vi "MC_7_25_12a_JW.vi"() -> ()   [LabVIEW 2011]
uses:
  <vilib>/Utility/file.llb/Read From Spreadsheet File (string).vi
  <vilib>/Utility/inputDevices.llb/keyboardAcquire.vi
  <vilib>/Utility/file.llb/Write To Spreadsheet File (DBL).vi
  <vilib>/Utility/file.llb/Write To Spreadsheet File (string).vi
  <vilib>/regexp/Match Regular Expression.xnode
panel:
  in  "Room Temp":dbl=294.0
  out "No Image 2":path=path "\\\\acad1\\physics/Jurchescu-group/JW-PD/Image Not Found.png"
  out "Save1 Array":string[][](array[string])
  out "XY Graph-Lin":cluster{dbl[], dbl[]}[](graph)
  out "Lin Vd":dbl
  out "Lin-Vg Array-Used":dbl[](array[numeric])
  out "Lin Id-Used":dbl[](array[numeric])
  out "Comments":string
  out "Folder Index":dbl caption="Length"
  out "Current \nRecord":string[](array[string])
  out "Transformer \nHeaders":string[](array[string])
  out "Current Device ID":string
  out "Column":string
  out "Row":string
  out "Rec: Concentration":dbl
  out "Rec: Solvent":string
  out "Rec: Method":string
  in  "?":T1(tab)
  out "Rec: Material":string
  in  "Treatment Concentration (mM):":dbl=30.0
  in  "Surface Treatment:":string
  in  "# Drops*:":dbl=inf
  in  "Solution Temp (C):":dbl=55.0
  in  "Relative Humidity (%):":dbl=nan
  in  "Room Temp (F):":dbl=nan
  in  "Time (s):":dbl=80.0
  out "Accel (RPM/s):":dbl
  in  "RPM:":dbl=1000.0
  in  "Wait Time (s):":dbl=10.0
  in  "Sample #:":dbl=1.0
  in  "Fabricator:":string="Jeremy"
  in  "Data File":path
  out "Data Folder":path
  in  "Image Folder":path
  out "Image File":path=path "D:/UserData/Desktop/Jeremy/WFU/Research/Programs/VI mods/Image Not Found.png"
  in  "Ramp (s):":dbl=3.0
  out "Calc: Off I-Sat":dbl caption="Off I-Sat" format="%#_4e"
  in  "Manuel-Dielectric":bool
  in  "Manuel-Length":bool
  out "Calc: VT-Lin":dbl
  out "New: VT-Lin":dbl
  out "Rec: VT-Lin":dbl caption="VT-Lin" format="%#_3g"
  out "Calc: Trap Density-STS":dbl format="%#_3e"
  out "New: Trap Density-STS":dbl format="%#_3e"
  out "Rec: Trap Density-STS":dbl caption="N-Sat (STS)" format="%#_3e"
  out "Calc: Trap Density-VT":dbl format="%#_3e"
  out "New: Trap Density-VT":dbl format="%#_3e"
  out "Rec: Trap Density-VT":dbl caption="N-Sat (VT)" format="%#_3e"
  out "Calc: Mobility-Lin":dbl format="%#_4e"
  out "New: Mobility-Lin":dbl format="%#_4e"
  out "Rec: Mobility-Lin":dbl caption="Mobility-Lin" format="%#_4e"
  out "Calc: Mobility-Sat":dbl format="%#_4e"
  out "Rec: Length":dbl caption="Length" format="%#_3g"
  out "Rec: Width":dbl caption="Width" format="%#_4g"
  out "Rec: Dielectric (d)":dbl caption="Dielectric (d)" format="%#_3g"
  out "XY Graph":cluster{dbl[], dbl[]}[](graph)
  in  "NumPts":dbl=5.0
  in  "Cancel Button":bool
  in  "Next Button":bool
  in  "Previous Button":bool
  in  "Up Button":bool
  in  "Down Button":bool
  out "Data Name:":string
  in  "Save Changes?":bool
  in  "New: Dielectric":dbl
  in  "New: Length":dbl
  in  "New: Width":dbl
  out "New: Mobility-Sat":dbl format="%#_4e"
  in  "Slide":dbl(slide) step=1.0 scale=-14.3..89.0 scale format="%#_1p"
  in  "Blank Button":bool
  in  "Zoom":i16(slide)=-3 scale=-5.0..5.0
  out "Image Out 2":T2(plugin-control)
  out "Image Out":T2(plugin-control)
  in  "Magnification":u16(ring) items=["5x", "10x", "20x", "50x", "80x"]
  out "Total Width":dbl
  out "Distances":dbl[](array[numeric])
  in  "Undo Button":bool
  in  "Remove Button":bool
  out "Rec: Mobility-Sat":dbl caption="Mobility-Sat" format="%#_4e"
  out "Index":string
  out "Image Name":string
  in  "Export":bool
  out "Calc: VT-Sat":dbl format="%#_3g"
  out "New: VT-Sat":dbl format="%#_3g"
  in  "Manual-Width":bool caption="Manual"
  out "XY Graph 2":cluster{dbl[], dbl[]}[](graph)
  in  "Next Button 2":bool
  in  "Previous Button 2":bool
  in  "Slide 2":dbl(slide) step=1.0 scale=-1.0..82.0 scale format="%#_1p"
  out "Calc: STS":dbl format="%#_3g"
  out "New: STS":dbl format="%#_3g"
  in  "NumPts 2":dbl=5.0 caption="NumPts"
  out "Rec: VT-Sat":dbl caption="VT-Sat" format="%#_3g"
  out "Rec: STS":dbl caption="STS-Sat" format="%#_3g"
  out "Rec: On/Off":dbl caption="On/Off-Sat" format="%#_4e"
  in  "Save Changes? 2":bool
  in  "Save Changes? 3":bool
  out "Date Recorded":string="Date Recorded" caption="Measured"
  out "Date Created":string caption="Fabricated"
  out "Rec: Temp":dbl caption="Sample Temp"
  out "New: Temp":dbl
  out "Rec: Off I-Sat":dbl caption="Off I-Sat" format="%#_4e"
  out "String":string
  in  "No Image":path=path "\\\\acad1\\physics/Jurchescu-group/JW-PD/Image Not Found.png"
  in  "Project":path=path "\\\\acad1\\physics/Jurchescu-group/JW-PD/Group Library/Origin Project Files/DeviceData_7_25a_JWW.opj"
  out "Index 2":dbl
  out "Sat Id-Log-Used":dbl[](array[numeric])
  out "Vg Array-Log-Used":dbl[](array[numeric])
  out "ROI Descriptor out":T3 {"Contours"."Type" items=["No Selection", "Point", "Line", "Rectangle", "Oval", "Polygon", "Freehand Region", "Annulus", "Unused2", "Unused3", "Broken Line", "Freehand Line", "Rotated Rectangle"]}
  out "ROI Descriptor":T3 {"Contours"."Type" items=["No Selection", "Point", "Line", "Rectangle", "Oval", "Polygon", "Freehand Region", "Annulus", "Unused2", "Unused3", "Broken Line", "Freehand Line", "Rotated Rectangle"]}
  out "Numeric 3":dbl
  out "Array 6":dbl[][](array[numeric])
  out "Cluster":T4
  out "Array 5":dbl[](array[numeric])
  out "Array 4":dbl[](array[numeric])
  out "Array 3":dbl[](array[numeric])
  out "Numeric 2":dbl
  out "Numeric":dbl
  out "Sat Id-Used":dbl[](array[numeric])
  out "Sat Vg Array-Used":dbl[](array[numeric])
  out "MobVi Index":dbl
  in  "Row Start":dbl=20.0
  # "Data Locations"
  # "Data Location"
  # "Image Location"
  # "Sample Properties"
  # "*     Inf = Full coverage\n   NaN = Unknown or Not Applicable"
  # "Recorded"
  # "Calculated"
  # "Re-Calculated"
  # "Manual"
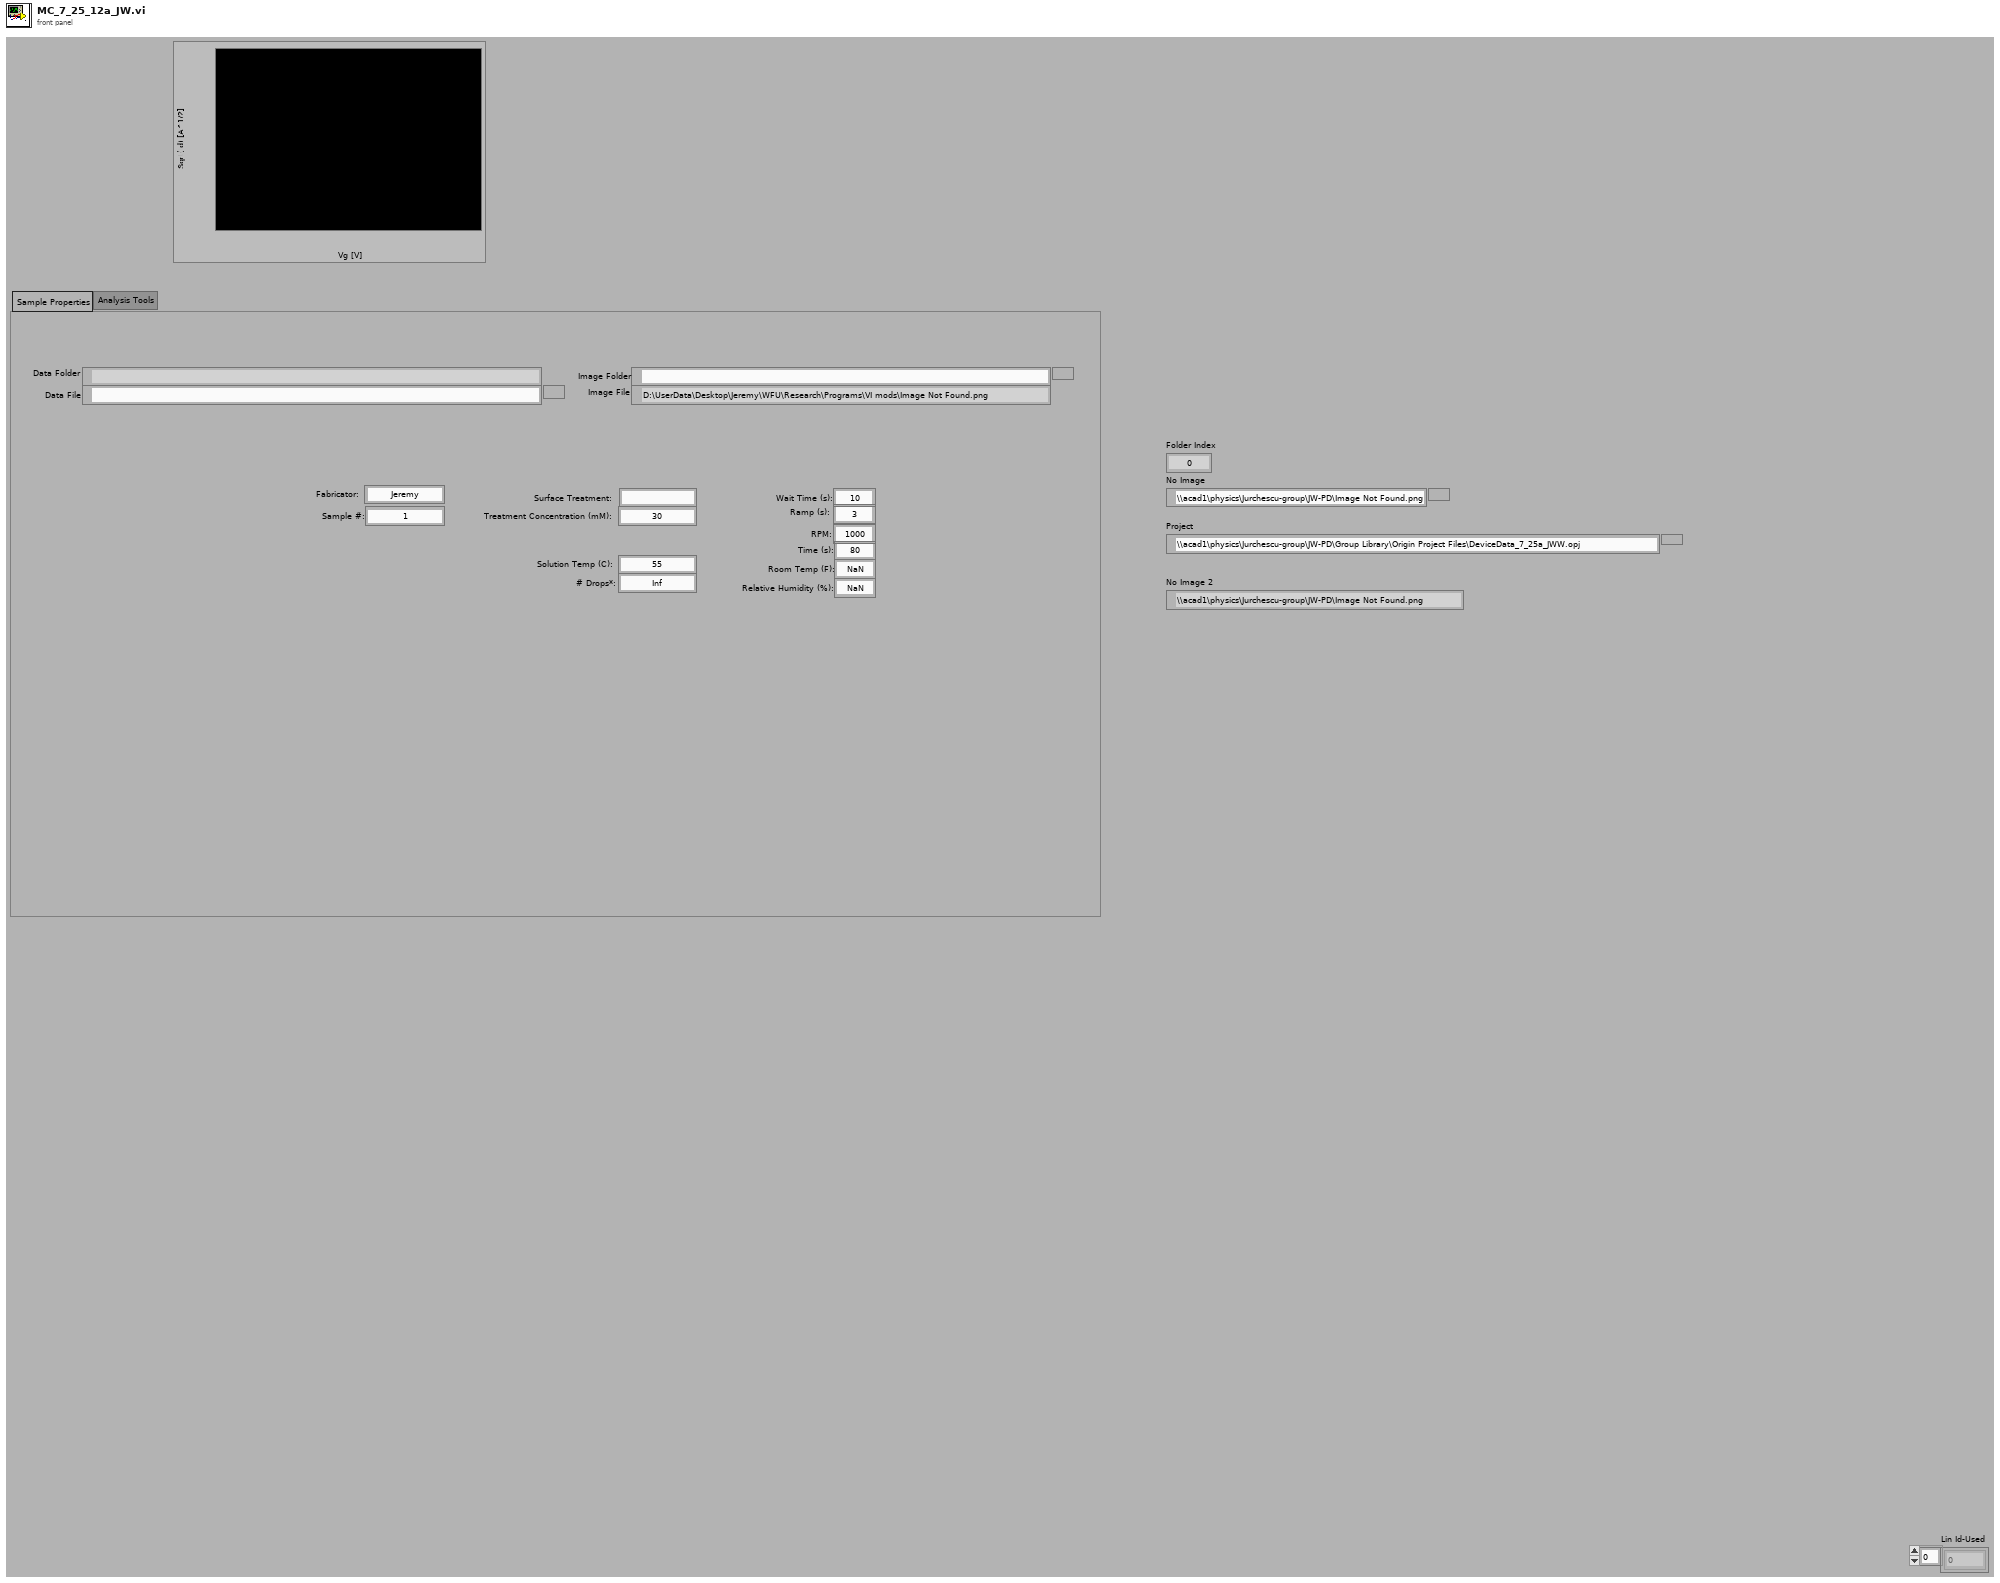
[diagram p1: front panel]
types:
  T1 = enum32{"Sample Properties", "Analysis Tools", "Current Database"}
  T2 = typedef "IMAQ Image.ctl" = refnum<image>
  T3 = typedef "ROI Descriptor" = cluster{"Global Rectangle":i32[], "Contours":cluster{"ID":enum32{"External", "Internal"}, "Type":u32, "Coordinates":i32[]}[]}
  T4 = cluster{"Numeric":dbl, "Numeric 2":dbl, "Numeric 3":dbl, "Numeric 4":dbl}
  T5 = cluster{"Mobility-Sat":dbl, "Moblitity-Lin":dbl, "On/Off":dbl, "Off Current":dbl, "Vt-Sat":dbl, "STS":dbl, "Trap Density-VT":dbl, "Trap Density-STS":dbl}
  T6 = cluster{"Date Recorded":string, "Index":string, "Length":dbl, "Width":dbl, "Sample Temp":dbl}
  T7 = cluster{"Date Created":string, "Material":string, "Solvent":string, "Concentration":dbl, "Method":string, "Dielectric (nm)":dbl, "Treatment":string, "Comments":string}
  T8 = cluster{"Mobility-Sat":dbl, "Vt-Sat":dbl, "Mobility-Lin":dbl, "Vt-Lin":dbl, "Off I-Sat":dbl, "On/Off I-Sat":dbl}
  T9 = cluster{"[0]":cluster{dbl[], dbl[]}, "[1]":cluster{dbl[], dbl[]}, "[2]":cluster{dbl[], dbl[]}, "[3]":cluster{dbl[], dbl[]}, "[4]":cluster{dbl[], dbl[]}, "[5]":cluster{dbl[], dbl[]}, "[6]":cluster{dbl[], dbl[]}, "[7]":cluster{dbl[], dbl[]}, "[8]":cluster{dbl[], dbl[]}}
  T10 = cluster{"Global Rectangle":i32[], "Contours":cluster{"Contour Type":u32, "ROI Type":u32, "Points":i32[]}[]}
  T11 = typedef "LVBoundsTypeDef.ctl" = cluster{"Width":u32, "Height":u32}
  T12 = enum16{"0", "1", "2", "3", "4", "5", "6", "7", "8", "9", "A", "B", "C", "D", "E", "F", "G", "H", "I", "J", "K", "L", "M", "N", "O", "P", "Q", "R", "S", "T", "U", "V", "W", "X", "Y", "Z", "F1", "F2", "F3", "F4", "F5", "F6", "F7", "F8", "F9", "F10", "F11", "F12", "F13", "F14", "F15", "ADD", "BACK", "BACKSLASH", "CAPITAL", "COMMA", "DECIMAL", "DELETE", "DIVIDE", "DOWN", "END", "EQUALS", "ESCAPE", "GRAVE (`)", "HOME", "INSERT", "LBRACKET", "LCONTROL", "LEFT", "L ALT", "LSHIFT", "LWIN", "MINUS", "MULTIPLY", "NEXT", "NUMLOCK", "NUMPAD_0", "NUMPAD_1", "NUMPAD_2", "NUMPAD_3", "NUMPAD_4", "NUMPAD_5", "NUMPAD_6", "NUMPAD_7", "NUMPAD_8", "NUMPAD_9", "PAUSE", "PERIOD", "PRIOR (PG UP)", "RBRACKET", "RCONTROL", "RETURN", "RIGHT", "R ALT", "RSHIFT", "RWIN", "SCROLL", "SEMICOLON", "SLASH", "SPACE", "SUBTRACT", "TAB", "UP", "ENTER (num pad)", "' (quote)"}[]
  T13 = enum16{"0", "1", "2", "3", "4", "5", "6", "7", "8", "9", "A", "B", "C", "D", "E", "F", "G", "H", "I", "J", "K", "L", "M", "N", "O", "P", "Q", "R", "S", "T", "U", "V", "W", "X", "Y", "Z", "F1", "F2", "F3", "F4", "F5", "F6", "F7", "F8", "F9", "F10", "F11", "F12", "F13", "F14", "F15", "ADD", "BACK", "BACKSLASH", "CAPITAL", "COMMA", "DECIMAL", "DELETE", "DIVIDE", "DOWN", "END", "EQUALS", "ESCAPE", "GRAVE (`)", "HOME", "INSERT", "LBRACKET", "LCONTROL", "LEFT", "L ALT", "LSHIFT", "LWIN", "MINUS", "MULTIPLY", "NEXT", "NUMLOCK", "NUMPAD_0", "NUMPAD_1", "NUMPAD_2", "NUMPAD_3", "NUMPAD_4", "NUMPAD_5", "NUMPAD_6", "NUMPAD_7", "NUMPAD_8", "NUMPAD_9", "PAUSE", "PERIOD", "PRIOR (PG UP)", "RBRACKET", "RCONTROL", "RETURN", "RIGHT", "R ALT", "RSHIFT", "RWIN", "SCROLL", "SEMICOLON", "SLASH", "SPACE", "SUBTRACT", "TAB", "UP", "ENTER (num pad)", "' (quote)"}
  T14 = cluster{"Contour Type":u32, "ROI Type":u32, "Points":i32[]}[]
  T15 = cluster{i32[], cluster{"Contour Type":u32, "ROI Type":u32, "Points":i32[]}[]}
  T16 = cluster{string, sgl, bool, bool, bool, bool, bool, bool, i32}
  T17 = cluster{i32, cluster{string, sgl, bool, bool, bool, bool, bool, bool, i32}, i32, i32}
  T18 = cluster{"Contour Type":u32, "ROI Type":u32, "Points":i32[]}
  T19 = cluster{"Points[0]":i32, "Points[1]":i32, "Points[2]":i32, "Points[3]":i32, "Points[4]":i32, "Points[5]":i32, "Points[6]":i32, "Points[7]":i32, "Points[8]":i32}
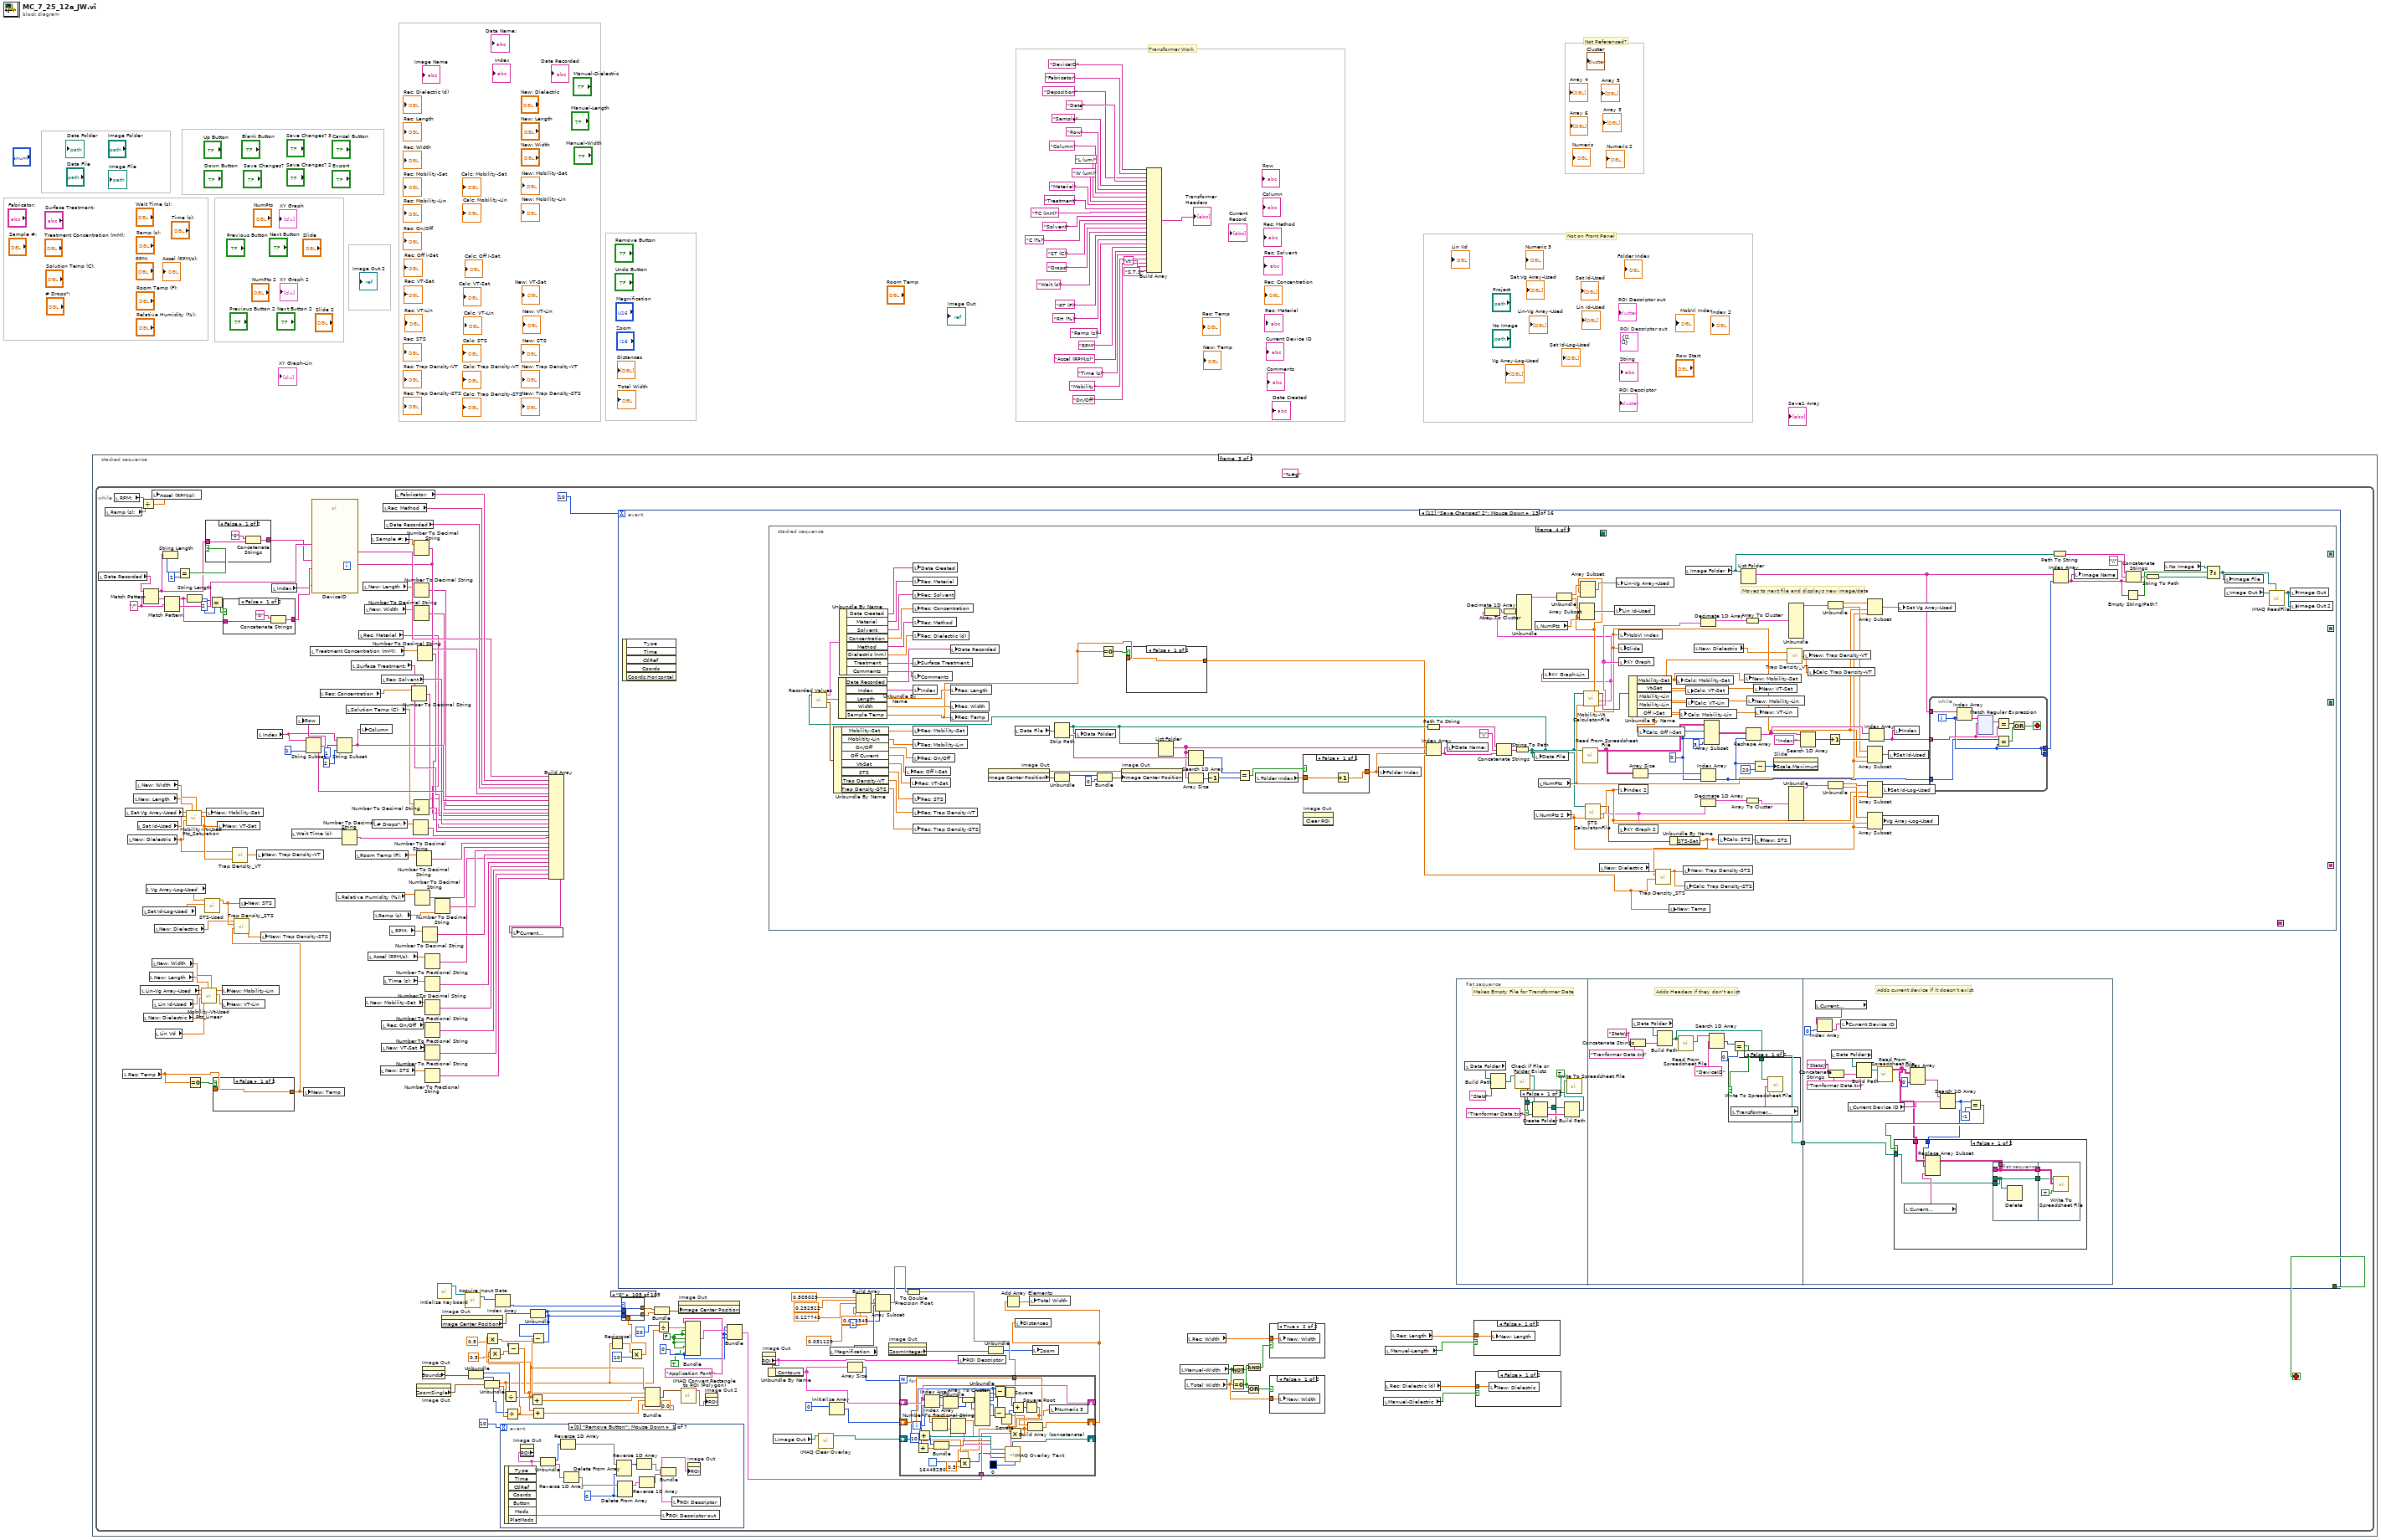
[diagram p0: block diagram]
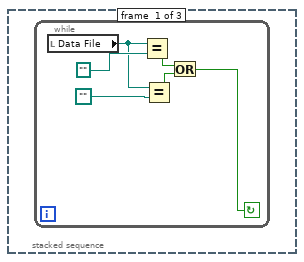
[diagram p2: hidden frame]
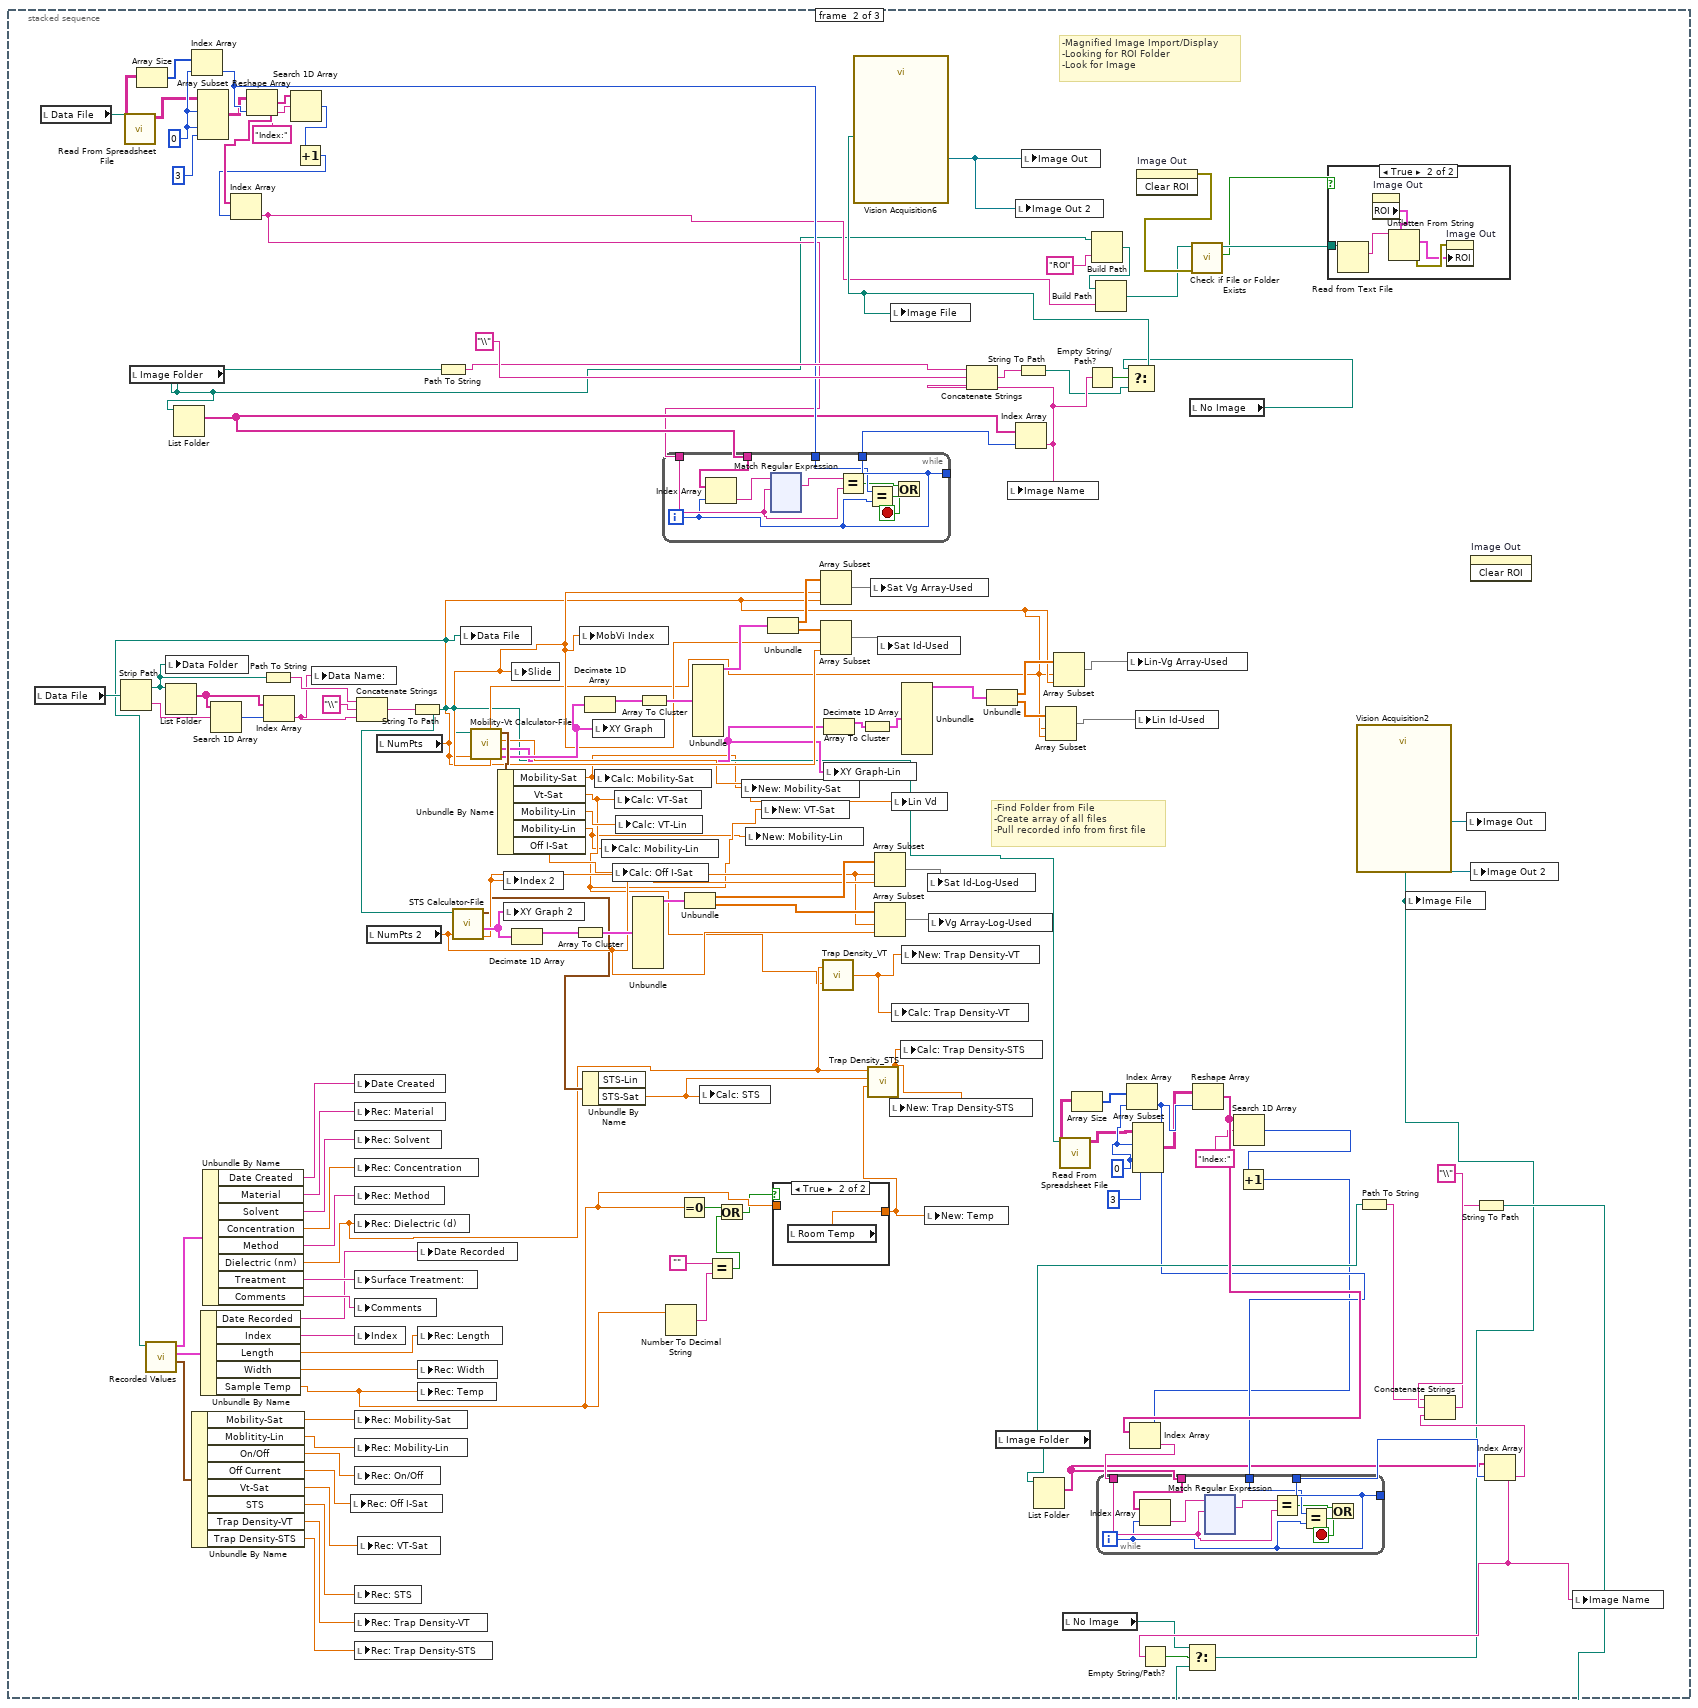
[diagram p3: hidden frame]
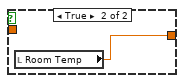
[diagram p6: hidden frame]
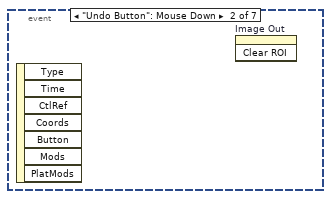
[diagram p13: hidden frame]
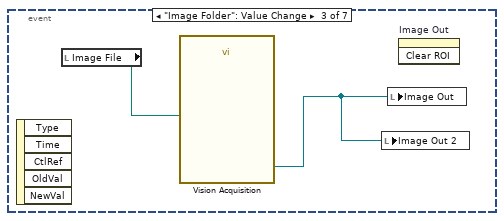
[diagram p14: hidden frame]
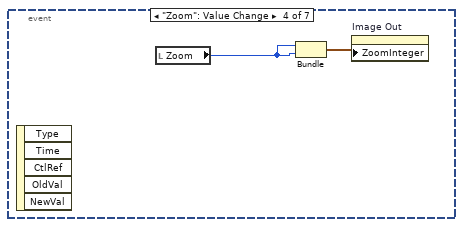
[diagram p15: hidden frame]
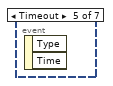
[diagram p16: hidden frame]
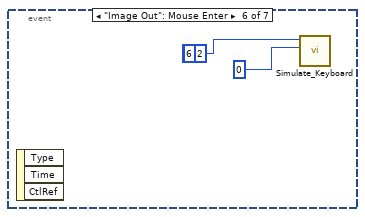
[diagram p17: hidden frame]
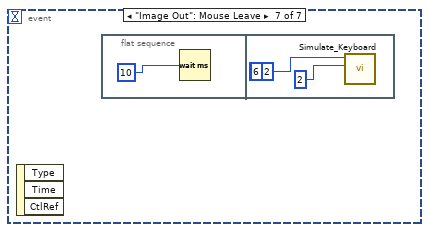
[diagram p18: hidden frame]
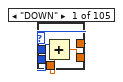
[diagram p19: hidden frame]
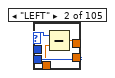
[diagram p20: hidden frame]
diagram:
  (unwired) T3 {"Global Rectangle"=[], "Contours"=[]}  # ROI Descriptor out
  # "Not Referenced?"
  # "Transformer Work"
  # "Not on Front Panel"
  n1 = stacked-sequence {
    frame #0 {
      n2 = while {
        stop <- w29 continue-if-true
        n3 = local read "Data File"() -> (w31:path)
        n4 = Equal?(x=w31, y=path "") -> (x = y?=w33:bool)
        n5 = Equal?(x=w31, y=path "") -> (x = y?=w32:bool)
        n6 = Or(x=w33, y=w32) -> (x .or. y?=w29:bool)
      }
    }
    frame #1 {
      w132 = 0
      w156 = 0
      # "-Find Folder from File\n-Create array of all files\n-Pull recorded info from first file"
      # "-Magnified Image Import/Display\n-Looking for ROI Folder\n-Look for Image"
      n7 = local read "Data File"() -> (w136:path)
      n8 = local read "Data File"() -> (w151:path)
      n9 = Strip Path(path=w136) -> (stripped path=w137:path, name=w123:string)
      n10 = call-poly <vilib>:"Read From Spreadsheet File.vi"("file path (dialog if empty)"=w151) -> ("all rows"=w154:string[][])  [unwired: 6 in, 4 out]
      n11 = local read "Image Folder"() -> (w93:path)
      n12 = Array Size(array=w154) -> (size(s)=w155:i32[])
      n13 = local write "Data Folder"(w137) -> ()
      n14 = List Folder(path=w137) -> (filenames=w127:string[])  [unwired: 3 in, 3 out]
      n15 = List Folder(path=w93) -> (filenames=w160:string[])  [unwired: 3 in, 3 out]
      n16 = Index Array(array=w155, index=w156) -> (element=w162:i32)
      n17 = Array Subset(array=w154, index (row)=w156, index (col)=w156, length (col)=3) -> (w153:string[][])  [unwired: 1 in]
      n18 = Search 1D Array(1D array=w127, element=w123) -> (index of element=w126:i32)  [unwired: 1 in]
      n19 = Reshape Array(w153, w162) -> (w167:string[])
      n20 = Path To String(path=w137) -> (string=w122:string)
      n21 = Index Array(array=w127, index=w126) -> (element=w92:string)
      n22 = Search 1D Array(1D array=w167, element="Index:") -> (index of element=w159:i32)  [unwired: 1 in]
      n23 = Increment(x=w159) -> (x+1=w158:i32)
      n24 = Index Array(array=w167, index=w158) -> (element=w94:string)
      n25 = local write "Data Name:"(w92) -> ()
      n26 = Concatenate Strings(w122, "\\", w92) -> (w124:string)
      n27 = local read "NumPts 2"() -> (w66:dbl)
      n28 = local read "NumPts"() -> (w57:dbl)
      n29 = String To Path(string=w124) -> (path=w50:path)
      n30 = call "Recorded Values.vi"("Path"=w50) -> ("Recorded Char"=w90:T5, "Recorded Prop"=w89:T6, "Fabrication Prop"=w91:T7)  [unwired: 8 in]
      n31 = Unbundle By Name(w90) -> ("Mobility-Sat"=w78:dbl, "Moblitity-Lin"=w77:dbl, "On/Off"=w76:dbl, "Off Current"=w75:dbl, "Vt-Sat"=w35:dbl, "STS"=w74:dbl, "Trap Density-VT"=w73:dbl, "Trap Density-STS"=w72:dbl)
      n32 = Unbundle By Name(w89) -> ("Date Recorded"=w82:string, "Index"=w81:string, "Length"=w80:dbl, "Width"=w79:dbl, "Sample Temp"=w41:dbl)
      n33 = Unbundle By Name(w91) -> ("Date Created"=w71:string, "Material"=w88:string, "Solvent"=w87:string, "Concentration"=w86:dbl, "Method"=w85:string, "Dielectric (nm)"=w46:dbl, "Treatment"=w84:string, "Comments"=w83:string)
      n34 = local write "Rec: Off I-Sat"(w75) -> ()
      n35 = local write "Date Created"(w71) -> ()
      n36 = local write "Rec: Material"(w88) -> ()
      n37 = local write "Rec: Solvent"(w87) -> ()
      n38 = local write "Rec: Concentration"(w86) -> ()
      n39 = local write "Rec: Method"(w85) -> ()
      n40 = local write "Rec: Dielectric (d)"(w46) -> ()
      n41 = local write "Surface Treatment:"(w84) -> ()
      n42 = local write "Comments"(w83) -> ()
      n43 = local write "Index"(w81) -> ()
      n44 = local write "Rec: Mobility-Sat"(w78) -> ()
      n45 = local write "Rec: Mobility-Lin"(w77) -> ()
      n46 = local write "Rec: On/Off"(w76) -> ()
      n47 = local write "Rec: STS"(w74) -> ()
      n48 = local write "Rec: Trap Density-VT"(w73) -> ()
      n49 = local write "Rec: Trap Density-STS"(w72) -> ()
      n50 = local write "Rec: VT-Sat"(w35) -> ()
      n51 = local write "Date Recorded"(w82) -> ()
      n52 = local write "Rec: Length"(w80) -> ()
      n53 = local write "Rec: Width"(w79) -> ()
      n54 = local write "Rec: Temp"(w41) -> ()
      n55 = Path To String(path=w93) -> (string=w164:string)
      n56 = call "STS Calculator-File.vi"("NumPts"=w66, "Path"=w50) -> ("STS Index-Sat"=w64:dbl, "XY Graph-Sat"=w65:cluster{dbl[], dbl[]}[], "Ouput"=w63:cluster{"STS-Sat":dbl, "STS-Lin":dbl})  [unwired: 5 in, 2 out]
      n57 = local write "Data File"(w50) -> ()
      n58 = call "Mobility-Vt Calculator-File.vi"("NumPts"=w57, "Path"=w50) -> ("XY Graph-Sat"=w68:cluster{dbl[], dbl[]}[], "XY Graph-Lin"=w52:cluster{dbl[], dbl[]}[], "Lin Vd"=w53:dbl, "Output"=w69:T8, "Index-Sat"=w67:dbl, "Index-Lin"=w56:dbl)  [unwired: 4 in]
      n59 = Unbundle By Name(w69) -> ("Mobility-Sat"=w45:dbl, "Vt-Sat"=w44:dbl, "Mobility-Lin"=w70:dbl, "Mobility-Lin"=w43:dbl, "Off I-Sat"=w51:dbl)
      n60 = local write "Index 2"(w64) -> ()
      n61 = local write "XY Graph 2"(w65) -> ()
      n62 = local write "Slide"(w67) -> ()
      n63 = Decimate 1D Array(w65) -> (w114:cluster{dbl[], dbl[]}[])  [unwired: 1 out]
      n64 = Array To Cluster(array=w114) -> (cluster=w116:T9)
      n65 = local write "MobVi Index"(w67) -> ()
      n66 = Unbundle By Name(w63) -> ("STS-Sat"=w49:dbl)  [unwired: 1 out]
      n67 = Decimate 1D Array(w68) -> (w150:cluster{dbl[], dbl[]}[])  [unwired: 1 out]
      n68 = local write "XY Graph"(w68) -> ()
      n69 = local write "Calc: Mobility-Sat"(w45) -> ()
      n70 = local write "Calc: Mobility-Lin"(w43) -> ()
      n71 = local write "Calc: Off I-Sat"(w51) -> ()
      n72 = local write "Calc: VT-Sat"(w44) -> ()
      n73 = local write "Calc: VT-Lin"(w70) -> ()
      n74 = Unbundle(w116) -> ("[0]"=w115:cluster{dbl[], dbl[]})  [unwired: 8 out]
      n75 = Array To Cluster(array=w150) -> (cluster=w148:T9)
      n76 = while {
        tunnel: w160 -> [w302]
        tunnel: w94 -> [w300]
        tunnel: [w299] -> _
        tunnel: [w299] -> w161
        tunnel: w162 -> [w298]
        i -> [w299]
        stop <- w295 stop-if-true
        n77 = Index Array(array=w302, index=w299) -> (element=w303:string)
        n78 = xnode "Match Regular Expression"("input string"=w303, "regular expression"=w300) -> ("whole match"=w301:string)  [unwired: 4 in, 4 out]
        n79 = Equal?(x=w301, y=w300) -> (x = y?=w297:bool)
        n80 = Equal?(x=w298, y=w299) -> (x = y?=w296:bool)
        n81 = Or(x=w297, y=w296) -> (x .or. y?=w295:bool)
      }
      n82 = Number To Decimal String(number=w41) -> (decimal integer string=w39:string)  [unwired: 1 in]
      n83 = Equal To 0?(x=w41) -> (x = 0?=w40:bool)
      n84 = Unbundle(w115) -> (w112:dbl[], w111:dbl[])
      n85 = Unbundle(w148) -> ("[0]"=w149:cluster{dbl[], dbl[]})  [unwired: 8 out]
      n86 = local write "Calc: STS"(w49) -> ()
      n87 = Equal?(x="", y=w39) -> (x = y?=w37:bool)
      n88 = Or(x=w40, y=w37) -> (x .or. y?=w36:bool)
      n89 = local write "New: Mobility-Sat"(w45) -> ()
      n90 = local write "New: Mobility-Lin"(w43) -> ()
      n91 = local write "New: VT-Sat"(w44) -> ()
      n92 = Unbundle(w149) -> (w113:dbl[], w117:dbl[])
      n93 = case shown="True" w36 {
        tunnel: [w168 w169] -> w48
        tunnel: w41 -> [w168 _]
        frame False {
        }
        frame True {
          n94 = local read "Room Temp"() -> (w169:dbl)
        }
      }
      n95 = Array Subset(array=w113, index=w67, length=w57) -> (w120:dbl[])
      n96 = Array Subset(array=w117, index=w67, length=w57) -> (w121:dbl[])
      n97 = call "Trap Density_VT.vi"("VT"=w44, "Dielectric"=w46) -> ("Trap Density-VT"=w42:dbl)
      n98 = Decimate 1D Array(w52) -> (w62:cluster{dbl[], dbl[]}[])  [unwired: 1 out]
      n99 = local write "XY Graph-Lin"(w52) -> ()
      n100 = Array To Cluster(array=w62) -> (cluster=w61:T9)
      n101 = call "Trap Density_STS.vi"("Temp (T) [K]"=w48, "S.T.S. (S)"=w49, "Dielectric"=w46) -> ("Trap Density (N)"=w47:dbl)  [unwired: 8 in]
      n102 = local write "Sat Vg Array-Used"(w120) -> ()
      n103 = Array Subset(array=w112, index=w64, length=w66) -> (w119:dbl[])
      n104 = Array Subset(array=w111, index=w64, length=w66) -> (w118:dbl[])
      n105 = local write "Sat Id-Used"(w121) -> ()
      n106 = local write "New: Trap Density-STS"(w47) -> ()
      n107 = local write "Lin Vd"(w53) -> ()
      n108 = local write "Calc: Trap Density-VT"(w42) -> ()
      n109 = local write "Calc: Trap Density-STS"(w47) -> ()
      n110 = Unbundle(w61) -> ("[0]"=w60:cluster{dbl[], dbl[]})  [unwired: 8 out]
      n111 = local write "New: Trap Density-VT"(w42) -> ()
      n112 = local write "New: Temp"(w48) -> ()
      n113 = local write "Sat Id-Log-Used"(w119) -> ()
      n114 = local write "Vg Array-Log-Used"(w118) -> ()
      n115 = Unbundle(w60) -> (w59:dbl[], w58:dbl[])
      n116 = local read "Image Folder"() -> (w143:path)
      n117 = Index Array(array=w160, index=w161) -> (element=w110:string)
      n118 = Concatenate Strings(w164, "\\", w110) -> (w165:string)
      n119 = local write "Image Name"(w110) -> ()
      n120 = String To Path(string=w165) -> (path=w108:path)
      n121 = List Folder(path=w143) -> (filenames=w139:string[])  [unwired: 3 in, 3 out]
      n122 = Array Subset(array=w58, index=w56, length=w57) -> (w54:dbl[])
      n123 = Array Subset(array=w59, index=w56, length=w57) -> (w55:dbl[])
      n124 = call-poly <vilib>:"Read From Spreadsheet File.vi"("file path (dialog if empty)"=w50) -> ("all rows"=w130:string[][])  [unwired: 6 in, 4 out]
      n125 = local read "No Image"() -> (w102:path)
      n126 = Array Size(array=w130) -> (size(s)=w131:i32[])
      n127 = Empty String/Path?(string/path=w110) -> (empty?=w109:bool)
      n128 = Build Path(base path=w93, name or relative path="ROI") -> (appended path=w96:path)
      n129 = Build Path(base path=w96, name or relative path=w94) -> (appended path=w95:path)
      n130 = Index Array(array=w131, index=w132) -> (element=w142:i32)
      n131 = local write "Lin-Vg Array-Used"(w55) -> ()
      n132 = Array Subset(array=w130, index (row)=w132, index (col)=w132, length (col)=3) -> (w129:string[][])  [unwired: 1 in]
      n133 = local write "Lin Id-Used"(w54) -> ()
      n134 = invoke on="Image Out" class="ImageControl" method="Clear ROI"() -> (error out=w100:errorcluster)  [unwired: 3 in, 2 out]
      n135 = local read "No Image"() -> (w101:path)
      n136 = Select(t=w101, s=w109, f=w108) -> (s? t:f=w107:path)
      n137 = call "Vision Acquisition6"("Image Path"=w107) -> ("Image Out"=w163:T2)  [unwired: 25 in, 1 out]
      n138 = local write "Image File"(w107) -> ()
      n139 = local write "Image Out 2"(w163) -> ()
      n140 = local write "Image Out"(w163) -> ()
      n141 = call <vilib>:"Check if File or Folder Exists.vi"("error in (no error)"=w100, "path"=w95) -> ("file or folder exists?"=w98:bool, "dup path"=w99:path)  [unwired: 7 in, 1 out]
      n142 = Reshape Array(w129, w142) -> (w147:string[])
      n143 = Search 1D Array(1D array=w147, element="Index:") -> (index of element=w135:i32)  [unwired: 1 in]
      n144 = Increment(x=w135) -> (x+1=w134:i32)
      n145 = Index Array(array=w147, index=w134) -> (element=w140:string)
      n146 = while {
        tunnel: w139 -> [w182]
        tunnel: w140 -> [w180]
        tunnel: [w179] -> _
        tunnel: [w179] -> w141
        tunnel: w142 -> [w178]
        i -> [w179]
        stop <- w175 stop-if-true
        n147 = Index Array(array=w182, index=w179) -> (element=w183:string)
        n148 = xnode "Match Regular Expression"("input string"=w183, "regular expression"=w180) -> ("whole match"=w181:string)  [unwired: 4 in, 4 out]
        n149 = Equal?(x=w181, y=w180) -> (x = y?=w177:bool)
        n150 = Equal?(x=w178, y=w179) -> (x = y?=w176:bool)
        n151 = Or(x=w177, y=w176) -> (x .or. y?=w175:bool)
      }
      n152 = case shown="True" w98 {
        tunnel: w99 -> [_ w170]
        frame False {
        }
        frame True {
          n153 = Read from Text File(file (use dialog)=w170) -> (text=w174:string)  [unwired: 3 in, 3 out]
          n154 = property on="Image Out" class="ImageControl"() -> ("ROI"=w171:T10)  [unwired: 2 in, 2 out]
          n155 = Unflatten From String(type=w171, binary string=w174) -> (value=w172:T10, error out=w173:errorcluster)  [unwired: 3 in, 1 out]
          n156 = property on="Image Out" class="ImageControl"(error in=w173, "ROI"=w172) -> ()  [unwired: 1 in, 2 out]
        }
      }
      n157 = Path To String(path=w143) -> (string=w144:string)
      n158 = invoke on="Image Out" class="ImageControl" method="Clear ROI"() -> ()  [unwired: 3 in, 3 out]
      n159 = Index Array(array=w139, index=w141) -> (element=w105:string)
      n160 = Empty String/Path?(string/path=w105) -> (empty?=w106:bool)
      n161 = Concatenate Strings(w144, "\\", w105) -> (w145:string)
      n162 = String To Path(string=w145) -> (path=w104:path)
      n163 = Select(t=w102, s=w106, f=w104) -> (s? t:f=w103:path)
      n164 = call "Vision Acquisition2"("Image Path"=w103) -> ("Image Out"=w138:T2)  [unwired: 25 in, 1 out]
      n165 = local write "Image File"(w103) -> ()
      n166 = local write "Image Out"(w138) -> ()
      n167 = local write "Image Out 2"(w138) -> ()
      n168 = local write "Image Name"(w105) -> ()
    }
    frame #2 {
      (unwired) "%#g"
      n169 = while {
        stop <- w580 stop-if-true
        w476 = "/"
        w530 = FALSE
        w528 = 0
        n170 = local read "Date Recorded"() -> (w479:string)
        n171 = local read "Ramp (s):"() -> (w446:dbl)
        n172 = local read "RPM:"() -> (w447:dbl)
        n173 = local read "Rec: Temp"() -> (w418:dbl)
        n174 = local read "Sat Vg Array-Used"() -> (w435:dbl[])
        n175 = local read "New: Dielectric"() -> (w420:dbl)
        n176 = local read "New: Length"() -> (w436:dbl)
        n177 = local read "New: Width"() -> (w438:dbl)
        n178 = local read "Sat Id-Used"() -> (w434:dbl[])
        n179 = local read "Lin-Vg Array-Used"() -> (w429:dbl[])
        n180 = Divide(x=w447, y=w446) -> (x/y=w445:dbl)
        n181 = local read "Sat Id-Log-Used"() -> (w433:dbl[])
        n182 = local read "New: Dielectric"() -> (w426:dbl)
        n183 = Match Pattern(string=w479, regular expression=w476) -> (before substring=w470:string, after substring=w477:string)  [unwired: 1 in, 2 out]
        n184 = local read "Vg Array-Log-Used"() -> (w432:dbl[])
        n185 = local read "New: Length"() -> (w428:dbl)
        n186 = local write "Accel (RPM/s):"(w445) -> ()
        n187 = local read "New: Width"() -> (w425:dbl)
        n188 = local read "Lin Id-Used"() -> (w430:dbl[])
        n189 = local read "New: Dielectric"() -> (w422:dbl)
        n190 = local read "Lin Vd"() -> (w424:dbl)
        n191 = String Length(string=w470) -> (length=w473:i32)
        n192 = Match Pattern(string=w477, regular expression=w476) -> (before substring=w464:string, after substring=w475:string)  [unwired: 1 in, 2 out]
        n193 = Equal?(x=w473, y=2) -> (x = y?=w471:bool)
        n194 = call "Mobility-Vt-Used Pts_Saturation.vi"("Width"=w438, "Length"=w436, "Dielectric (d)"=w420, "Sat Id Used"=w434, "Vg Used"=w435) -> ("Vt"=w421:dbl, "Mobility"=w437:dbl)  [unwired: 4 in, 1 out]
        n195 = String Length(string=w464) -> (length=w466:i32)
        n196 = Equal To 0?(x=w418) -> (x = 0?=w417:bool)
        n197 = call "Mobility-Vt-Used Pts_Linear.vi"("Width"=w425, "Length"=w428, "Vd"=w424, "Dielectric (d)"=w426, "Sat Id Used"=w430, "Vg Used"=w429) -> ("Vt"=w431:dbl, "Mobility"=w427:dbl)  [unwired: 3 in, 1 out]
        n198 = call "STS-Used.vi"("Id Used"=w433, "Vg-Used"=w432) -> ("STS"=w423:dbl)  [unwired: 9 in]
        n199 = case shown="False" w471 {
          tunnel: w470 -> [w590 w592]
          tunnel: [w589 w592] -> w469
          frame False {
            n200 = Concatenate Strings("0", w590) -> (w589:string)
          }
          frame True {
          }
        }
        n201 = local write "New: Mobility-Sat"(w437) -> ()
        n202 = Equal?(x=w466, y=2) -> (x = y?=w468:bool)
        n203 = case shown="False" w417 {
          tunnel: [w581 w582] -> w415
          tunnel: w418 -> [w581 _]
          frame False {
          }
          frame True {
            n204 = local read "Room Temp"() -> (w582:dbl)
          }
        }
        n205 = local write "New: VT-Sat"(w421) -> ()
        n206 = local write "New: Mobility-Lin"(w427) -> ()
        n207 = local write "New: VT-Lin"(w431) -> ()
        n208 = case shown="False" w468 {
          tunnel: w464 -> [w586 w588]
          tunnel: [w585 w588] -> w465
          frame False {
            n209 = Concatenate Strings("0", w586) -> (w585:string)
          }
          frame True {
          }
        }
        n210 = call "Trap Density_VT.vi"("VT"=w421, "Dielectric"=w420) -> ("Trap Density-VT"=w419:dbl)
        n211 = call "Trap Density_STS.vi"("Temp (T) [K]"=w415, "S.T.S. (S)"=w423, "Dielectric"=w422) -> ("Trap Density (N)"=w416:dbl)  [unwired: 8 in]
        n212 = local write "New: STS"(w423) -> ()
        n213 = local write "New: Trap Density-VT"(w419) -> ()
        n214 = local read "Index"() -> (w449:string)
        n215 = local write "New: Trap Density-STS"(w416) -> ()
        n216 = local read "Index"() -> (w463:string)
        n217 = local read "Wait Time (s):"() -> (w509:dbl)
        n218 = local write "New: Temp"(w415) -> ()
        n219 = String Subset(string=w449, length (rest)=1) -> (substring=w504:string)  [unwired: 1 in]
        n220 = local write "Row"(w504) -> ()
        n221 = local read "Treatment Concentration (mM):"() -> (w457:dbl)
        n222 = local read "Rec: Concentration"() -> (w444:dbl)
        n223 = local read "Relative Humidity (%):"() -> (w454:dbl)
        n224 = String Subset(string=w449, offset (0)=1, length (rest)=2) -> (substring=w505:string)
        n225 = Number To Decimal String(number=w509) -> (decimal integer string=w510:string)  [unwired: 1 in]
        n226 = local read "Solution Temp (C):"() -> (w498:dbl)
        n227 = local read "Surface Treatment:"() -> (w456:string)
        n228 = local read "Room Temp (F):"() -> (w502:dbl)
        n229 = local read "Rec: Material"() -> (w452:string)
        n230 = local write "Column"(w505) -> ()
        n231 = local read "New: Length"() -> (w462:dbl)
        n232 = local read "New: Width"() -> (w461:dbl)
        n233 = local read "New: Mobility-Sat"() -> (w491:dbl)
        n234 = local read "Accel (RPM/s):"() -> (w489:dbl)
        n235 = local read "Sample #:"() -> (w481:dbl)
        n236 = local read "# Drops*:"() -> (w499:dbl)
        n237 = local read "Ramp (s):"() -> (w507:dbl)
        n238 = local read "New: STS"() -> (w483:dbl)
        n239 = local read "Rec: Solvent"() -> (w458:string)
        n240 = local read "New: VT-Sat"() -> (w485:dbl)
        n241 = local read "Rec: On/Off"() -> (w487:dbl)
        n242 = local read "Rec: Method"() -> (w482:string)
        n243 = local read "Time (s):"() -> (w494:dbl)
        n244 = local read "Date Recorded"() -> (w478:string)
        n245 = local read "RPM:"() -> (w495:dbl)
        n246 = local read "Fabricator:"() -> (w503:string)
        n247 = Number To Decimal String(number=w444) -> (decimal integer string=w443:string)  [unwired: 1 in]
        n248 = Number To Decimal String(number=w499) -> (decimal integer string=w500:string)  [unwired: 1 in]
        n249 = Number To Decimal String(number=w481) -> (decimal integer string=w474:string)  [unwired: 1 in]
        n250 = call "DeviceID"("Sample"=w474, "Year"=w475, "Month"=w469, "Day"=w465, "Index"=w463) -> ("Result"=w480:string)  [unwired: 9 in, 1 out]
        n251 = Number To Decimal String(number=w462) -> (decimal integer string=w460:string)  [unwired: 1 in]
        n252 = Number To Decimal String(number=w461) -> (decimal integer string=w459:string)  [unwired: 1 in]
        n253 = Number To Decimal String(number=w498) -> (decimal integer string=w497:string)  [unwired: 1 in]
        n254 = Number To Decimal String(number=w454) -> (decimal integer string=w453:string)  [unwired: 1 in]
        n255 = Number To Decimal String(number=w502) -> (decimal integer string=w501:string)  [unwired: 1 in]
        n256 = property on="Image Out" class="ImageControl"() -> ("ZoomSingle"=w548:cluster{"X":sgl, "Y":sgl})  [unwired: 2 in, 2 out]
        n257 = Number To Decimal String(number=w457) -> (decimal integer string=w455:string)  [unwired: 1 in]
        n258 = property on="Image Out" class="ImageControl"() -> ("Bounds"=w549:T11)  [unwired: 2 in, 2 out]
        n259 = Number To Decimal String(number=w495) -> (decimal integer string=w496:string)  [unwired: 1 in]
        n260 = Number To Fractional String(number=w489) -> (F-format string=w490:string)  [unwired: 3 in]
        n261 = Number To Decimal String(number=w494) -> (decimal integer string=w493:string)  [unwired: 1 in]
        n262 = Number To Fractional String(number=w491) -> (F-format string=w492:string)  [unwired: 3 in]
        n263 = Number To Fractional String(number=w487) -> (F-format string=w488:string)  [unwired: 3 in]
        n264 = Number To Fractional String(number=w485) -> (F-format string=w486:string)  [unwired: 3 in]
        n265 = Number To Fractional String(number=w483) -> (F-format string=w484:string)  [unwired: 3 in]
        n266 = Number To Decimal String(number=w507) -> (decimal integer string=w508:string)  [unwired: 1 in]
        n267 = call <vilib>:"Intialize Keyboard.vi"() -> ("device ID"=w560:refnum<k1>)  [unwired: 10 in, 1 out]
        n268 = property on="Image Out" class="ImageControl"() -> ("Image Center Position"=w555:cluster{"X":u32, "Y":u32})  [unwired: 2 in, 2 out]
        n269 = call-poly <vilib>:"Acquire Input Data.vi"("device ID"=w560) -> ("keys pressed"=w559:T12)  [unwired: 16 in, 2 out]
        n270 = Unbundle(w549) -> ("Width"=w546:u32, "Height"=w545:u32)
        n271 = Unbundle(w548) -> ("X"=w523:sgl, "Y"=w547:sgl)
        n272 = Index Array(array=w559) -> (element=w563:T13)  [unwired: 1 in]
        n273 = event shown="[0] \"Remove Button\": Mouse Down" {
          selector: _ -> [_ _ _ _ _ _ _]
          dyn-events: _ -> [_ _ _ _ _ _ _]
          timeout: 10 -> [_ _ _ _ _ _ _]
          event "Remove Button": Mouse Down {
            w597 = 0
            n274 = event-data() -> ()  [unwired: 1 in, 7 out]
            n275 = property on="Image Out" class="ImageControl"() -> ("ROI"=w595:T10)  [unwired: 2 in, 2 out]
            n276 = Unbundle(w595) -> ("Global Rectangle"=w598:i32[], "Contours"=w600:T14)
            n277 = Reverse 1D Array(array=w598) -> (reversed array=w599:i32[])
            n278 = Reverse 1D Array(array=w600) -> (reversed array=w601:T14)
            n279 = Delete From Array(array=w599, index=w597) -> (array with subset deleted=w602:i32[])  [unwired: 1 in, 1 out]
            n280 = Delete From Array(array=w601, index=w597) -> (array with subset deleted=w603:T14)  [unwired: 1 in, 1 out]
            n281 = Reverse 1D Array(array=w602) -> (reversed array=w604:i32[])
            n282 = Reverse 1D Array(array=w603) -> (reversed array=w605:T14)
            n283 = Bundle(w604, w605) -> (w596:T15)  [unwired: 1 in]
            n284 = local write "ROI Descriptor out"(w595) -> ()
            n285 = local write "ROI Descriptor"(w596) -> ()
            n286 = property on="Image Out" class="ImageControl"("ROI"=w596) -> ()  [unwired: 2 in, 2 out]
          }
          event "Undo Button": Mouse Down {
            n287 = event-data() -> ()  [unwired: 1 in, 7 out]
            n288 = invoke on="Image Out" class="ImageControl" method="Clear ROI"() -> ()  [unwired: 3 in, 3 out]
          }
          event "Image Folder": Value Change {
            n289 = event-data() -> ()  [unwired: 1 in, 5 out]
            n290 = local read "Image File"() -> (w607:path)
            n291 = call "Vision Acquisition"("Image Path"=w607) -> ("Image Out"=w606:T2)  [unwired: 25 in, 1 out]
            n292 = local write "Image Out 2"(w606) -> ()
            n293 = local write "Image Out"(w606) -> ()
            n294 = invoke on="Image Out" class="ImageControl" method="Clear ROI"() -> ()  [unwired: 3 in, 3 out]
          }
          event "Zoom": Value Change {
            n295 = event-data() -> ()  [unwired: 1 in, 5 out]
            n296 = local read "Zoom"() -> (w608:i16)
            n297 = Bundle("Zoom"=w608, "Zoom"=w608) -> (w609:cluster{"Zoom":i16, "Zoom":i16})  [unwired: 1 in]
            n298 = property on="Image Out" class="ImageControl"("ZoomInteger"=w609) -> ()  [unwired: 2 in, 2 out]
          }
          event Timeout {
            n299 = event-data() -> ()  [unwired: 1 in, 2 out]
          }
          event "Image Out": Mouse Enter {
            (unwired) 6
            n300 = event-data() -> ()  [unwired: 1 in, 3 out]
            n301 = call "Simulate_Keyboard.vi"("Action"=0, "Virtual Key"=162) -> ()  [unwired: 7 in, 1 out]
          }
          event "Image Out": Mouse Leave {
            n302 = event-data() -> ()  [unwired: 1 in, 3 out]
            n303 = flat-sequence {
              frame #0 {
                n304 = Wait (ms)(milliseconds to wait=10) -> ()  [unwired: 1 out]
              }
              frame #1 {
                (unwired) 6
                n305 = call "Simulate_Keyboard.vi"("Action"=2, "Virtual Key"=162) -> ()  [unwired: 7 in, 1 out]
              }
            }
          }
        }
        n306 = Divide(x=w546, y=w523) -> (x/y=w536:sgl)
        n307 = Multiply(x=w536, y=0.5) -> (x*y=w542:dbl)
        n308 = Divide(x=w545, y=w547) -> (x/y=w535:sgl)
        n309 = Multiply(x=w535, y=0.5) -> (x*y=w541:dbl)
        n310 = Unbundle(w555) -> ("X"=w537:u32, "Y"=w538:u32)
        n311 = Subtract(x=w538, y=w541) -> (x-y=w539:dbl)
        n312 = Subtract(x=w537, y=w542) -> (x-y=w540:dbl)
        n313 = Add(x=w540, y=w536) -> (x+y=w554:dbl)
        n314 = Add(x=w539, y=w535) -> (x+y=w553:dbl)
        n315 = Build Array(w480, w503, w482, w478, w474, w504, w505, w460, w459, w452, w456, w455, w458, w443, w497, w500, w510, w501, w453, w508, w496, w490, w493, w492, w488, w486, w484) -> (w506:string[])
        n316 = local write "Current \nRecord"(w506) -> ()
        n317 = Reciprocal(x=w523) -> (1/x=w522:sgl)
        n318 = event shown="[12] \"Save Changes? 2\": Mouse Down" {
          selector: _ -> [_ _ _ _ _ _ _ _ _ _ _ _ _ _ _ _]
          dyn-events: _ -> [_ _ _ _ _ _ _ _ _ _ _ _ _ _ _ _]
          timeout: 10 -> [_ _ _ _ _ _ _ _ _ _ _ _ _ _ _ _]
          tunnel: [_ _ _ _ _ _ _ _ _ _ _ _ _ TRUE _ TRUE] -> w580
          event Timeout {
            n319 = event-data() -> ()  [unwired: 1 in, 2 out]
          }
          event "Down Button": Mouse Down {
            w948 = 0
            n320 = event-data() -> ()  [unwired: 1 in, 7 out]
            n321 = local read "Data File"() -> (w953:path)
            n322 = Strip Path(path=w953) -> (stripped path=w944:path, name=w962:string)
            n323 = local write "Data Folder"(w944) -> ()
            n324 = List Folder(path=w944) -> (filenames=w958:string[], error out=w898:errorcluster)  [unwired: 3 in, 2 out]
            n325 = local read "Folder Index"() -> (w900:dbl)
            n326 = property on="Image Out" class="ImageControl"() -> (error out=w901:errorcluster, "Image Center Position"=w905:cluster{"X":u32, "Y":u32})  [unwired: 2 in, 1 out]
            n327 = Array Size(array=w958) -> (size(s)=w954:i32)
            n328 = Search 1D Array(1D array=w958, element=w962) -> (index of element=w955:i32)  [unwired: 1 in]
            n329 = Decrement(x=w954) -> (x-1=w956:i32)
            n330 = Equal?(x=w955, y=w956) -> (x = y?=w957:bool)
            n331 = invoke on="Image Out" class="ImageControl" method="Clear ROI"() -> ()  [unwired: 3 in, 3 out]
            n332 = case shown="False" w957 {
              tunnel: w900 -> [w1115 _]
              tunnel: [w1114 0] -> w899
              tunnel: w898 -> [w1113 w1116]
              tunnel: [w1113 w1116] -> w897
              frame False {
                n333 = Increment(x=w1115) -> (x+1=w1114:dbl)
              }
              frame True {
              }
            }
            n334 = Unbundle(w905) -> ("X"=w903:u32)  [unwired: 1 out]
            n335 = local write "Folder Index"(w899) -> ()
            n336 = Bundle("X"=w903, 0) -> (w904:cluster{"X":u32, i32})  [unwired: 1 in]
            n337 = property on="Image Out" class="ImageControl"(error in=w901, "Image Center Position"=w904) -> ()  [unwired: 1 in, 2 out]
            n338 = Path To String(path=w944) -> (string=w963:string)
            n339 = Index Array(array=w958, index=w899) -> (element=w959:string)
            n340 = local write "Data Name:"(w959) -> ()
            n341 = Concatenate Strings(w963, "\\", w959) -> (w961:string)
            n342 = String To Path(string=w961) -> (path=w870:path)
            n343 = call "Recorded Values.vi"("Path"=w870) -> ("Recorded Char"=w965:T5, "Recorded Prop"=w966:T6, "Fabrication Prop"=w964:T7)  [unwired: 8 in]
            n344 = Unbundle By Name(w965) -> ("Mobility-Sat"=w978:dbl, "Moblitity-Lin"=w979:dbl, "On/Off"=w980:dbl, "Off Current"=w981:dbl, "Vt-Sat"=w865:dbl, "STS"=w982:dbl, "Trap Density-VT"=w983:dbl, "Trap Density-STS"=w984:dbl)
            n345 = Unbundle By Name(w964) -> ("Date Created"=w985:string, "Material"=w967:string, "Solvent"=w968:string, "Concentration"=w969:dbl, "Method"=w970:string, "Dielectric (nm)"=w971:dbl, "Treatment"=w972:string, "Comments"=w973:string)
            n346 = Unbundle By Name(w966) -> ("Date Recorded"=w974:string, "Index"=w975:string, "Length"=w976:dbl, "Width"=w977:dbl, "Sample Temp"=w867:dbl)
            n347 = local write "Date Created"(w985) -> ()
            n348 = local write "Rec: Off I-Sat"(w981) -> ()
            n349 = local write "Rec: Material"(w967) -> ()
            n350 = local write "Rec: VT-Sat"(w865) -> ()
            n351 = local write "Rec: Concentration"(w969) -> ()
            n352 = local write "Rec: Method"(w970) -> ()
            n353 = local write "Rec: Dielectric (d)"(w971) -> ()
            n354 = local write "Surface Treatment:"(w972) -> ()
            n355 = local write "Comments"(w973) -> ()
            n356 = local write "Index"(w975) -> ()
            n357 = local write "Rec: Mobility-Sat"(w978) -> ()
            n358 = local write "Rec: Mobility-Lin"(w979) -> ()
            n359 = local write "Rec: On/Off"(w980) -> ()
            n360 = local write "Rec: STS"(w982) -> ()
            n361 = local write "Rec: Trap Density-VT"(w983) -> ()
            n362 = local write "Rec: Trap Density-STS"(w984) -> ()
            n363 = local write "Rec: Solvent"(w968) -> ()
            n364 = local write "Date Recorded"(w974) -> ()
            n365 = local write "Rec: Length"(w976) -> ()
            n366 = local write "Rec: Width"(w977) -> ()
            n367 = local write "Rec: Temp"(w867) -> ()
            n368 = Equal To 0?(x=w867) -> (x = 0?=w868:bool)
            n369 = case shown="True" w868 {
              tunnel: [w986 w987] -> w866
              tunnel: w867 -> [w986 _]
              frame False {
              }
              frame True {
                n370 = local read "Room Temp"() -> (w987:dbl)
              }
            }
            n371 = local read "NumPts 2"() -> (w892:dbl)
            n372 = local read "NumPts"() -> (w896:dbl)
            n373 = local write "Data File"(w870) -> ()
            n374 = call-poly <vilib>:"Read From Spreadsheet File.vi"("file path (dialog if empty)"=w870) -> ("all rows"=w950:string[][])  [unwired: 6 in, 4 out]
            n375 = call "Mobility-Vt Calculator-File.vi"("NumPts"=w896, "Path"=w870) -> ("XY Graph-Sat"=w894:cluster{dbl[], dbl[]}[], "XY Graph-Lin"=w880:cluster{dbl[], dbl[]}[], "Output"=w895:T8, "Index-Sat"=w893:dbl, "Index-Lin"=w878:dbl)  [unwired: 4 in, 1 out]
            n376 = local read "New: Dielectric"() -> (w875:dbl)
            n377 = call "STS Calculator-File.vi"("NumPts"=w892, "Path"=w870) -> ("STS Index-Sat"=w891:dbl, "XY Graph-Sat"=w890:cluster{dbl[], dbl[]}[], "Ouput"=w889:cluster{"STS-Sat":dbl, "STS-Lin":dbl})  [unwired: 5 in, 2 out]
            n378 = Unbundle By Name(w895) -> ("Mobility-Sat"=w888:dbl, "Vt-Sat"=w874:dbl, "Mobility-Lin"=w887:dbl, "Vt-Lin"=w886:dbl, "Off I-Sat"=w871:dbl)
            n379 = Unbundle By Name(w889) -> ("STS-Sat"=w869:dbl)  [unwired: 1 out]
            n380 = local write "Index 2"(w891) -> ()
            n381 = local write "XY Graph 2"(w890) -> ()
            n382 = local write "MobVi Index"(w893) -> ()
            n383 = local write "Slide"(w893) -> ()
            n384 = local write "XY Graph"(w894) -> ()
            n385 = Array Size(array=w950) -> (size(s)=w949:i32[])
            n386 = call "Trap Density_VT.vi"("VT"=w874, "Dielectric"=w875) -> ("Trap Density-VT"=w873:dbl)
            n387 = call "Trap Density_STS.vi"("Temp (T) [K]"=w866, "S.T.S. (S)"=w869, "Dielectric"=w875) -> ("Trap Density (N)"=w872:dbl)  [unwired: 8 in]
            n388 = local write "New: STS"(w869) -> ()
            n389 = local write "Calc: Mobility-Lin"(w886) -> ()
            n390 = local write "Calc: Mobility-Sat"(w888) -> ()
            n391 = local write "Calc: STS"(w869) -> ()
            n392 = local write "Calc: VT-Sat"(w874) -> ()
            n393 = local write "Calc: Off I-Sat"(w871) -> ()
            n394 = local write "Calc: VT-Lin"(w887) -> ()
            n395 = Index Array(array=w949, index=w948) -> (element=w930:i32)
            n396 = Decimate 1D Array(w890) -> (w924:cluster{dbl[], dbl[]}[])  [unwired: 1 out]
            n397 = Decimate 1D Array(w894) -> (w934:cluster{dbl[], dbl[]}[])  [unwired: 1 out]
            n398 = Decimate 1D Array(w880) -> (w885:cluster{dbl[], dbl[]}[])  [unwired: 1 out]
            n399 = Array Subset(array=w950, index (row)=w948, index (col)=w948, length (col)=3) -> (w951:string[][])  [unwired: 1 in]
            n400 = local write "Calc: Trap Density-VT"(w873) -> ()
            n401 = local write "Calc: Trap Density-STS"(w872) -> ()
            n402 = local write "New: Trap Density-STS"(w872) -> ()
            n403 = local write "New: Trap Density-VT"(w873) -> ()
            n404 = Array To Cluster(array=w924) -> (cluster=w922:T9)
            n405 = Array To Cluster(array=w934) -> (cluster=w936:T9)
            n406 = Reshape Array(w951, w930) -> (w937:string[])
            n407 = Array To Cluster(array=w885) -> (cluster=w884:T9)
            n408 = Subtract(x=w930, y=20) -> (x-y=w929:i32)
            n409 = local write "New: Mobility-Sat"(w888) -> ()
            n410 = local write "New: Mobility-Lin"(w887) -> ()
            n411 = local write "New: VT-Sat"(w874) -> ()
            n412 = local write "New: VT-Lin"(w886) -> ()
            n413 = property on="Slide" class="Slide (strict)"("Scale.Maximum"=w929) -> ()  [unwired: 2 in, 2 out]
            n414 = Unbundle(w922) -> ("[0]"=w923:cluster{dbl[], dbl[]})  [unwired: 8 out]
            n415 = Unbundle(w936) -> ("[0]"=w935:cluster{dbl[], dbl[]})  [unwired: 8 out]
            n416 = Unbundle(w884) -> ("[0]"=w881:cluster{dbl[], dbl[]})  [unwired: 8 out]
            n417 = Search 1D Array(1D array=w937, element="Index:") -> (index of element=w945:i32)  [unwired: 1 in]
            n418 = local read "NumPts"() -> (w879:dbl)
            n419 = Unbundle(w881) -> (w883:dbl[], w882:dbl[])
            n420 = Increment(x=w945) -> (x+1=w946:i32)
            n421 = Unbundle(w923) -> (w921:dbl[], w920:dbl[])
            n422 = Unbundle(w935) -> (w926:dbl[], w925:dbl[])
            n423 = Array Subset(array=w883, index=w878, length=w879) -> (w877:dbl[])
            n424 = Array Subset(array=w882, index=w878, length=w879) -> (w876:dbl[])
            n425 = Array Subset(array=w921, index=w891, length=w892) -> (w928:dbl[])
            n426 = Array Subset(array=w920, index=w891, length=w892) -> (w927:dbl[])
            n427 = Array Subset(array=w926, index=w893, length=w896) -> (w933:dbl[])
            n428 = Array Subset(array=w925, index=w893, length=w896) -> (w932:dbl[])
            n429 = Index Array(array=w937, index=w946) -> (element=w909:string)
            n430 = local write "Lin-Vg Array-Used"(w877) -> ()
            n431 = local write "Sat Vg Array-Used"(w933) -> ()
            n432 = local write "Vg Array-Log-Used"(w927) -> ()
            n433 = local write "Lin Id-Used"(w876) -> ()
            n434 = local read "Image Folder"() -> (w907:path)
            n435 = local write "Sat Id-Used"(w932) -> ()
            n436 = local write "Sat Id-Log-Used"(w928) -> ()
            n437 = List Folder(path=w907, error in=w897) -> (filenames=w943:string[], error out=w910:errorcluster)  [unwired: 2 in, 2 out]
            n438 = while {
              tunnel: w943 -> [w1000]
              tunnel: w909 -> [w998]
              tunnel: [w997] -> _
              tunnel: [w997] -> w942
              tunnel: w930 -> [w996]
              i -> [w997]
              stop <- w993 stop-if-true
              n439 = Index Array(array=w1000, index=w997) -> (element=w1001:string)
              n440 = xnode "Match Regular Expression"("input string"=w1001, "regular expression"=w998) -> ("whole match"=w999:string)  [unwired: 4 in, 4 out]
              n441 = Equal?(x=w999, y=w998) -> (x = y?=w995:bool)
              n442 = Equal?(x=w996, y=w997) -> (x = y?=w994:bool)
              n443 = Or(x=w995, y=w994) -> (x .or. y?=w993:bool)
            }
            n444 = Build Path(base path=w907, name or relative path="ROI") -> (appended path=w906:path)
            n445 = Path To String(path=w907) -> (string=w940:string)
            n446 = Index Array(array=w943, index=w942) -> (element=w918:string)
            n447 = invoke on="Image Out" class="ImageControl" method="Clear ROI"(error in=w910) -> (error out=w913:errorcluster)  [unwired: 2 in, 2 out]
            n448 = local write "Image Name"(w918) -> ()
            n449 = Build Path(base path=w906, name or relative path=w909) -> (appended path=w914:path)
            n450 = call <vilib>:"Check if File or Folder Exists.vi"("error in (no error)"=w913, "path"=w914) -> ("file or folder exists?"=w911:bool, "dup path"=w912:path)  [unwired: 7 in, 1 out]
            n451 = Concatenate Strings(w940, "\\", w918) -> (w939:string)
            n452 = case shown="False" w911 {
              tunnel: w912 -> [_ w988]
              frame False {
              }
              frame True {
                n453 = Read from Text File(file (use dialog)=w988) -> (text=w992:string)  [unwired: 3 in, 3 out]
                n454 = property on="Image Out" class="ImageControl"() -> ("ROI"=w989:T10)  [unwired: 2 in, 2 out]
                n455 = Unflatten From String(type=w989, binary string=w992) -> (value=w990:T10, error out=w991:errorcluster)  [unwired: 3 in, 1 out]
                n456 = property on="Image Out" class="ImageControl"(error in=w991, "ROI"=w990) -> ()  [unwired: 1 in, 2 out]
              }
            }
            n457 = String To Path(string=w939) -> (path=w917:path)
            n458 = Empty String/Path?(string/path=w918) -> (empty?=w919:bool)
            n459 = local read "No Image"() -> (w915:path)
            n460 = Select(t=w915, s=w919, f=w917) -> (s? t:f=w916:path)
            n461 = local write "Image File"(w916) -> ()
            n462 = call "Vision Acquisition4"("Image Path"=w916) -> ("Image Out"=w941:T2)  [unwired: 25 in, 1 out]
            n463 = local write "Image Out"(w941) -> ()
            n464 = local write "Image Out 2"(w941) -> ()
          }
          event "Data File": Value Change {
            w1223 = 0
            n465 = event-data() -> ()  [unwired: 1 in, 5 out]
            n466 = local read "Data File"() -> (w1219:path)
            n467 = Strip Path(path=w1219) -> (stripped path=w1218:path, name=w1232:string)
            n468 = local write "Data Folder"(w1218) -> ()
            n469 = property on="Image Out" class="ImageControl"() -> (error out=w1174:errorcluster, "Image Center Position"=w1178:cluster{"X":u32, "Y":u32})  [unwired: 2 in, 1 out]
            n470 = List Folder(path=w1218) -> (filenames=w1228:string[], error out=w1184:errorcluster)  [unwired: 3 in, 2 out]
            n471 = Search 1D Array(1D array=w1228, element=w1232) -> (index of element=w1173:i32)  [unwired: 1 in]
            n472 = local write "Folder Index"(w1173) -> ()
            n473 = Unbundle(w1178) -> ("X"=w1176:u32)  [unwired: 1 out]
            n474 = Path To String(path=w1218) -> (string=w1233:string)
            n475 = Index Array(array=w1228, index=w1173) -> (element=w1229:string)
            n476 = Bundle("X"=w1176, 0) -> (w1177:cluster{"X":u32, i32})  [unwired: 1 in]
            n477 = local write "Data Name:"(w1229) -> ()
            n478 = property on="Image Out" class="ImageControl"(error in=w1174, "Image Center Position"=w1177) -> ()  [unwired: 1 in, 2 out]
            n479 = Concatenate Strings(w1233, "\\", w1229) -> (w1231:string)
            n480 = String To Path(string=w1231) -> (path=w1122:path)
            n481 = call "Recorded Values.vi"("Path"=w1122) -> ("Recorded Char"=w1171:T5, "Recorded Prop"=w1170:T6, "Fabrication Prop"=w1172:T7)  [unwired: 8 in]
            n482 = Unbundle By Name(w1171) -> ("Mobility-Sat"=w1158:dbl, "Moblitity-Lin"=w1157:dbl, "On/Off"=w1156:dbl, "Off Current"=w1155:dbl, "Vt-Sat"=w1118:dbl, "STS"=w1154:dbl, "Trap Density-VT"=w1153:dbl, "Trap Density-STS"=w1152:dbl)
            n483 = Unbundle By Name(w1172) -> ("Date Created"=w1151:string, "Material"=w1169:string, "Solvent"=w1168:string, "Concentration"=w1167:dbl, "Method"=w1166:string, "Dielectric (nm)"=w1165:dbl, "Treatment"=w1164:string, "Comments"=w1163:string)
            n484 = Unbundle By Name(w1170) -> ("Date Recorded"=w1162:string, "Index"=w1161:string, "Length"=w1160:dbl, "Width"=w1159:dbl, "Sample Temp"=w1120:dbl)
            n485 = local write "Date Created"(w1151) -> ()
            n486 = local write "Rec: Material"(w1169) -> ()
            n487 = local write "Rec: Off I-Sat"(w1155) -> ()
            n488 = local write "Rec: VT-Sat"(w1118) -> ()
            n489 = local write "Rec: Concentration"(w1167) -> ()
            n490 = local write "Rec: Method"(w1166) -> ()
            n491 = local write "Rec: Dielectric (d)"(w1165) -> ()
            n492 = local write "Surface Treatment:"(w1164) -> ()
            n493 = local write "Comments"(w1163) -> ()
            n494 = local write "Index"(w1161) -> ()
            n495 = local write "Rec: Mobility-Sat"(w1158) -> ()
            n496 = local write "Rec: Mobility-Lin"(w1157) -> ()
            n497 = local write "Rec: On/Off"(w1156) -> ()
            n498 = local write "Rec: STS"(w1154) -> ()
            n499 = local write "Rec: Trap Density-VT"(w1153) -> ()
            n500 = local write "Rec: Trap Density-STS"(w1152) -> ()
            n501 = local write "Rec: Solvent"(w1168) -> ()
            n502 = local write "Date Recorded"(w1162) -> ()
            n503 = local write "Rec: Length"(w1160) -> ()
            n504 = local write "Rec: Width"(w1159) -> ()
            n505 = local write "Rec: Temp"(w1120) -> ()
            n506 = Equal To 0?(x=w1120) -> (x = 0?=w1121:bool)
            n507 = case shown="False" w1121 {
              tunnel: [w1234 w1235] -> w1119
              tunnel: w1120 -> [w1234 _]
              frame False {
              }
              frame True {
                n508 = local read "Room Temp"() -> (w1235:dbl)
              }
            }
            n509 = local read "NumPts 2"() -> (w1146:dbl)
            n510 = local write "Data File"(w1122) -> ()
            n511 = local read "NumPts"() -> (w1147:dbl)
            n512 = call-poly <vilib>:"Read From Spreadsheet File.vi"("file path (dialog if empty)"=w1122) -> ("all rows"=w1225:string[][])  [unwired: 6 in, 4 out]
            n513 = local read "New: Dielectric"() -> (w1128:dbl)
            n514 = call "STS Calculator-File.vi"("NumPts"=w1146, "Path"=w1122) -> ("STS Index-Sat"=w1144:dbl, "XY Graph-Sat"=w1145:cluster{dbl[], dbl[]}[], "Ouput"=w1143:cluster{"STS-Sat":dbl, "STS-Lin":dbl})  [unwired: 5 in, 2 out]
            n515 = call "Mobility-Vt Calculator-File.vi"("NumPts"=w1147, "Path"=w1122) -> ("XY Graph-Sat"=w1150:cluster{dbl[], dbl[]}[], "XY Graph-Lin"=w1140:cluster{dbl[], dbl[]}[], "Output"=w1148:T8, "Index-Sat"=w1149:dbl, "Index-Lin"=w1135:dbl)  [unwired: 4 in, 1 out]
            n516 = Unbundle By Name(w1148) -> ("Mobility-Sat"=w1131:dbl, "Vt-Sat"=w1124:dbl, "Mobility-Lin"=w1130:dbl, "Mobility-Lin"=w1129:dbl, "Off I-Sat"=w1123:dbl)
            n517 = local write "Index 2"(w1144) -> ()
            n518 = local write "XY Graph 2"(w1145) -> ()
            n519 = Unbundle By Name(w1143) -> ("STS-Sat"=w1125:dbl)  [unwired: 1 out]
            n520 = local write "MobVi Index"(w1149) -> ()
            n521 = Array Size(array=w1225) -> (size(s)=w1224:i32[])
            n522 = call "Trap Density_VT.vi"("VT"=w1124, "Dielectric"=w1128) -> ("Trap Density-VT"=w1127:dbl)
            n523 = call "Trap Density_STS.vi"("Temp (T) [K]"=w1119, "S.T.S. (S)"=w1125, "Dielectric"=w1128) -> ("Trap Density (N)"=w1126:dbl)  [unwired: 8 in]
            n524 = local write "Slide"(w1149) -> ()
            n525 = local write "Calc: Mobility-Sat"(w1131) -> ()
            n526 = local write "Calc: Mobility-Lin"(w1129) -> ()
            n527 = local write "Calc: Off I-Sat"(w1123) -> ()
            n528 = local write "Calc: VT-Sat"(w1124) -> ()
            n529 = local write "Calc: VT-Lin"(w1130) -> ()
            n530 = local write "Calc: STS"(w1125) -> ()
            n531 = Decimate 1D Array(w1140) -> (w1142:cluster{dbl[], dbl[]}[])  [unwired: 1 out]
            n532 = local write "Calc: Trap Density-VT"(w1127) -> ()
            n533 = local write "Calc: Trap Density-STS"(w1126) -> ()
            n534 = local write "New: Trap Density-STS"(w1126) -> ()
            n535 = local write "New: Trap Density-VT"(w1127) -> ()
            n536 = Decimate 1D Array(w1145) -> (w1199:cluster{dbl[], dbl[]}[])  [unwired: 1 out]
            n537 = Index Array(array=w1224, index=w1223) -> (element=w1205:i32)
            n538 = Decimate 1D Array(w1150) -> (w1208:cluster{dbl[], dbl[]}[])  [unwired: 1 out]
            n539 = local write "XY Graph"(w1150) -> ()
            n540 = Array Subset(array=w1225, index (row)=w1223, index (col)=w1223, length (col)=3) -> (w1226:string[][])  [unwired: 1 in]
            n541 = Array To Cluster(array=w1142) -> (cluster=w1141:T9)
            n542 = local write "New: STS"(w1125) -> ()
            n543 = Array To Cluster(array=w1199) -> (cluster=w1197:T9)
            n544 = Array To Cluster(array=w1208) -> (cluster=w1210:T9)
            n545 = Reshape Array(w1226, w1205) -> (w1211:string[])
            n546 = local write "New: Mobility-Sat"(w1131) -> ()
            n547 = local write "New: Mobility-Lin"(w1130) -> ()
            n548 = Subtract(x=w1205, y=20) -> (x-y=w1203:i32)
            n549 = local write "New: VT-Sat"(w1124) -> ()
            n550 = local write "New: VT-Lin"(w1129) -> ()
            n551 = Unbundle(w1141) -> ("[0]"=w1139:cluster{dbl[], dbl[]})  [unwired: 8 out]
            n552 = property on="Slide" class="Slide (strict)"("Scale.Maximum"=w1203) -> ()  [unwired: 2 in, 2 out]
            n553 = local read "NumPts"() -> (w1136:dbl)
            n554 = Unbundle(w1139) -> (w1138:dbl[], w1137:dbl[])
            n555 = Unbundle(w1197) -> ("[0]"=w1198:cluster{dbl[], dbl[]})  [unwired: 8 out]
            n556 = Unbundle(w1210) -> ("[0]"=w1209:cluster{dbl[], dbl[]})  [unwired: 8 out]
            n557 = Search 1D Array(1D array=w1211, element="Index:") -> (index of element=w1220:i32)  [unwired: 1 in]
            n558 = local read "NumPts"() -> (w1132:dbl)
            n559 = Array Subset(array=w1138, index=w1135, length=w1136) -> (w1134:dbl[])
            n560 = Array Subset(array=w1137, index=w1135, length=w1136) -> (w1133:dbl[])
            n561 = Increment(x=w1220) -> (x+1=w1221:i32)
            n562 = Unbundle(w1198) -> (w1195:dbl[], w1194:dbl[])
            n563 = Unbundle(w1209) -> (w1196:dbl[], w1200:dbl[])
            n564 = local read "Image Folder"() -> (w1180:path)
            n565 = local write "Lin-Vg Array-Used"(w1134) -> ()
            n566 = Array Subset(array=w1195, index=w1144, length=w1146) -> (w1202:dbl[])
            n567 = Array Subset(array=w1194, index=w1144, length=w1146) -> (w1201:dbl[])
            n568 = Array Subset(array=w1196, index=w1149, length=w1132) -> (w1207:dbl[])
            n569 = Array Subset(array=w1200, index=w1149, length=w1132) -> (w1206:dbl[])
            n570 = Index Array(array=w1211, index=w1221) -> (element=w1182:string)
            n571 = local write "Lin Id-Used"(w1133) -> ()
            n572 = local write "Sat Vg Array-Used"(w1207) -> ()
            n573 = local write "Vg Array-Log-Used"(w1201) -> ()
            n574 = local write "Sat Id-Log-Used"(w1202) -> ()
            n575 = local write "Sat Id-Used"(w1206) -> ()
            n576 = local write "Index"(w1182) -> ()
            n577 = List Folder(path=w1180, error in=w1184) -> (filenames=w1216:string[], error out=w1183:errorcluster)  [unwired: 2 in, 2 out]
            n578 = Build Path(base path=w1180, name or relative path="ROI") -> (appended path=w1179:path)
            n579 = while {
              tunnel: w1216 -> [w1248]
              tunnel: w1182 -> [w1246]
              tunnel: [w1245] -> _
              tunnel: [w1245] -> w1215
              tunnel: w1205 -> [w1244]
              i -> [w1245]
              stop <- w1241 stop-if-true
              n580 = Index Array(array=w1248, index=w1245) -> (element=w1249:string)
              n581 = xnode "Match Regular Expression"("input string"=w1249, "regular expression"=w1246) -> ("whole match"=w1247:string)  [unwired: 4 in, 4 out]
              n582 = Equal?(x=w1247, y=w1246) -> (x = y?=w1243:bool)
              n583 = Equal?(x=w1244, y=w1245) -> (x = y?=w1242:bool)
              n584 = Or(x=w1243, y=w1242) -> (x .or. y?=w1241:bool)
            }
            n585 = invoke on="Image Out" class="ImageControl" method="Clear ROI"(error in=w1183) -> (error out=w1187:errorcluster)  [unwired: 2 in, 2 out]
            n586 = Build Path(base path=w1179, name or relative path=w1182) -> (appended path=w1188:path)
            n587 = call <vilib>:"Check if File or Folder Exists.vi"("error in (no error)"=w1187, "path"=w1188) -> ("file or folder exists?"=w1185:bool, "dup path"=w1186:path)  [unwired: 7 in, 1 out]
            n588 = case shown="True" w1185 {
              tunnel: w1186 -> [_ w1236]
              frame False {
              }
              frame True {
                n589 = Read from Text File(file (use dialog)=w1236) -> (text=w1240:string)  [unwired: 3 in, 3 out]
                n590 = property on="Image Out" class="ImageControl"() -> ("ROI"=w1237:T10)  [unwired: 2 in, 2 out]
                n591 = Unflatten From String(type=w1237, binary string=w1240) -> (value=w1238:T10, error out=w1239:errorcluster)  [unwired: 3 in, 1 out]
                n592 = property on="Image Out" class="ImageControl"(error in=w1239, "ROI"=w1238) -> ()  [unwired: 1 in, 2 out]
              }
            }
            n593 = invoke on="Image Out" class="ImageControl" method="Clear ROI"() -> ()  [unwired: 3 in, 3 out]
            n594 = Path To String(path=w1180) -> (string=w1214:string)
            n595 = Index Array(array=w1216, index=w1215) -> (element=w1192:string)
            n596 = Concatenate Strings(w1214, "\\", w1192) -> (w1213:string)
            n597 = local write "Image Name"(w1192) -> ()
            n598 = String To Path(string=w1213) -> (path=w1191:path)
            n599 = Empty String/Path?(string/path=w1192) -> (empty?=w1193:bool)
            n600 = local read "No Image"() -> (w1189:path)
            n601 = Select(t=w1189, s=w1193, f=w1191) -> (s? t:f=w1190:path)
            n602 = local write "Image File"(w1190) -> ()
            n603 = call "Vision Acquisition3"("Image Path"=w1190) -> ("Image Out"=w1217:T2)  [unwired: 25 in, 1 out]
            n604 = local write "Image Out"(w1217) -> ()
            n605 = local write "Image Out 2"(w1217) -> ()
          }
          event "Up Button": Mouse Down {
            w1467 = 0
            n606 = event-data() -> ()  [unwired: 1 in, 5 out]
            n607 = local read "Data File"() -> (w1463:path)
            n608 = Strip Path(path=w1463) -> (stripped path=w1462:path, name=w1478:string)
            n609 = local write "Data Folder"(w1462) -> ()
            n610 = List Folder(path=w1462) -> (filenames=w1472:string[], error out=w1429:errorcluster)  [unwired: 3 in, 2 out]
            n611 = Array Size(array=w1472) -> (size(s)=w1417:i32)
            n612 = Search 1D Array(1D array=w1472, element=w1478) -> (index of element=w1473:i32)  [unwired: 1 in]
            n613 = Equal To 0?(x=w1473) -> (x = 0?=w1474:bool)
            n614 = local read "Folder Index"() -> (w1416:dbl)
            n615 = property on="Image Out" class="ImageControl"() -> (error out=w1419:errorcluster, "Image Center Position"=w1423:cluster{"X":u32, "Y":u32})  [unwired: 2 in, 1 out]
            n616 = case shown="True" w1474 {
              tunnel: w1416 -> [w1608 _]
              tunnel: [w1607 w1609] -> w1415
              tunnel: w1417 -> [_ w1610]
              frame False {
                n617 = Decrement(x=w1608) -> (x-1=w1607:dbl)
              }
              frame True {
                n618 = Decrement(x=w1610) -> (x-1=w1609:i32)
              }
            }
            n619 = Unbundle(w1423) -> ("X"=w1421:u32)  [unwired: 1 out]
            n620 = local write "Folder Index"(w1415) -> ()
            n621 = Bundle("X"=w1421, 0) -> (w1422:cluster{"X":u32, i32})  [unwired: 1 in]
            n622 = Path To String(path=w1462) -> (string=w1479:string)
            n623 = Index Array(array=w1472, index=w1415) -> (element=w1475:string)
            n624 = local write "Data Name:"(w1475) -> ()
            n625 = property on="Image Out" class="ImageControl"(error in=w1419, "Image Center Position"=w1422) -> ()  [unwired: 1 in, 2 out]
            n626 = Concatenate Strings(w1479, "\\", w1475) -> (w1477:string)
            n627 = String To Path(string=w1477) -> (path=w1365:path)
            n628 = call "Recorded Values.vi"("Path"=w1365) -> ("Recorded Char"=w1413:T5, "Recorded Prop"=w1412:T6, "Fabrication Prop"=w1414:T7)  [unwired: 8 in]
            n629 = Unbundle By Name(w1413) -> ("Mobility-Sat"=w1400:dbl, "Moblitity-Lin"=w1399:dbl, "On/Off"=w1398:dbl, "Off Current"=w1397:dbl, "Vt-Sat"=w1361:dbl, "STS"=w1396:dbl, "Trap Density-VT"=w1395:dbl, "Trap Density-STS"=w1394:dbl)
            n630 = Unbundle By Name(w1414) -> ("Date Created"=w1393:string, "Material"=w1411:string, "Solvent"=w1410:string, "Concentration"=w1409:dbl, "Method"=w1408:string, "Dielectric (nm)"=w1407:dbl, "Treatment"=w1406:string, "Comments"=w1405:string)
            n631 = Unbundle By Name(w1412) -> ("Date Recorded"=w1404:string, "Index"=w1403:string, "Length"=w1402:dbl, "Width"=w1401:dbl, "Sample Temp"=w1362:dbl)
            n632 = local write "Date Created"(w1393) -> ()
            n633 = local write "Rec: Material"(w1411) -> ()
            n634 = local write "Rec: Off I-Sat"(w1397) -> ()
            n635 = local write "Rec: VT-Sat"(w1361) -> ()
            n636 = local write "Rec: Solvent"(w1410) -> ()
            n637 = local write "Rec: Concentration"(w1409) -> ()
            n638 = local write "Rec: Method"(w1408) -> ()
            n639 = local write "Rec: Dielectric (d)"(w1407) -> ()
            n640 = local write "Surface Treatment:"(w1406) -> ()
            n641 = local write "Comments"(w1405) -> ()
            n642 = local write "Index"(w1403) -> ()
            n643 = local write "Rec: Mobility-Sat"(w1400) -> ()
            n644 = local write "Rec: Mobility-Lin"(w1399) -> ()
            n645 = local write "Rec: On/Off"(w1398) -> ()
            n646 = local write "Rec: STS"(w1396) -> ()
            n647 = local write "Rec: Trap Density-VT"(w1395) -> ()
            n648 = local write "Rec: Trap Density-STS"(w1394) -> ()
            n649 = local write "Date Recorded"(w1404) -> ()
            n650 = local write "Rec: Length"(w1402) -> ()
            n651 = local write "Rec: Width"(w1401) -> ()
            n652 = local write "Rec: Temp"(w1362) -> ()
            n653 = Equal To 0?(x=w1362) -> (x = 0?=w1364:bool)
            n654 = case shown="False" w1364 {
              tunnel: [w1480 w1481] -> w1363
              tunnel: w1362 -> [w1480 _]
              frame False {
              }
              frame True {
                n655 = local read "Room Temp"() -> (w1481:dbl)
              }
            }
            n656 = local read "NumPts 2"() -> (w1388:dbl)
            n657 = local write "Data File"(w1365) -> ()
            n658 = local read "NumPts"() -> (w1392:dbl)
            n659 = local read "New: Dielectric"() -> (w1371:dbl)
            n660 = call "Mobility-Vt Calculator-File.vi"("NumPts"=w1392, "Path"=w1365) -> ("XY Graph-Sat"=w1390:cluster{dbl[], dbl[]}[], "XY Graph-Lin"=w1375:cluster{dbl[], dbl[]}[], "Output"=w1391:T8, "Index-Sat"=w1389:dbl, "Index-Lin"=w1376:dbl)  [unwired: 4 in, 1 out]
            n661 = call "STS Calculator-File.vi"("NumPts"=w1388, "Path"=w1365) -> ("STS Index-Sat"=w1387:dbl, "XY Graph-Sat"=w1386:cluster{dbl[], dbl[]}[], "Ouput"=w1385:cluster{"STS-Sat":dbl, "STS-Lin":dbl})  [unwired: 5 in, 2 out]
            n662 = call-poly <vilib>:"Read From Spreadsheet File.vi"("file path (dialog if empty)"=w1365) -> ("all rows"=w1469:string[][])  [unwired: 6 in, 4 out]
            n663 = Unbundle By Name(w1391) -> ("Mobility-Sat"=w1374:dbl, "Vt-Sat"=w1367:dbl, "Mobility-Lin"=w1373:dbl, "Mobility-Lin"=w1372:dbl, "Off I-Sat"=w1366:dbl)
            n664 = Unbundle By Name(w1385) -> ("STS-Sat"=w1368:dbl)  [unwired: 1 out]
            n665 = local write "Index 2"(w1387) -> ()
            n666 = local write "XY Graph 2"(w1386) -> ()
            n667 = local write "MobVi Index"(w1389) -> ()
            n668 = local write "Slide"(w1389) -> ()
            n669 = local write "XY Graph"(w1390) -> ()
            n670 = Array Size(array=w1469) -> (size(s)=w1468:i32[])
            n671 = local write "Calc: Mobility-Sat"(w1374) -> ()
            n672 = local write "Calc: Mobility-Lin"(w1372) -> ()
            n673 = call "Trap Density_VT.vi"("VT"=w1367, "Dielectric"=w1371) -> ("Trap Density-VT"=w1370:dbl)
            n674 = call "Trap Density_STS.vi"("Temp (T) [K]"=w1363, "S.T.S. (S)"=w1368, "Dielectric"=w1371) -> ("Trap Density (N)"=w1369:dbl)  [unwired: 8 in]
            n675 = local write "Calc: VT-Sat"(w1367) -> ()
            n676 = local write "Calc: Off I-Sat"(w1366) -> ()
            n677 = local write "Calc: VT-Lin"(w1373) -> ()
            n678 = local write "Calc: STS"(w1368) -> ()
            n679 = local write "New: STS"(w1368) -> ()
            n680 = Decimate 1D Array(w1375) -> (w1384:cluster{dbl[], dbl[]}[])  [unwired: 1 out]
            n681 = local write "Calc: Trap Density-VT"(w1370) -> ()
            n682 = local write "Calc: Trap Density-STS"(w1369) -> ()
            n683 = local write "New: Trap Density-STS"(w1369) -> ()
            n684 = local write "New: Trap Density-VT"(w1370) -> ()
            n685 = Decimate 1D Array(w1386) -> (w1446:cluster{dbl[], dbl[]}[])  [unwired: 1 out]
            n686 = Index Array(array=w1468, index=w1467) -> (element=w1452:i32)
            n687 = Decimate 1D Array(w1390) -> (w1456:cluster{dbl[], dbl[]}[])  [unwired: 1 out]
            n688 = Array To Cluster(array=w1384) -> (cluster=w1383:T9)
            n689 = Array Subset(array=w1469, index (row)=w1467, index (col)=w1467, length (col)=3) -> (w1470:string[][])  [unwired: 1 in]
            n690 = Array To Cluster(array=w1446) -> (cluster=w1444:T9)
            n691 = Array To Cluster(array=w1456) -> (cluster=w1458:T9)
            n692 = Reshape Array(w1470, w1452) -> (w1459:string[])
            n693 = Subtract(x=w1452, y=20) -> (x-y=w1451:i32)
            n694 = Unbundle(w1383) -> ("[0]"=w1380:cluster{dbl[], dbl[]})  [unwired: 8 out]
            n695 = local write "New: Mobility-Sat"(w1374) -> ()
            n696 = local write "New: Mobility-Lin"(w1373) -> ()
            n697 = local write "New: VT-Sat"(w1367) -> ()
            n698 = local write "New: VT-Lin"(w1372) -> ()
            n699 = property on="Slide" class="Slide (strict)"("Scale.Maximum"=w1451) -> ()  [unwired: 2 in, 2 out]
            n700 = Unbundle(w1444) -> ("[0]"=w1445:cluster{dbl[], dbl[]})  [unwired: 8 out]
            n701 = Unbundle(w1458) -> ("[0]"=w1457:cluster{dbl[], dbl[]})  [unwired: 8 out]
            n702 = local read "NumPts"() -> (w1377:dbl)
            n703 = Unbundle(w1380) -> (w1379:dbl[], w1378:dbl[])
            n704 = Search 1D Array(1D array=w1459, element="Index:") -> (index of element=w1464:i32)  [unwired: 1 in]
            n705 = Increment(x=w1464) -> (x+1=w1465:i32)
            n706 = Unbundle(w1445) -> (w1443:dbl[], w1442:dbl[])
            n707 = Unbundle(w1457) -> (w1450:dbl[], w1449:dbl[])
            n708 = Array Subset(array=w1379, index=w1376, length=w1377) -> (w1381:dbl[])
            n709 = Array Subset(array=w1378, index=w1376, length=w1377) -> (w1382:dbl[])
            n710 = local read "Image Folder"() -> (w1418:path)
            n711 = local write "Lin-Vg Array-Used"(w1381) -> ()
            n712 = Array Subset(array=w1443, index=w1387, length=w1388) -> (w1448:dbl[])
            n713 = Array Subset(array=w1442, index=w1387, length=w1388) -> (w1447:dbl[])
            n714 = Array Subset(array=w1450, index=w1389, length=w1392) -> (w1455:dbl[])
            n715 = Array Subset(array=w1449, index=w1389, length=w1392) -> (w1454:dbl[])
            n716 = local write "Lin Id-Used"(w1382) -> ()
            n717 = Index Array(array=w1459, index=w1465) -> (element=w1425:string)
            n718 = local write "Sat Vg Array-Used"(w1455) -> ()
            n719 = local write "Vg Array-Log-Used"(w1447) -> ()
            n720 = local write "Sat Id-Log-Used"(w1448) -> ()
            n721 = local write "Sat Id-Used"(w1454) -> ()
            n722 = local write "Index"(w1425) -> ()
            n723 = List Folder(path=w1418, error in=w1429) -> (filenames=w1461:string[], error out=w1428:errorcluster)  [unwired: 2 in, 2 out]
            n724 = Build Path(base path=w1418, name or relative path="ROI") -> (appended path=w1426:path)
            n725 = while {
              tunnel: w1461 -> [w1494]
              tunnel: w1425 -> [w1492]
              tunnel: [w1491] -> w1460
              tunnel: w1452 -> [w1490]
              i -> [w1491]
              stop <- w1487 stop-if-true
              n726 = Index Array(array=w1494, index=w1491) -> (element=w1495:string)
              n727 = xnode "Match Regular Expression"("input string"=w1495, "regular expression"=w1492) -> ("whole match"=w1493:string)  [unwired: 4 in, 4 out]
              n728 = Equal?(x=w1493, y=w1492) -> (x = y?=w1489:bool)
              n729 = Equal?(x=w1490, y=w1491) -> (x = y?=w1488:bool)
              n730 = Or(x=w1489, y=w1488) -> (x .or. y?=w1487:bool)
            }
            n731 = invoke on="Image Out" class="ImageControl" method="Clear ROI"(error in=w1428) -> (error out=w1432:errorcluster)  [unwired: 2 in, 2 out]
            n732 = Build Path(base path=w1426, name or relative path=w1425) -> (appended path=w1424:path)
            n733 = call <vilib>:"Check if File or Folder Exists.vi"("error in (no error)"=w1432, "path"=w1424) -> ("file or folder exists?"=w1430:bool, "dup path"=w1431:path)  [unwired: 7 in, 1 out]
            n734 = case shown="True" w1430 {
              tunnel: w1431 -> [_ w1482]
              frame False {
              }
              frame True {
                n735 = Read from Text File(file (use dialog)=w1482) -> (text=w1486:string)  [unwired: 3 in, 3 out]
                n736 = property on="Image Out" class="ImageControl"() -> ("ROI"=w1483:T10)  [unwired: 2 in, 2 out]
                n737 = Unflatten From String(type=w1483, binary string=w1486) -> (value=w1484:T10, error out=w1485:errorcluster)  [unwired: 3 in, 1 out]
                n738 = property on="Image Out" class="ImageControl"(error in=w1485, "ROI"=w1484) -> ()  [unwired: 1 in, 2 out]
              }
            }
            n739 = Index Array(array=w1461, index=w1460) -> (element=w1434:string)
            n740 = local write "Image Name"(w1434) -> ()
            n741 = Empty String/Path?(string/path=w1434) -> (empty?=w1441:bool)
            n742 = Build Path(base path=w1418, name or relative path=w1434) -> (appended path=w1433:path)
            n743 = local read "No Image"() -> (w1440:path)
            n744 = Select(t=w1440, s=w1441, f=w1433) -> (s? t:f=w1435:path)
            n745 = call <vilib>:"Get File Extension.vi"("file"=w1435) -> ("lowercase file extension"=w1437:string)  [unwired: 7 in, 3 out]
            n746 = local write "Image File"(w1435) -> ()
            n747 = local write "String"(w1437) -> ()
            n748 = Search 1D Array(1D array=string[] ["bmp", "jpeg", "png", "jpg", "gif"], element=w1437) -> (index of element=w1436:i32)  [unwired: 1 in]
            n749 = call "Vision Acquisition5"("Image Path"=w1435) -> ("Image Out"=w1439:T2)  [unwired: 25 in, 1 out]
            n750 = Less Than 0?(x=w1436) -> ()  [unwired: 1 out]
            n751 = local write "Image Out"(w1439) -> ()
            n752 = local write "Image Out 2"(w1439) -> ()
          }
          event "Save Changes? 3": Mouse Down {
            n753 = event-data() -> ()  [unwired: 1 in, 7 out]
            n754 = local read "Image Folder"() -> (w1611:path)
            n755 = Build Path(base path=w1611, name or relative path="ROI") -> (appended path=w1618:path)
            n756 = call <vilib>:"Check if File or Folder Exists.vi"("path"=w1618) -> ("file or folder exists?"=w1620:bool, "dup path"=w1617:path)  [unwired: 8 in, 1 out]
            n757 = case shown="False" w1620 {
              tunnel: w1617 -> [w1622 w1623]
              tunnel: [w1621 w1623] -> w1612
              frame False {
                n758 = Create Folder(path (use dialog)=w1622) -> (created path=w1621:path)  [unwired: 2 in, 2 out]
              }
              frame True {
              }
            }
            n759 = local read "Index"() -> (w1614:string)
            n760 = property on="Image Out" class="ImageControl"() -> ("ROI"=w1616:T10)  [unwired: 2 in, 2 out]
            n761 = Build Path(base path=w1612, name or relative path=w1614) -> (appended path=w1613:path)
            n762 = Flatten To String(anything=w1616) -> (data string=w1615:string)  [unwired: 3 in, 2 out]
            n763 = Write to Text File(file (use dialog)=w1613, text=w1615) -> ()  [unwired: 2 in, 3 out]
          }
          event "Next Button": Mouse Down {
            n764 = event-data() -> ()  [unwired: 1 in, 5 out]
            n765 = local read "XY Graph"() -> (w1636:cluster{dbl[], dbl[]}[])
            n766 = Decimate 1D Array(w1636) -> (w1632:cluster{dbl[], dbl[]}[], w1631:cluster{dbl[], dbl[]}[])
            n767 = Array To Cluster(array=w1632) -> (cluster=w1642:T9)
            n768 = local read "MobVi Index"() -> (w1638:dbl)
            n769 = Unbundle(w1642) -> ("[0]"=w1641:cluster{dbl[], dbl[]})  [unwired: 8 out]
            n770 = local read "NumPts"() -> (w1637:dbl)
            n771 = Unbundle(w1641) -> (w1640:dbl[], w1639:dbl[])
            n772 = Increment(x=w1638) -> (x+1=w1633:dbl)
            n773 = local read "New: Dielectric"() -> (w1627:dbl)
            n774 = local read "New: Length"() -> (w1626:dbl)
            n775 = local read "New: Width"() -> (w1625:dbl)
            n776 = local write "MobVi Index"(w1633) -> ()
            n777 = Array Subset(array=w1640, index=w1633, length=w1637) -> (w1629:dbl[])
            n778 = Array Subset(array=w1639, index=w1633, length=w1637) -> (w1628:dbl[])
            n779 = local write "Sat Vg Array-Used"(w1629) -> ()
            n780 = local write "Sat Id-Used"(w1628) -> ()
            n781 = call "Mobility-Vt-Used Pts_Saturation.vi"("Width"=w1625, "Length"=w1626, "Dielectric (d)"=w1627, "Sat Id Used"=w1628, "Vg Used"=w1629) -> ("Vt"=w1624:dbl, "Mobility"=w1630:dbl)  [unwired: 4 in, 1 out]
            n782 = Bundle(w1629, w1628) -> (w1635:cluster{dbl[], dbl[]})  [unwired: 1 in]
            n783 = Build Array (concatenate)(w1632, w1631, w1635) -> (w1634:cluster{dbl[], dbl[]}[])
            n784 = local write "New: Mobility-Sat"(w1630) -> ()
            n785 = local write "New: VT-Sat"(w1624) -> ()
            n786 = local write "XY Graph"(w1634) -> ()
          }
          event "Next Button 2": Mouse Down {
            n787 = event-data() -> ()  [unwired: 1 in, 7 out]
            n788 = local read "XY Graph 2"() -> (w1651:cluster{dbl[], dbl[]}[])
            n789 = Decimate 1D Array(w1651) -> (w1647:cluster{dbl[], dbl[]}[], w1646:cluster{dbl[], dbl[]}[])
            n790 = Array To Cluster(array=w1647) -> (cluster=w1657:T9)
            n791 = local read "Index 2"() -> (w1653:dbl)
            n792 = Unbundle(w1657) -> ("[0]"=w1656:cluster{dbl[], dbl[]})  [unwired: 8 out]
            n793 = local read "NumPts 2"() -> (w1652:dbl)
            n794 = Unbundle(w1656) -> (w1655:dbl[], w1654:dbl[])
            n795 = Increment(x=w1653) -> (x+1=w1648:dbl)
            n796 = local write "Index 2"(w1648) -> ()
            n797 = Array Subset(array=w1654, index=w1648, length=w1652) -> (w1643:dbl[])
            n798 = Array Subset(array=w1655, index=w1648, length=w1652) -> (w1644:dbl[])
            n799 = call "STS-Used.vi"("Id Used"=w1644, "Vg-Used"=w1643) -> ("STS"=w1645:dbl)  [unwired: 9 in]
            n800 = Bundle(w1644, w1643) -> (w1650:cluster{dbl[], dbl[]})  [unwired: 1 in]
            n801 = local write "Vg Array-Log-Used"(w1643) -> ()
            n802 = local write "Sat Id-Log-Used"(w1644) -> ()
            n803 = local write "New: STS"(w1645) -> ()
            n804 = Build Array (concatenate)(w1647, w1646, w1650) -> (w1649:cluster{dbl[], dbl[]}[])
            n805 = local write "XY Graph 2"(w1649) -> ()
          }
          event "Previous Button 2": Mouse Down {
            n806 = event-data() -> ()  [unwired: 1 in, 7 out]
            n807 = local read "XY Graph 2"() -> (w1667:cluster{dbl[], dbl[]}[])
            n808 = Decimate 1D Array(w1667) -> (w1664:cluster{dbl[], dbl[]}[], w1663:cluster{dbl[], dbl[]}[])
            n809 = Array To Cluster(array=w1664) -> (cluster=w1672:T9)
            n810 = local read "Index 2"() -> (w1660:dbl)
            n811 = Unbundle(w1672) -> ("[0]"=w1671:cluster{dbl[], dbl[]})  [unwired: 8 out]
            n812 = local read "NumPts 2"() -> (w1668:dbl)
            n813 = Unbundle(w1671) -> (w1670:dbl[], w1669:dbl[])
            n814 = Decrement(x=w1660) -> (x-1=w1661:dbl)
            n815 = local write "Index 2"(w1661) -> ()
            n816 = Array Subset(array=w1670, index=w1661, length=w1668) -> (w1658:dbl[])
            n817 = Array Subset(array=w1669, index=w1661, length=w1668) -> (w1659:dbl[])
            n818 = local write "Vg Array-Log-Used"(w1659) -> ()
            n819 = local write "Sat Id-Log-Used"(w1658) -> ()
            n820 = Bundle(w1658, w1659) -> (w1666:cluster{dbl[], dbl[]})  [unwired: 1 in]
            n821 = call "STS-Used.vi"("Id Used"=w1658, "Vg-Used"=w1659) -> ("STS"=w1662:dbl)  [unwired: 9 in]
            n822 = Build Array (concatenate)(w1664, w1663, w1666) -> (w1665:cluster{dbl[], dbl[]}[])
            n823 = local write "New: STS"(w1662) -> ()
            n824 = local write "XY Graph 2"(w1665) -> ()
          }
          event "Previous Button": Mouse Down {
            n825 = event-data() -> ()  [unwired: 1 in, 5 out]
            n826 = local read "XY Graph"() -> (w1686:cluster{dbl[], dbl[]}[])
            n827 = Decimate 1D Array(w1686) -> (w1683:cluster{dbl[], dbl[]}[], w1682:cluster{dbl[], dbl[]}[])
            n828 = Array To Cluster(array=w1683) -> (cluster=w1691:T9)
            n829 = local read "MobVi Index"() -> (w1681:dbl)
            n830 = Unbundle(w1691) -> ("[0]"=w1690:cluster{dbl[], dbl[]})  [unwired: 8 out]
            n831 = local read "NumPts"() -> (w1687:dbl)
            n832 = Unbundle(w1690) -> (w1689:dbl[], w1688:dbl[])
            n833 = Decrement(x=w1681) -> (x-1=w1680:dbl)
            n834 = local read "New: Dielectric"() -> (w1674:dbl)
            n835 = local read "New: Length"() -> (w1675:dbl)
            n836 = local read "New: Width"() -> (w1676:dbl)
            n837 = local write "MobVi Index"(w1680) -> ()
            n838 = Array Subset(array=w1689, index=w1680, length=w1687) -> (w1679:dbl[])
            n839 = Array Subset(array=w1688, index=w1680, length=w1687) -> (w1678:dbl[])
            n840 = local write "Sat Vg Array-Used"(w1679) -> ()
            n841 = local write "Sat Id-Used"(w1678) -> ()
            n842 = call "Mobility-Vt-Used Pts_Linear.vi"("Width"=w1676, "Length"=w1675, "Dielectric (d)"=w1674, "Sat Id Used"=w1678, "Vg Used"=w1679) -> ("Vt"=w1673:dbl, "Mobility"=w1677:dbl)  [unwired: 4 in, 1 out]
            n843 = Bundle(w1679, w1678) -> (w1685:cluster{dbl[], dbl[]})  [unwired: 1 in]
            n844 = local write "New: VT-Sat"(w1673) -> ()
            n845 = Build Array (concatenate)(w1683, w1682, w1685) -> (w1684:cluster{dbl[], dbl[]}[])
            n846 = local write "New: Mobility-Sat"(w1677) -> ()
            n847 = local write "XY Graph"(w1684) -> ()
          }
          event "Slide": Value Change {
            n848 = event-data() -> ()  [unwired: 1 in, 5 out]
            n849 = local read "XY Graph"() -> (w1704:cluster{dbl[], dbl[]}[])
            n850 = Decimate 1D Array(w1704) -> (w1701:cluster{dbl[], dbl[]}[], w1700:cluster{dbl[], dbl[]}[])
            n851 = Array To Cluster(array=w1701) -> (cluster=w1709:T9)
            n852 = Unbundle(w1709) -> ("[0]"=w1708:cluster{dbl[], dbl[]})  [unwired: 8 out]
            n853 = local read "NumPts"() -> (w1705:dbl)
            n854 = local read "Slide"() -> (w1693:dbl)
            n855 = Unbundle(w1708) -> (w1707:dbl[], w1706:dbl[])
            n856 = local read "New: Dielectric"() -> (w1694:dbl)
            n857 = local read "New: Length"() -> (w1695:dbl)
            n858 = local read "New: Width"() -> (w1696:dbl)
            n859 = local write "MobVi Index"(w1693) -> ()
            n860 = Array Subset(array=w1707, index=w1693, length=w1705) -> (w1699:dbl[])
            n861 = Array Subset(array=w1706, index=w1693, length=w1705) -> (w1698:dbl[])
            n862 = local write "Sat Vg Array-Used"(w1699) -> ()
            n863 = local write "Sat Id-Used"(w1698) -> ()
            n864 = call "Mobility-Vt-Used Pts_Linear.vi"("Width"=w1696, "Length"=w1695, "Dielectric (d)"=w1694, "Sat Id Used"=w1698, "Vg Used"=w1699) -> ("Vt"=w1692:dbl, "Mobility"=w1697:dbl)  [unwired: 4 in, 1 out]
            n865 = Bundle(w1699, w1698) -> (w1703:cluster{dbl[], dbl[]})  [unwired: 1 in]
            n866 = local write "New: VT-Sat"(w1692) -> ()
            n867 = Build Array (concatenate)(w1701, w1700, w1703) -> (w1702:cluster{dbl[], dbl[]}[])
            n868 = local write "New: Mobility-Sat"(w1697) -> ()
            n869 = local write "XY Graph"(w1702) -> ()
          }
          event "Slide 2": Value Change {
            n870 = event-data() -> ()  [unwired: 1 in, 5 out]
            n871 = local read "XY Graph 2"() -> (w1718:cluster{dbl[], dbl[]}[])
            n872 = Decimate 1D Array(w1718) -> (w1715:cluster{dbl[], dbl[]}[], w1714:cluster{dbl[], dbl[]}[])
            n873 = Array To Cluster(array=w1715) -> (cluster=w1723:T9)
            n874 = Unbundle(w1723) -> ("[0]"=w1722:cluster{dbl[], dbl[]})  [unwired: 8 out]
            n875 = local read "NumPts 2"() -> (w1719:dbl)
            n876 = local read "Slide 2"() -> (w1713:dbl)
            n877 = Unbundle(w1722) -> (w1721:dbl[], w1720:dbl[])
            n878 = local write "Index 2"(w1713) -> ()
            n879 = Array Subset(array=w1721, index=w1713, length=w1719) -> (w1711:dbl[])
            n880 = Array Subset(array=w1720, index=w1713, length=w1719) -> (w1710:dbl[])
            n881 = local write "Vg Array-Log-Used"(w1710) -> ()
            n882 = local write "Sat Id-Log-Used"(w1711) -> ()
            n883 = call "STS-Used.vi"("Id Used"=w1711, "Vg-Used"=w1710) -> ("STS"=w1712:dbl)  [unwired: 9 in]
            n884 = Bundle(w1711, w1710) -> (w1717:cluster{dbl[], dbl[]})  [unwired: 1 in]
            n885 = local write "New: STS"(w1712) -> ()
            n886 = Build Array (concatenate)(w1715, w1714, w1717) -> (w1716:cluster{dbl[], dbl[]}[])
            n887 = local write "XY Graph 2"(w1716) -> ()
          }
          event "Save Changes?": Mouse Down {
            n888 = event-data() -> ()  [unwired: 1 in, 5 out]
            n889 = flat-sequence {
              tunnel: [w1751] -> w1728
              tunnel: [w1745] -> w1727
              tunnel: [w1731] -> w1726
              tunnel: w1728 -> [w2032]
              tunnel: w1727 -> [w2029]
              tunnel: [w2030] -> w1725
              tunnel: w1726 -> [w2030]
              tunnel: [w2029] -> w1724
              tunnel: w1725 -> [w2037]
              tunnel: w1724 -> [w2036]
              frame #0 {
                n890 = local read "New: Temp"() -> (w1732:dbl)
                n891 = local read "Data File"() -> (w1751:path)
                n892 = local read "New: Length"() -> (w1736:dbl)
                n893 = local read "New: Width"() -> (w1734:dbl)
                n894 = To Single Precision Float(number=w1732) -> (single precision float=w1733:sgl)
                n895 = call-poly <vilib>:"Read From Spreadsheet File.vi"("file path (dialog if empty)"=w1751) -> ("all rows"=w1729:string[][])  [unwired: 6 in, 4 out]
                n896 = Number To Decimal String(number=w1733) -> (decimal integer string=w1748:string)  [unwired: 1 in]
                n897 = To Single Precision Float(number=w1734) -> (single precision float=w1735:sgl)
                n898 = To Single Precision Float(number=w1736) -> (single precision float=w1737:sgl)
                n899 = local read "Index"() -> (w1754:string)
                n900 = Strip Path(path=w1751) -> (stripped path=w1759:path)  [unwired: 1 out]
                n901 = Number To Decimal String(number=w1737) -> (decimal integer string=w1752:string)  [unwired: 1 in]
                n902 = Number To Decimal String(number=w1735) -> (decimal integer string=w1753:string)  [unwired: 1 in]
                n903 = Array Size(array=w1729) -> (size(s)=w1742:i32[])
                n904 = Concatenate Strings("_", w1748, "K") -> (w1746:string)
                n905 = Array Subset(array=w1729, index (row)=0, index (col)=0, length (col)=3) -> (w1738:string[][])  [unwired: 1 in]
                n906 = Index Array(array=w1742, index=0) -> (element=w1744:i32)
                n907 = call "Build Text"("Temp"=w1746, "Index"=w1754, "Length"=w1752, "Width"=w1753) -> ("Result"=w1755:string)  [unwired: 10 in, 1 out]
                n908 = flat-sequence {
                  tunnel: [w1986] -> w1750
                  tunnel: w1750 -> [w2003]
                  frame #0 {
                    # "Makes Empty File for Transformer Data"
                    n909 = local read "Data Folder"() -> (w1975:path)
                    n910 = Build Path(base path=w1975, name or relative path="Stats") -> (appended path=w1977:path)
                    n911 = call <vilib>:"Check if File or Folder Exists.vi"("path"=w1977) -> ("file or folder exists?"=w1978:bool, "dup path"=w1979:path)  [unwired: 8 in, 1 out]
                    n912 = case shown="False" w1978 {
                      tunnel: [w1983 w1985] -> w1980
                      tunnel: w1979 -> [w1984 w1985]
                      frame False {
                        n913 = Create Folder(path (use dialog)=w1984) -> (created path=w1983:path)  [unwired: 2 in, 2 out]
                      }
                      frame True {
                      }
                    }
                    n914 = Build Path(base path=w1980, name or relative path="Tranformer Data.txt") -> (appended path=w1982:path)
                    n915 = call-poly <vilib>:"Write To Spreadsheet File.vi"("append to file? (new file:F)"=TRUE, "file path (dialog if empty)"=w1982) -> ()  [unwired: 6 in, 1 out]
                  }
                  frame #1 {
                    # "Adds Headers if they don't exist"
                    n916 = Concatenate Strings("Stats\\", "Tranformer Data.txt") -> (w1993:string)
                    n917 = local read "Data Folder"() -> (w1992:path)
                    n918 = Build Path(base path=w1992, name or relative path=w1993) -> (appended path=w1986:path)
                    n919 = call-poly <vilib>:"Read From Spreadsheet File.vi"("file path (dialog if empty)"=w1986) -> ("first row"=w1991:string[])  [unwired: 6 in, 4 out]
                    n920 = Search 1D Array(1D array=w1991, element="DeviceID") -> (index of element=w1989:i32)  [unwired: 1 in]
                    n921 = Equal?(x=w1989, y=0) -> (x = y?=w1987:bool)
                    n922 = case shown="False" w1987 {
                      tunnel: w1986 -> [w1997 _]
                      frame False {
                        n923 = local read "Transformer \nHeaders"() -> (w1996:string[])
                        n924 = call-poly <vilib>:"Write To Spreadsheet File.vi"("1D data"=w1996, "file path (dialog if empty)"=w1997) -> ()  [unwired: 6 in, 1 out]
                      }
                      frame True {
                      }
                    }
                  }
                  frame #2 {
                    # "Adds current device if it doesn't exist"
                    n925 = local read "Current \nRecord"() -> (w2002:string[])
                    n926 = Index Array(array=w2002, index=0) -> (element=w2001:string)
                    n927 = Concatenate Strings("Stats\\", "Tranformer Data.txt") -> (w2006:string)
                    n928 = local read "Data Folder"() -> (w2005:path)
                    n929 = local write "Current Device ID"(w2001) -> ()
                    n930 = local read "Current Device ID"() -> (w2011:string)
                    n931 = Build Path(base path=w2005, name or relative path=w2006) -> (appended path=w2004:path)
                    n932 = call-poly <vilib>:"Read From Spreadsheet File.vi"("file path (dialog if empty)"=w2004) -> ("all rows"=w1998:string[][])  [unwired: 6 in, 4 out]
                    n933 = Index Array(array=w1998, index (col)=0) -> (element=w1999:string[])  [unwired: 1 in]
                    n934 = Search 1D Array(1D array=w1999, element=w2011) -> (index of element=w2000:i32)  [unwired: 1 in]
                    n935 = Equal?(x=w2000, y=-1) -> (x = y?=w2013:bool)
                    n936 = case shown="False" w2013 {
                      tunnel: w2003 -> [w2016 w2027]
                      tunnel: w2000 -> [w2019 _]
                      tunnel: w1998 -> [w2020 _]
                      frame False {
                        n937 = local read "Current \nRecord"() -> (w2018:string[])
                        n938 = Replace Array Subset(array=w2020, new element=w2018, index (row)=w2019) -> (w2017:string[][])  [unwired: 1 in]
                        n939 = flat-sequence {
                          tunnel: w2016 -> [w2021]
                          tunnel: w2017 -> [w2022]
                          tunnel: [w2022] -> w2015
                          tunnel: [w2021] -> w2014
                          tunnel: w2015 -> [w2024]
                          tunnel: w2014 -> [w2023]
                          frame #0 {
                            n940 = Delete(path (use dialog)=w2021) -> ()  [unwired: 4 in, 3 out]
                          }
                          frame #1 {
                            n941 = call-poly <vilib>:"Write To Spreadsheet File.vi"("append to file? (new file:F)"=TRUE, "2D data"=w2024, "file path (dialog if empty)"=w2023) -> ()  [unwired: 5 in, 1 out]
                          }
                        }
                      }
                      frame True {
                        n942 = local read "Current \nRecord"() -> (w2026:string[])
                        n943 = call-poly <vilib>:"Write To Spreadsheet File.vi"("append to file? (new file:F)"=TRUE, "1D data"=w2026, "file path (dialog if empty)"=w2027) -> ()  [unwired: 5 in, 1 out]
                      }
                    }
                  }
                }
                n944 = Reshape Array(w1738, w1744) -> (w1730:string[])
                n945 = Path To String(path=w1759) -> (string=w1757:string)
                n946 = stacked-sequence {
                  tunnel: w1730 -> [w1766 w1779 w1797 w1815 w1833 w1851 w1869 w1887 w1904 w1922 w1940 w1958]
                  tunnel: [_ _ _ _ _ _ _ _ _ _ _ w1956] -> w1731
                  frame #0 {
                    n947 = Search 1D Array(1D array=w1766, element="Dielectric (nm):") -> (index of element=w1763:i32)  [unwired: 1 in]
                    n948 = Equal?(x=w1763, y=-1) -> (x = y?=w1762:bool)
                    n949 = local read "Save1 Array"() -> (w1761:string[][])
                    n950 = case shown="False" w1762 {
                      tunnel: w1761 -> [w1772 w1776]
                      tunnel: w1763 -> [w1768 _]
                      tunnel: [w1767 w1776] -> w1760
                      frame False {
                        n951 = local read "New: Dielectric"() -> (w1774:dbl)
                        n952 = Number To Fractional String(number=w1774) -> (F-format string=w1769:string)  [unwired: 3 in]
                        n953 = Divide(x=w1768, y=3) -> (x/y=w1771:dbl)
                        n954 = To Word Integer(number=w1771) -> (16bit integer=w1770:i16)
                        n955 = Replace Array Subset(array=w1772, new element=w1769, index (row)=w1770, index (col)=1) -> (w1767:string[][])
                      }
                      frame True {
                      }
                    }
                    n956 = local write "Save1 Array"(w1760) -> ()
                  }
                  frame #1 {
                    n957 = Search 1D Array(1D array=w1779, element="Length (um):") -> (index of element=w1781:i32)  [unwired: 1 in]
                    n958 = Equal?(x=w1781, y=-1) -> (x = y?=w1780:bool)
                    n959 = local read "Save1 Array"() -> (w1778:string[][])
                    n960 = case shown="False" w1780 {
                      tunnel: w1778 -> [w1791 w1794]
                      tunnel: w1781 -> [w1788 _]
                      tunnel: [w1787 w1794] -> w1777
                      frame False {
                        n961 = local read "New: Length"() -> (w1784:dbl)
                        n962 = Divide(x=w1788, y=3) -> (x/y=w1790:dbl)
                        n963 = Format Value(format string="%#g", value (0)=w1784) -> (output string=w1785:string)  [unwired: 1 in]
                        n964 = To Word Integer(number=w1790) -> (16bit integer=w1789:i16)
                        n965 = Replace Array Subset(array=w1791, new element=w1785, index (row)=w1789, index (col)=1) -> (w1787:string[][])
                      }
                      frame True {
                      }
                    }
                    n966 = local write "Save1 Array"(w1777) -> ()
                  }
                  frame #2 {
                    n967 = Search 1D Array(1D array=w1797, element="Width (um):") -> (index of element=w1799:i32)  [unwired: 1 in]
                    n968 = Equal?(x=w1799, y=-1) -> (x = y?=w1798:bool)
                    n969 = local read "Save1 Array"() -> (w1796:string[][])
                    n970 = case shown="False" w1798 {
                      tunnel: w1799 -> [w1807 _]
                      tunnel: w1796 -> [w1806 w1812]
                      tunnel: [w1805 w1812] -> w1795
                      frame False {
                        n971 = local read "New: Width"() -> (w1802:dbl)
                        n972 = Divide(x=w1807, y=3) -> (x/y=w1809:dbl)
                        n973 = To Word Integer(number=w1809) -> (16bit integer=w1808:i16)
                        n974 = Format Value(format string="%#g", value (0)=w1802) -> (output string=w1803:string)  [unwired: 1 in]
                        n975 = Replace Array Subset(array=w1806, new element=w1803, index (row)=w1808, index (col)=1) -> (w1805:string[][])
                      }
                      frame True {
                      }
                    }
                    n976 = local write "Save1 Array"(w1795) -> ()
                  }
                  frame #3 {
                    n977 = Search 1D Array(1D array=w1815, element="Sample Temp (K):") -> (index of element=w1817:i32)  [unwired: 1 in]
                    n978 = Equal?(x=w1817, y=-1) -> (x = y?=w1816:bool)
                    n979 = local read "Save1 Array"() -> (w1814:string[][])
                    n980 = case shown="False" w1816 {
                      tunnel: w1814 -> [w1827 w1830]
                      tunnel: w1817 -> [w1824 _]
                      tunnel: [w1823 w1830] -> w1813
                      frame False {
                        n981 = local read "New: Temp"() -> (w1821:dbl)
                        n982 = Divide(x=w1824, y=3) -> (x/y=w1826:dbl)
                        n983 = Format Value(format string="%#g", value (0)=w1821) -> (output string=w1820:string)  [unwired: 1 in]
                        n984 = To Word Integer(number=w1826) -> (16bit integer=w1825:i16)
                        n985 = Replace Array Subset(array=w1827, new element=w1820, index (row)=w1825, index (col)=1) -> (w1823:string[][])
                      }
                      frame True {
                      }
                    }
                    n986 = local write "Save1 Array"(w1813) -> ()
                  }
                  frame #4 {
                    n987 = Search 1D Array(1D array=w1833, element="Mobility-Sat (cm^2/Vs):") -> (index of element=w1835:i32)  [unwired: 1 in]
                    n988 = Equal?(x=w1835, y=-1) -> (x = y?=w1834:bool)
                    n989 = local read "Save1 Array"() -> (w1831:string[][])
                    n990 = case shown="False" w1834 {
                      tunnel: w1831 -> [w1845 w1848]
                      tunnel: w1835 -> [w1842 _]
                      tunnel: [w1841 w1848] -> w1832
                      frame False {
                        n991 = local read "New: Mobility-Sat"() -> (w1838:dbl)
                        n992 = Divide(x=w1842, y=3) -> (x/y=w1844:dbl)
                        n993 = To Word Integer(number=w1844) -> (16bit integer=w1843:i16)
                        n994 = Format Value(format string="%#g", value (0)=w1838) -> (output string=w1839:string)  [unwired: 1 in]
                        n995 = Replace Array Subset(array=w1845, new element=w1839, index (row)=w1843, index (col)=1) -> (w1841:string[][])
                      }
                      frame True {
                      }
                    }
                    n996 = local write "Save1 Array"(w1832) -> ()
                  }
                  frame #5 {
                    n997 = Search 1D Array(1D array=w1851, element="Mobility-Lin (cm^2/Vs):") -> (index of element=w1853:i32)  [unwired: 1 in]
                    n998 = Equal?(x=w1853, y=-1) -> (x = y?=w1852:bool)
                    n999 = local read "Save1 Array"() -> (w1850:string[][])
                    n1000 = case shown="False" w1852 {
                      tunnel: w1850 -> [w1863 w1866]
                      tunnel: w1853 -> [w1860 _]
                      tunnel: [w1859 w1866] -> w1849
                      frame False {
                        n1001 = local read "New: Mobility-Lin"() -> (w1856:dbl)
                        n1002 = Divide(x=w1860, y=3) -> (x/y=w1862:dbl)
                        n1003 = To Word Integer(number=w1862) -> (16bit integer=w1861:i16)
                        n1004 = Format Value(format string="%#g", value (0)=w1856) -> (output string=w1857:string)  [unwired: 1 in]
                        n1005 = Replace Array Subset(array=w1863, new element=w1857, index (row)=w1861, index (col)=1) -> (w1859:string[][])
                      }
                      frame True {
                      }
                    }
                    n1006 = local write "Save1 Array"(w1849) -> ()
                  }
                  frame #6 {
                    n1007 = Search 1D Array(1D array=w1869, element="Off I-Sat (A):") -> (index of element=w1871:i32)  [unwired: 1 in]
                    n1008 = Equal?(x=w1871, y=-1) -> (x = y?=w1870:bool)
                    n1009 = local read "Save1 Array"() -> (w1868:string[][])
                    n1010 = case shown="False" w1870 {
                      tunnel: w1868 -> [w1881 w1884]
                      tunnel: w1871 -> [w1878 _]
                      tunnel: [w1877 w1884] -> w1867
                      frame False {
                        n1011 = local read "Calc: Off I-Sat"() -> (w1876:dbl)
                        n1012 = Divide(x=w1878, y=3) -> (x/y=w1880:dbl)
                        n1013 = Format Value(format string="%#g", value (0)=w1876) -> (output string=w1874:string)  [unwired: 1 in]
                        n1014 = To Word Integer(number=w1880) -> (16bit integer=w1879:i16)
                        n1015 = Replace Array Subset(array=w1881, new element=w1874, index (row)=w1879, index (col)=1) -> (w1877:string[][])
                      }
                      frame True {
                      }
                    }
                    n1016 = local write "Save1 Array"(w1867) -> ()
                  }
                  frame #7 {
                    n1017 = Search 1D Array(1D array=w1887, element="Vt-Sat (V):") -> (index of element=w1889:i32)  [unwired: 1 in]
                    n1018 = Equal?(x=w1889, y=-1) -> (x = y?=w1888:bool)
                    n1019 = local read "Save1 Array"() -> (w1886:string[][])
                    n1020 = case shown="False" w1888 {
                      tunnel: w1886 -> [w1897 w1901]
                      tunnel: w1889 -> [w1893 _]
                      tunnel: [w1892 w1901] -> w1885
                      frame False {
                        n1021 = local read "New: VT-Sat"() -> (w1899:dbl)
                        n1022 = Number To Fractional String(number=w1899) -> (F-format string=w1894:string)  [unwired: 3 in]
                        n1023 = Divide(x=w1893, y=3) -> (x/y=w1896:dbl)
                        n1024 = To Word Integer(number=w1896) -> (16bit integer=w1895:i16)
                        n1025 = Replace Array Subset(array=w1897, new element=w1894, index (row)=w1895, index (col)=1) -> (w1892:string[][])
                      }
                      frame True {
                      }
                    }
                    n1026 = local write "Save1 Array"(w1885) -> ()
                  }
                  frame #8 {
                    n1027 = Search 1D Array(1D array=w1904, element="VT-Lin (V):") -> (index of element=w1906:i32)  [unwired: 1 in]
                    n1028 = Equal?(x=w1906, y=-1) -> (x = y?=w1905:bool)
                    n1029 = local read "Save1 Array"() -> (w1903:string[][])
                    n1030 = case shown="False" w1905 {
                      tunnel: w1903 -> [w1916 w1919]
                      tunnel: w1906 -> [w1913 _]
                      tunnel: [w1912 w1919] -> w1902
                      frame False {
                        n1031 = local read "New: VT-Lin"() -> (w1910:dbl)
                        n1032 = Divide(x=w1913, y=3) -> (x/y=w1915:dbl)
                        n1033 = Format Value(format string="%#g", value (0)=w1910) -> (output string=w1909:string)  [unwired: 1 in]
                        n1034 = To Word Integer(number=w1915) -> (16bit integer=w1914:i16)
                        n1035 = Replace Array Subset(array=w1916, new element=w1909, index (row)=w1914, index (col)=1) -> (w1912:string[][])
                      }
                      frame True {
                      }
                    }
                    n1036 = local write "Save1 Array"(w1902) -> ()
                  }
                  frame #9 {
                    n1037 = Search 1D Array(1D array=w1922, element="STS-Sat (V/decade):") -> (index of element=w1924:i32)  [unwired: 1 in]
                    n1038 = Equal?(x=w1924, y=-1) -> (x = y?=w1923:bool)
                    n1039 = local read "Save1 Array"() -> (w1921:string[][])
                    n1040 = case shown="False" w1923 {
                      tunnel: w1921 -> [w1934 w1937]
                      tunnel: w1924 -> [w1931 _]
                      tunnel: [w1930 w1937] -> w1920
                      frame False {
                        n1041 = local read "New: STS"() -> (w1928:dbl)
                        n1042 = Divide(x=w1931, y=3) -> (x/y=w1933:dbl)
                        n1043 = Format Value(format string="%#g", value (0)=w1928) -> (output string=w1927:string)  [unwired: 1 in]
                        n1044 = To Word Integer(number=w1933) -> (16bit integer=w1932:i16)
                        n1045 = Replace Array Subset(array=w1934, new element=w1927, index (row)=w1932, index (col)=1) -> (w1930:string[][])
                      }
                      frame True {
                      }
                    }
                    n1046 = local write "Save1 Array"(w1920) -> ()
                  }
                  frame #10 {
                    n1047 = Search 1D Array(1D array=w1940, element="Trap Density-VT (Traps/Vcm^2):") -> (index of element=w1942:i32)  [unwired: 1 in]
                    n1048 = Equal?(x=w1942, y=-1) -> (x = y?=w1941:bool)
                    n1049 = local read "Save1 Array"() -> (w1939:string[][])
                    n1050 = case shown="False" w1941 {
                      tunnel: w1939 -> [w1952 w1955]
                      tunnel: w1942 -> [w1948 _]
                      tunnel: [w1947 w1955] -> w1938
                      frame False {
                        n1051 = local read "New: Trap Density-VT"() -> (w1946:dbl)
                        n1052 = Format Value(format string="%#g", value (0)=w1946) -> (output string=w1949:string)  [unwired: 1 in]
                        n1053 = Divide(x=w1948, y=3) -> (x/y=w1951:dbl)
                        n1054 = To Word Integer(number=w1951) -> (16bit integer=w1950:i16)
                        n1055 = Replace Array Subset(array=w1952, new element=w1949, index (row)=w1950, index (col)=1) -> (w1947:string[][])
                      }
                      frame True {
                      }
                    }
                    n1056 = local write "Save1 Array"(w1938) -> ()
                  }
                  frame #11 {
                    n1057 = Search 1D Array(1D array=w1958, element="Trap Density-STS (Traps/Vcm^2):") -> (index of element=w1960:i32)  [unwired: 1 in]
                    n1058 = Equal?(x=w1960, y=-1) -> (x = y?=w1959:bool)
                    n1059 = local read "Save1 Array"() -> (w1957:string[][])
                    n1060 = case shown="False" w1959 {
                      tunnel: w1957 -> [w1970 w1973]
                      tunnel: w1960 -> [w1967 _]
                      tunnel: [w1966 w1973] -> w1956
                      frame False {
                        n1061 = local read "New: Trap Density-STS"() -> (w1964:dbl)
                        n1062 = Divide(x=w1967, y=3) -> (x/y=w1969:dbl)
                        n1063 = To Word Integer(number=w1969) -> (16bit integer=w1968:i16)
                        n1064 = Format Value(format string="%#g", value (0)=w1964) -> (output string=w1963:string)  [unwired: 1 in]
                        n1065 = Replace Array Subset(array=w1970, new element=w1963, index (row)=w1968, index (col)=1) -> (w1966:string[][])
                      }
                      frame True {
                      }
                    }
                    n1066 = local write "Save1 Array"(w1956) -> ()
                  }
                }
                n1067 = Concatenate Strings(w1757, "\\", w1755) -> (w1756:string)
                n1068 = String To Path(string=w1756) -> (path=w1745:path)
                n1069 = local write "Save1 Array"(w1729) -> ()
              }
              frame #1 {
                n1070 = Equal?(x=w2032, y=w2029) -> (x = y?=w2031:bool)
                n1071 = case shown="False" w2031 {
                  tunnel: w2032 -> [w2035 _]
                  tunnel: w2029 -> [w2034 _]
                  frame False {
                    n1072 = Move(source path=w2035, 9:TRUE, 10:w2034) -> ()  [unwired: 2 in, 3 out]
                  }
                  frame True {
                  }
                }
              }
              frame #2 {
                n1073 = local write "Data File"(w2036) -> ()
                n1074 = call-poly <vilib>:"Write To Spreadsheet File.vi"("2D data"=w2037, "file path (dialog if empty)"=w2036) -> ()  [unwired: 6 in, 1 out]
              }
            }
          }
          event "Save Changes? 2": Mouse Down {
            n1075 = event-data() -> ()  [unwired: 1 in, 5 out]
            n1076 = stacked-sequence {
              seq-local: [w2097 _ _ _ _] -> [_ w2332 _ _ _]
              seq-local: [w2100 _ _ _ _] -> [_ w2333 _ _ _]
              seq-local: [w2097 _ _ _ _] -> [_ w2331 _ _ _]
              seq-local: [w2095 _ _ _ _] -> [_ w2329 _ _ _]
              seq-local: [_ w2333 _ _ _] -> [_ _ w2338 _ _]
              seq-local: [_ w2329 _ _ _] -> [_ _ w2337 _ _]
              frame #0 {
                n1077 = local read "New: Temp"() -> (w2099:dbl)
                n1078 = local read "Data File"() -> (w2100:path)
                n1079 = local read "New: Length"() -> (w2103:dbl)
                n1080 = local read "New: Width"() -> (w2101:dbl)
                n1081 = To Word Integer(number=w2099) -> (16bit integer=w2098:i16)
                n1082 = call-poly <vilib>:"Read From Spreadsheet File.vi"("file path (dialog if empty)"=w2100) -> ("all rows"=w2094:string[][])  [unwired: 6 in, 4 out]
                n1083 = Number To Decimal String(number=w2098) -> (decimal integer string=w2114:string)  [unwired: 1 in]
                n1084 = To Single Precision Float(number=w2101) -> (single precision float=w2102:sgl)
                n1085 = To Single Precision Float(number=w2103) -> (single precision float=w2104:sgl)
                n1086 = local read "Index"() -> (w2118:string)
                n1087 = Strip Path(path=w2100) -> (stripped path=w2123:path)  [unwired: 1 out]
                n1088 = Number To Decimal String(number=w2104) -> (decimal integer string=w2116:string)  [unwired: 1 in]
                n1089 = Number To Decimal String(number=w2102) -> (decimal integer string=w2117:string)  [unwired: 1 in]
                n1090 = Array Size(array=w2094) -> (size(s)=w2109:i32[])
                n1091 = Concatenate Strings("_", w2114, "K") -> (w2112:string)
                n1092 = Array Subset(array=w2094, index (row)=0, index (col)=0, length (col)=3) -> (w2105:string[][])  [unwired: 1 in]
                n1093 = Index Array(array=w2109, index=0) -> (element=w2111:i32)
                n1094 = call "Build Text2"("Temp"=w2112, "Index"=w2118, "Length"=w2116, "Width"=w2117) -> ("Result"=w2119:string)  [unwired: 10 in, 1 out]
                n1095 = Reshape Array(w2105, w2111) -> (w2096:string[])
                n1096 = Path To String(path=w2123) -> (string=w2121:string)
                n1097 = stacked-sequence {
                  tunnel: w2096 -> [w2130 w2143 w2160 w2177 w2194 w2211 w2228 w2246 w2263 w2280 w2297 w2314]
                  tunnel: [_ _ _ _ _ _ _ _ _ _ _ w2312] -> w2095
                  frame #0 {
                    n1098 = Search 1D Array(1D array=w2130, element="Dielectric (nm):") -> (index of element=w2127:i32)  [unwired: 1 in]
                    n1099 = Equal?(x=w2127, y=-1) -> (x = y?=w2126:bool)
                    n1100 = local read "Save1 Array"() -> (w2125:string[][])
                    n1101 = case shown="False" w2126 {
                      tunnel: w2125 -> [w2136 w2140]
                      tunnel: w2127 -> [w2132 _]
                      tunnel: [w2131 w2140] -> w2124
                      frame False {
                        n1102 = local read "New: Dielectric"() -> (w2138:dbl)
                        n1103 = Number To Fractional String(number=w2138) -> (F-format string=w2133:string)  [unwired: 3 in]
                        n1104 = Divide(x=w2132, y=3) -> (x/y=w2135:dbl)
                        n1105 = To Word Integer(number=w2135) -> (16bit integer=w2134:i16)
                        n1106 = Replace Array Subset(array=w2136, new element=w2133, index (row)=w2134, index (col)=1) -> (w2131:string[][])
                      }
                      frame True {
                      }
                    }
                    n1107 = local write "Save1 Array"(w2124) -> ()
                  }
                  frame #1 {
                    n1108 = Search 1D Array(1D array=w2143, element="Length (um):") -> (index of element=w2145:i32)  [unwired: 1 in]
                    n1109 = Equal?(x=w2145, y=-1) -> (x = y?=w2144:bool)
                    n1110 = local read "Save1 Array"() -> (w2142:string[][])
                    n1111 = case shown="True" w2144 {
                      tunnel: w2142 -> [w2153 w2157]
                      tunnel: w2145 -> [w2149 _]
                      tunnel: [w2148 w2157] -> w2141
                      frame False {
                        n1112 = local read "New: Length"() -> (w2155:dbl)
                        n1113 = Number To Fractional String(number=w2155) -> (F-format string=w2150:string)  [unwired: 3 in]
                        n1114 = Divide(x=w2149, y=3) -> (x/y=w2152:dbl)
                        n1115 = To Word Integer(number=w2152) -> (16bit integer=w2151:i16)
                        n1116 = Replace Array Subset(array=w2153, new element=w2150, index (row)=w2151, index (col)=1) -> (w2148:string[][])
                      }
                      frame True {
                      }
                    }
                    n1117 = local write "Save1 Array"(w2141) -> ()
                  }
                  frame #2 {
                    n1118 = Search 1D Array(1D array=w2160, element="Width (um):") -> (index of element=w2162:i32)  [unwired: 1 in]
                    n1119 = Equal?(x=w2162, y=-1) -> (x = y?=w2161:bool)
                    n1120 = local read "Save1 Array"() -> (w2159:string[][])
                    n1121 = case shown="False" w2161 {
                      tunnel: w2162 -> [w2167 _]
                      tunnel: w2159 -> [w2166 w2174]
                      tunnel: [w2165 w2174] -> w2158
                      frame False {
                        n1122 = local read "New: Width"() -> (w2172:dbl)
                        n1123 = Number To Fractional String(number=w2172) -> (F-format string=w2168:string)  [unwired: 3 in]
                        n1124 = Divide(x=w2167, y=3) -> (x/y=w2170:dbl)
                        n1125 = To Word Integer(number=w2170) -> (16bit integer=w2169:i16)
                        n1126 = Replace Array Subset(array=w2166, new element=w2168, index (row)=w2169, index (col)=1) -> (w2165:string[][])
                      }
                      frame True {
                      }
                    }
                    n1127 = local write "Save1 Array"(w2158) -> ()
                  }
                  frame #3 {
                    n1128 = Search 1D Array(1D array=w2177, element="Sample Temp (K):") -> (index of element=w2179:i32)  [unwired: 1 in]
                    n1129 = Equal?(x=w2179, y=-1) -> (x = y?=w2178:bool)
                    n1130 = local read "Save1 Array"() -> (w2176:string[][])
                    n1131 = case shown="False" w2178 {
                      tunnel: w2176 -> [w2187 w2191]
                      tunnel: w2179 -> [w2183 _]
                      tunnel: [w2182 w2191] -> w2175
                      frame False {
                        n1132 = local read "New: Temp"() -> (w2189:dbl)
                        n1133 = Number To Fractional String(number=w2189) -> (F-format string=w2184:string)  [unwired: 3 in]
                        n1134 = Divide(x=w2183, y=3) -> (x/y=w2186:dbl)
                        n1135 = To Word Integer(number=w2186) -> (16bit integer=w2185:i16)
                        n1136 = Replace Array Subset(array=w2187, new element=w2184, index (row)=w2185, index (col)=1) -> (w2182:string[][])
                      }
                      frame True {
                      }
                    }
                    n1137 = local write "Save1 Array"(w2175) -> ()
                  }
                  frame #4 {
                    n1138 = Search 1D Array(1D array=w2194, element="Mobility-Sat (cm^2/Vs):") -> (index of element=w2196:i32)  [unwired: 1 in]
                    n1139 = Equal?(x=w2196, y=-1) -> (x = y?=w2195:bool)
                    n1140 = local read "Save1 Array"() -> (w2192:string[][])
                    n1141 = case shown="False" w2195 {
                      tunnel: w2192 -> [w2204 w2208]
                      tunnel: w2196 -> [w2200 _]
                      tunnel: [w2199 w2208] -> w2193
                      frame False {
                        n1142 = local read "New: Mobility-Sat"() -> (w2206:dbl)
                        n1143 = Number To Fractional String(number=w2206) -> (F-format string=w2201:string)  [unwired: 3 in]
                        n1144 = Divide(x=w2200, y=3) -> (x/y=w2203:dbl)
                        n1145 = To Word Integer(number=w2203) -> (16bit integer=w2202:i16)
                        n1146 = Replace Array Subset(array=w2204, new element=w2201, index (row)=w2202, index (col)=1) -> (w2199:string[][])
                      }
                      frame True {
                      }
                    }
                    n1147 = local write "Save1 Array"(w2193) -> ()
                  }
                  frame #5 {
                    n1148 = Search 1D Array(1D array=w2211, element="Mobility-Lin (cm^2/Vs):") -> (index of element=w2213:i32)  [unwired: 1 in]
                    n1149 = Equal?(x=w2213, y=-1) -> (x = y?=w2212:bool)
                    n1150 = local read "Save1 Array"() -> (w2210:string[][])
                    n1151 = case shown="False" w2212 {
                      tunnel: w2210 -> [w2221 w2225]
                      tunnel: w2213 -> [w2217 _]
                      tunnel: [w2216 w2225] -> w2209
                      frame False {
                        n1152 = local read "New: Mobility-Lin"() -> (w2223:dbl)
                        n1153 = Number To Fractional String(number=w2223) -> (F-format string=w2218:string)  [unwired: 3 in]
                        n1154 = Divide(x=w2217, y=3) -> (x/y=w2220:dbl)
                        n1155 = To Word Integer(number=w2220) -> (16bit integer=w2219:i16)
                        n1156 = Replace Array Subset(array=w2221, new element=w2218, index (row)=w2219, index (col)=1) -> (w2216:string[][])
                      }
                      frame True {
                      }
                    }
                    n1157 = local write "Save1 Array"(w2209) -> ()
                  }
                  frame #6 {
                    n1158 = Search 1D Array(1D array=w2228, element="Off I-Sat (A):") -> (index of element=w2230:i32)  [unwired: 1 in]
                    n1159 = Equal?(x=w2230, y=-1) -> (x = y?=w2229:bool)
                    n1160 = local read "Save1 Array"() -> (w2227:string[][])
                    n1161 = case shown="False" w2229 {
                      tunnel: w2227 -> [w2240 w2243]
                      tunnel: w2230 -> [w2237 _]
                      tunnel: [w2236 w2243] -> w2226
                      frame False {
                        n1162 = local read "Calc: Off I-Sat"() -> (w2235:dbl)
                        n1163 = Format Value(format string="%#g", value (0)=w2235) -> (output string=w2234:string)  [unwired: 1 in]
                        n1164 = Divide(x=w2237, y=3) -> (x/y=w2239:dbl)
                        n1165 = To Word Integer(number=w2239) -> (16bit integer=w2238:i16)
                        n1166 = Replace Array Subset(array=w2240, new element=w2234, index (row)=w2238, index (col)=1) -> (w2236:string[][])
                      }
                      frame True {
                      }
                    }
                    n1167 = local write "Save1 Array"(w2226) -> ()
                  }
                  frame #7 {
                    n1168 = Search 1D Array(1D array=w2246, element="Vt-Sat (V):") -> (index of element=w2248:i32)  [unwired: 1 in]
                    n1169 = Equal?(x=w2248, y=-1) -> (x = y?=w2247:bool)
                    n1170 = local read "Save1 Array"() -> (w2245:string[][])
                    n1171 = case shown="False" w2247 {
                      tunnel: w2245 -> [w2256 w2260]
                      tunnel: w2248 -> [w2252 _]
                      tunnel: [w2251 w2260] -> w2244
                      frame False {
                        n1172 = local read "New: VT-Sat"() -> (w2258:dbl)
                        n1173 = Number To Fractional String(number=w2258) -> (F-format string=w2253:string)  [unwired: 3 in]
                        n1174 = Divide(x=w2252, y=3) -> (x/y=w2255:dbl)
                        n1175 = To Word Integer(number=w2255) -> (16bit integer=w2254:i16)
                        n1176 = Replace Array Subset(array=w2256, new element=w2253, index (row)=w2254, index (col)=1) -> (w2251:string[][])
                      }
                      frame True {
                      }
                    }
                    n1177 = local write "Save1 Array"(w2244) -> ()
                  }
                  frame #8 {
                    n1178 = Search 1D Array(1D array=w2263, element="VT-Lin (V):") -> (index of element=w2265:i32)  [unwired: 1 in]
                    n1179 = Equal?(x=w2265, y=-1) -> (x = y?=w2264:bool)
                    n1180 = local read "Save1 Array"() -> (w2262:string[][])
                    n1181 = case shown="True" w2264 {
                      tunnel: w2262 -> [w2273 w2277]
                      tunnel: w2265 -> [w2269 _]
                      tunnel: [w2268 w2277] -> w2261
                      frame False {
                        n1182 = local read "New: VT-Lin"() -> (w2275:dbl)
                        n1183 = Number To Fractional String(number=w2275) -> (F-format string=w2270:string)  [unwired: 3 in]
                        n1184 = Divide(x=w2269, y=3) -> (x/y=w2272:dbl)
                        n1185 = To Word Integer(number=w2272) -> (16bit integer=w2271:i16)
                        n1186 = Replace Array Subset(array=w2273, new element=w2270, index (row)=w2271, index (col)=1) -> (w2268:string[][])
                      }
                      frame True {
                      }
                    }
                    n1187 = local write "Save1 Array"(w2261) -> ()
                  }
                  frame #9 {
                    n1188 = Search 1D Array(1D array=w2280, element="STS-Sat (V/decade):") -> (index of element=w2282:i32)  [unwired: 1 in]
                    n1189 = Equal?(x=w2282, y=-1) -> (x = y?=w2281:bool)
                    n1190 = local read "Save1 Array"() -> (w2279:string[][])
                    n1191 = case shown="False" w2281 {
                      tunnel: w2279 -> [w2290 w2294]
                      tunnel: w2282 -> [w2286 _]
                      tunnel: [w2285 w2294] -> w2278
                      frame False {
                        n1192 = local read "New: STS"() -> (w2292:dbl)
                        n1193 = Number To Fractional String(number=w2292) -> (F-format string=w2287:string)  [unwired: 3 in]
                        n1194 = Divide(x=w2286, y=3) -> (x/y=w2289:dbl)
                        n1195 = To Word Integer(number=w2289) -> (16bit integer=w2288:i16)
                        n1196 = Replace Array Subset(array=w2290, new element=w2287, index (row)=w2288, index (col)=1) -> (w2285:string[][])
                      }
                      frame True {
                      }
                    }
                    n1197 = local write "Save1 Array"(w2278) -> ()
                  }
                  frame #10 {
                    n1198 = Search 1D Array(1D array=w2297, element="Trap Density-VT (Traps/Vcm^2):") -> (index of element=w2299:i32)  [unwired: 1 in]
                    n1199 = Equal?(x=w2299, y=-1) -> (x = y?=w2298:bool)
                    n1200 = local read "Save1 Array"() -> (w2296:string[][])
                    n1201 = case shown="False" w2298 {
                      tunnel: w2296 -> [w2307 w2311]
                      tunnel: w2299 -> [w2303 _]
                      tunnel: [w2302 w2311] -> w2295
                      frame False {
                        n1202 = local read "New: Trap Density-VT"() -> (w2309:dbl)
                        n1203 = Number To Fractional String(number=w2309) -> (F-format string=w2304:string)  [unwired: 3 in]
                        n1204 = Divide(x=w2303, y=3) -> (x/y=w2306:dbl)
                        n1205 = To Word Integer(number=w2306) -> (16bit integer=w2305:i16)
                        n1206 = Replace Array Subset(array=w2307, new element=w2304, index (row)=w2305, index (col)=1) -> (w2302:string[][])
                      }
                      frame True {
                      }
                    }
                    n1207 = local write "Save1 Array"(w2295) -> ()
                  }
                  frame #11 {
                    n1208 = Search 1D Array(1D array=w2314, element="Trap Density-STS (Traps/Vcm^2):") -> (index of element=w2316:i32)  [unwired: 1 in]
                    n1209 = Equal?(x=w2316, y=-1) -> (x = y?=w2315:bool)
                    n1210 = local read "Save1 Array"() -> (w2313:string[][])
                    n1211 = case shown="False" w2315 {
                      tunnel: w2313 -> [w2324 w2328]
                      tunnel: w2316 -> [w2320 _]
                      tunnel: [w2319 w2328] -> w2312
                      frame False {
                        n1212 = local read "New: Trap Density-STS"() -> (w2326:dbl)
                        n1213 = Number To Fractional String(number=w2326) -> (F-format string=w2321:string)  [unwired: 3 in]
                        n1214 = Divide(x=w2320, y=3) -> (x/y=w2323:dbl)
                        n1215 = To Word Integer(number=w2323) -> (16bit integer=w2322:i16)
                        n1216 = Replace Array Subset(array=w2324, new element=w2321, index (row)=w2322, index (col)=1) -> (w2319:string[][])
                      }
                      frame True {
                      }
                    }
                    n1217 = local write "Save1 Array"(w2312) -> ()
                  }
                }
                n1218 = Concatenate Strings(w2121, "\\", w2119) -> (w2120:string)
                n1219 = String To Path(string=w2120) -> (path=w2097:path)
                "No Image 2" <- w2097
                n1220 = local write "Save1 Array"(w2094) -> ()
              }
              frame #1 {
                n1221 = Equal?(x=w2332, y=w2331) -> (x = y?=w2330:bool)
                n1222 = case shown="False" w2330 {
                  tunnel: w2332 -> [w2336 _]
                  tunnel: w2331 -> [w2335 _]
                  frame False {
                    n1223 = Move(source path=w2336, 9:TRUE, 10:w2335) -> ()  [unwired: 2 in, 3 out]
                  }
                  frame True {
                  }
                }
              }
              frame #2 {
                n1224 = local write "Data File"(w2338) -> ()
                n1225 = call-poly <vilib>:"Write To Spreadsheet File.vi"("2D data"=w2337, "file path (dialog if empty)"=w2338) -> ()  [unwired: 6 in, 1 out]
              }
              frame #3 {
                w2437 = 0
                # "Moves to next file and displays new image/data"
                n1226 = property on="Image Out" class="ImageControl"() -> (error out=w2399:errorcluster, "Image Center Position"=w2403:cluster{"X":u32, "Y":u32})  [unwired: 2 in, 1 out]
                n1227 = local read "Data File"() -> (w2442:path)
                n1228 = Strip Path(path=w2442) -> (stripped path=w2433:path, name=w2451:string)
                n1229 = Unbundle(w2403) -> ("X"=w2401:u32)  [unwired: 1 out]
                n1230 = local write "Data Folder"(w2433) -> ()
                n1231 = Bundle("X"=w2401, 0) -> (w2402:cluster{"X":u32, i32})  [unwired: 1 in]
                n1232 = property on="Image Out" class="ImageControl"(error in=w2399, "Image Center Position"=w2402) -> ()  [unwired: 1 in, 2 out]
                n1233 = List Folder(path=w2433) -> (filenames=w2447:string[])  [unwired: 3 in, 3 out]
                n1234 = Search 1D Array(1D array=w2447, element=w2451) -> (index of element=w2444:i32)  [unwired: 1 in]
                n1235 = Array Size(array=w2447) -> (size(s)=w2443:i32)
                n1236 = Decrement(x=w2443) -> (x-1=w2445:i32)
                n1237 = Equal?(x=w2444, y=w2445) -> (x = y?=w2446:bool)
                n1238 = local read "Folder Index"() -> (w2395:dbl)
                n1239 = case shown="False" w2446 {
                  tunnel: w2395 -> [w2576 _]
                  tunnel: [w2575 0] -> w2394
                  frame False {
                    n1240 = Increment(x=w2576) -> (x+1=w2575:dbl)
                  }
                  frame True {
                  }
                }
                n1241 = invoke on="Image Out" class="ImageControl" method="Clear ROI"() -> ()  [unwired: 3 in, 3 out]
                n1242 = local write "Folder Index"(w2394) -> ()
                n1243 = Path To String(path=w2433) -> (string=w2452:string)
                n1244 = Index Array(array=w2447, index=w2394) -> (element=w2448:string)
                n1245 = local write "Data Name:"(w2448) -> ()
                n1246 = Concatenate Strings(w2452, "\\", w2448) -> (w2450:string)
                n1247 = String To Path(string=w2450) -> (path=w2345:path)
                n1248 = call "Recorded Values.vi"("Path"=w2345) -> ("Recorded Char"=w2347:T5, "Recorded Prop"=w2348:T6, "Fabrication Prop"=w2346:T7)  [unwired: 8 in]
                n1249 = Unbundle By Name(w2347) -> ("Mobility-Sat"=w2360:dbl, "Moblitity-Lin"=w2361:dbl, "On/Off"=w2362:dbl, "Off Current"=w2363:dbl, "Vt-Sat"=w2339:dbl, "STS"=w2364:dbl, "Trap Density-VT"=w2365:dbl, "Trap Density-STS"=w2366:dbl)
                n1250 = Unbundle By Name(w2348) -> ("Date Recorded"=w2356:string, "Index"=w2357:string, "Length"=w2358:dbl, "Width"=w2359:dbl, "Sample Temp"=w2342:dbl)
                n1251 = Unbundle By Name(w2346) -> ("Date Created"=w2367:string, "Material"=w2349:string, "Solvent"=w2350:string, "Concentration"=w2351:dbl, "Method"=w2352:string, "Dielectric (nm)"=w2353:dbl, "Treatment"=w2354:string, "Comments"=w2355:string)
                n1252 = local write "Rec: Off I-Sat"(w2363) -> ()
                n1253 = local write "Rec: VT-Sat"(w2339) -> ()
                n1254 = local write "Date Created"(w2367) -> ()
                n1255 = local write "Rec: Material"(w2349) -> ()
                n1256 = local write "Rec: Solvent"(w2350) -> ()
                n1257 = local write "Rec: Concentration"(w2351) -> ()
                n1258 = local write "Rec: Method"(w2352) -> ()
                n1259 = local write "Rec: Dielectric (d)"(w2353) -> ()
                n1260 = local write "Surface Treatment:"(w2354) -> ()
                n1261 = local write "Comments"(w2355) -> ()
                n1262 = local write "Index"(w2357) -> ()
                n1263 = local write "Rec: Mobility-Sat"(w2360) -> ()
                n1264 = local write "Rec: Mobility-Lin"(w2361) -> ()
                n1265 = local write "Rec: On/Off"(w2362) -> ()
                n1266 = local write "Rec: STS"(w2364) -> ()
                n1267 = local write "Rec: Trap Density-VT"(w2365) -> ()
                n1268 = local write "Rec: Trap Density-STS"(w2366) -> ()
                n1269 = local write "Date Recorded"(w2356) -> ()
                n1270 = local write "Rec: Length"(w2358) -> ()
                n1271 = local write "Rec: Width"(w2359) -> ()
                n1272 = local write "Rec: Temp"(w2342) -> ()
                n1273 = Equal To 0?(x=w2342) -> (x = 0?=w2343:bool)
                n1274 = case shown="False" w2343 {
                  tunnel: [w2453 w2454] -> w2340
                  tunnel: w2342 -> [w2453 _]
                  frame False {
                  }
                  frame True {
                    n1275 = local read "Room Temp"() -> (w2454:dbl)
                  }
                }
                n1276 = local write "Data File"(w2345) -> ()
                n1277 = local read "NumPts 2"() -> (w2390:dbl)
                n1278 = local read "NumPts"() -> (w2379:dbl)
                n1279 = local read "NumPts"() -> (w2391:dbl)
                n1280 = call-poly <vilib>:"Read From Spreadsheet File.vi"("file path (dialog if empty)"=w2345) -> ("all rows"=w2439:string[][])  [unwired: 6 in, 4 out]
                n1281 = call "Mobility-Vt Calculator-File.vi"("NumPts"=w2391, "Path"=w2345) -> ("XY Graph-Sat"=w2392:cluster{dbl[], dbl[]}[], "XY Graph-Lin"=w2374:cluster{dbl[], dbl[]}[], "Output"=w2393:T8, "Index-Sat"=w2371:dbl, "Index-Lin"=w2378:dbl)  [unwired: 4 in, 1 out]
                n1282 = Decimate 1D Array(w2374) -> (w2386:cluster{dbl[], dbl[]}[])  [unwired: 1 out]
                n1283 = Array To Cluster(array=w2386) -> (cluster=w2384:T9)
                n1284 = Unbundle(w2384) -> ("[0]"=w2385:cluster{dbl[], dbl[]})  [unwired: 8 out]
                n1285 = local write "XY Graph-Lin"(w2374) -> ()
                n1286 = Unbundle(w2385) -> (w2383:dbl[], w2382:dbl[])
                n1287 = Array Subset(array=w2382, index=w2378, length=w2379) -> (w2380:dbl[])
                n1288 = Array Subset(array=w2383, index=w2378, length=w2379) -> (w2381:dbl[])
                n1289 = call "STS Calculator-File.vi"("NumPts"=w2390, "Path"=w2345) -> ("STS Index-Sat"=w2389:dbl, "XY Graph-Sat"=w2388:cluster{dbl[], dbl[]}[], "Ouput"=w2387:cluster{"STS-Sat":dbl, "STS-Lin":dbl})  [unwired: 5 in, 2 out]
                n1290 = local read "New: Dielectric"() -> (w2373:dbl)
                n1291 = local write "Lin Id-Used"(w2380) -> ()
                n1292 = local write "Lin-Vg Array-Used"(w2381) -> ()
                n1293 = local write "MobVi Index"(w2371) -> ()
                n1294 = local write "Slide"(w2371) -> ()
                n1295 = local write "XY Graph"(w2392) -> ()
                n1296 = local write "Index 2"(w2389) -> ()
                n1297 = local write "XY Graph 2"(w2388) -> ()
                n1298 = Unbundle By Name(w2393) -> ("Mobility-Sat"=w2377:dbl, "Vt-Sat"=w2370:dbl, "Mobility-Lin"=w2376:dbl, "Mobility-Lin"=w2375:dbl, "Off I-Sat"=w2368:dbl)
                n1299 = Array Size(array=w2439) -> (size(s)=w2438:i32[])
                n1300 = local write "Calc: Off I-Sat"(w2368) -> ()
                n1301 = local write "New: Temp"(w2340) -> ()
                n1302 = Unbundle By Name(w2387) -> ("STS-Sat"=w2372:dbl)
                n1303 = call "Trap Density_STS.vi"("Temp (T) [K]"=w2340, "S.T.S. (S)"=w2372, "Dielectric"=w2373) -> ("Trap Density (N)"=w2344:dbl)  [unwired: 8 in]
                n1304 = local write "Calc: Mobility-Sat"(w2377) -> ()
                n1305 = local write "Calc: Mobility-Lin"(w2375) -> ()
                n1306 = local write "New: Trap Density-STS"(w2344) -> ()
                n1307 = local write "Calc: Trap Density-STS"(w2344) -> ()
                n1308 = local read "Image Folder"() -> (w2427:path)
                n1309 = local write "Calc: VT-Sat"(w2370) -> ()
                n1310 = local write "Calc: VT-Lin"(w2376) -> ()
                n1311 = local read "New: Dielectric"() -> (w2369:dbl)
                n1312 = Decimate 1D Array(w2392) -> (w2422:cluster{dbl[], dbl[]}[])  [unwired: 1 out]
                n1313 = Index Array(array=w2438, index=w2437) -> (element=w2418:i32)
                n1314 = Decimate 1D Array(w2388) -> (w2412:cluster{dbl[], dbl[]}[])  [unwired: 1 out]
                n1315 = Array Subset(array=w2439, index (row)=w2437, index (col)=w2437, length (col)=3) -> (w2440:string[][])  [unwired: 1 in]
                n1316 = local write "Calc: STS"(w2372) -> ()
                n1317 = List Folder(path=w2427) -> (filenames=w2432:string[])  [unwired: 3 in, 3 out]
                n1318 = local write "New: Mobility-Sat"(w2377) -> ()
                n1319 = Array To Cluster(array=w2422) -> (cluster=w2424:T9)
                n1320 = Array To Cluster(array=w2412) -> (cluster=w2410:T9)
                n1321 = Reshape Array(w2440, w2418) -> (w2425:string[])
                n1322 = local write "New: Mobility-Lin"(w2376) -> ()
                n1323 = Subtract(x=w2418, y=20) -> (x-y=w2417:i32)
                n1324 = local write "New: VT-Sat"(w2370) -> ()
                n1325 = local write "New: VT-Lin"(w2375) -> ()
                n1326 = local write "New: STS"(w2372) -> ()
                n1327 = property on="Slide" class="Slide (strict)"("Scale.Maximum"=w2417) -> ()  [unwired: 2 in, 2 out]
                n1328 = call "Trap Density_VT.vi"("VT"=w2370, "Dielectric"=w2369) -> ("Trap Density-VT"=w2341:dbl)
                n1329 = Unbundle(w2424) -> ("[0]"=w2423:cluster{dbl[], dbl[]})  [unwired: 8 out]
                n1330 = Unbundle(w2410) -> ("[0]"=w2411:cluster{dbl[], dbl[]})  [unwired: 8 out]
                n1331 = Search 1D Array(1D array=w2425, element="Index:") -> (index of element=w2434:i32)  [unwired: 1 in]
                n1332 = local write "New: Trap Density-VT"(w2341) -> ()
                n1333 = local write "Calc: Trap Density-VT"(w2341) -> ()
                n1334 = Increment(x=w2434) -> (x+1=w2435:i32)
                n1335 = Unbundle(w2423) -> (w2414:dbl[], w2413:dbl[])
                n1336 = Unbundle(w2411) -> (w2409:dbl[], w2408:dbl[])
                n1337 = Array Subset(array=w2414, index=w2371, length=w2391) -> (w2421:dbl[])
                n1338 = Array Subset(array=w2413, index=w2371, length=w2391) -> (w2420:dbl[])
                n1339 = Array Subset(array=w2409, index=w2389, length=w2390) -> (w2416:dbl[])
                n1340 = Array Subset(array=w2408, index=w2389, length=w2390) -> (w2415:dbl[])
                n1341 = Index Array(array=w2425, index=w2435) -> (element=w2430:string)
                n1342 = local write "Vg Array-Log-Used"(w2415) -> ()
                n1343 = local write "Sat Id-Log-Used"(w2416) -> ()
                n1344 = local write "Sat Id-Used"(w2420) -> ()
                n1345 = local write "Index"(w2430) -> ()
                n1346 = local write "Sat Vg Array-Used"(w2421) -> ()
                n1347 = while {
                  tunnel: w2432 -> [w2462]
                  tunnel: w2430 -> [w2460]
                  tunnel: [w2459] -> _
                  tunnel: [w2459] -> w2431
                  tunnel: w2418 -> [w2458]
                  i -> [w2459]
                  stop <- w2455 stop-if-true
                  n1348 = Index Array(array=w2462, index=w2459) -> (element=w2463:string)
                  n1349 = xnode "Match Regular Expression"("input string"=w2463, "regular expression"=w2460) -> ("whole match"=w2461:string)  [unwired: 4 in, 4 out]
                  n1350 = Equal?(x=w2461, y=w2460) -> (x = y?=w2457:bool)
                  n1351 = Equal?(x=w2458, y=w2459) -> (x = y?=w2456:bool)
                  n1352 = Or(x=w2457, y=w2456) -> (x .or. y?=w2455:bool)
                }
                n1353 = Path To String(path=w2427) -> (string=w2429:string)
                n1354 = Index Array(array=w2432, index=w2431) -> (element=w2406:string)
                n1355 = local write "Image Name"(w2406) -> ()
                n1356 = Empty String/Path?(string/path=w2406) -> (empty?=w2407:bool)
                n1357 = Concatenate Strings(w2429, "\\", w2406) -> (w2428:string)
                n1358 = String To Path(string=w2428) -> (path=w2405:path)
                n1359 = local read "No Image"() -> (w2404:path)
                n1360 = Select(t=w2404, s=w2407, f=w2405) -> (s? t:f=w2398:path)
                n1361 = local write "Image File"(w2398) -> ()
                n1362 = local read "Image Out"() -> (w2396:T2)
                n1363 = call "IMAQ ReadFile"("File Path"=w2398, "Image"=w2396) -> ("Image Out"=w2397:T2)  [unwired: 5 in, 4 out]
                n1364 = local write "Image Out"(w2397) -> ()
                n1365 = local write "Image Out 2"(w2397) -> ()
              }
              frame #4 {
                # "Output ROI data"
                n1366 = local read "Image Folder"() -> (w2578:path)
                n1367 = Build Path(base path=w2578, name or relative path="ROI") -> (appended path=w2580:path)
                n1368 = local read "Index"() -> (w2579:string)
                n1369 = Build Path(base path=w2580, name or relative path=w2579) -> (appended path=w2585:path)
                n1370 = invoke on="Image Out" class="ImageControl" method="Clear ROI"() -> (error out=w2584:errorcluster)  [unwired: 3 in, 2 out]
                n1371 = call <vilib>:"Check if File or Folder Exists.vi"("error in (no error)"=w2584, "path"=w2585) -> ("file or folder exists?"=w2582:bool, "dup path"=w2583:path)  [unwired: 7 in, 1 out]
                n1372 = case shown="True" w2582 {
                  tunnel: w2583 -> [_ w2586]
                  frame False {
                  }
                  frame True {
                    n1373 = Read from Text File(file (use dialog)=w2586) -> (text=w2590:string)  [unwired: 3 in, 3 out]
                    n1374 = property on="Image Out" class="ImageControl"() -> ("ROI"=w2587:T10)  [unwired: 2 in, 2 out]
                    n1375 = Unflatten From String(type=w2587, binary string=w2590) -> (value=w2588:T10, error out=w2589:errorcluster)  [unwired: 3 in, 1 out]
                    n1376 = property on="Image Out" class="ImageControl"(error in=w2589, "ROI"=w2588) -> ()  [unwired: 1 in, 2 out]
                  }
                }
              }
            }
            n1377 = flat-sequence {
              tunnel: [w2051] -> w2038
              tunnel: w2038 -> [w2065]
              frame #0 {
                # "Makes Empty File for Transformer Data"
                n1378 = local read "Data Folder"() -> (w2040:path)
                n1379 = Build Path(base path=w2040, name or relative path="Stats") -> (appended path=w2042:path)
                n1380 = call <vilib>:"Check if File or Folder Exists.vi"("path"=w2042) -> ("file or folder exists?"=w2043:bool, "dup path"=w2044:path)  [unwired: 8 in, 1 out]
                n1381 = case shown="False" w2043 {
                  tunnel: [w2048 w2050] -> w2045
                  tunnel: w2044 -> [w2049 w2050]
                  frame False {
                    n1382 = Create Folder(path (use dialog)=w2049) -> (created path=w2048:path)  [unwired: 2 in, 2 out]
                  }
                  frame True {
                  }
                }
                n1383 = Build Path(base path=w2045, name or relative path="Tranformer Data.txt") -> (appended path=w2047:path)
                n1384 = call-poly <vilib>:"Write To Spreadsheet File.vi"("append to file? (new file:F)"=TRUE, "file path (dialog if empty)"=w2047) -> ()  [unwired: 6 in, 1 out]
              }
              frame #1 {
                # "Adds Headers if they don't exist"
                n1385 = Concatenate Strings("Stats\\", "Tranformer Data.txt") -> (w2058:string)
                n1386 = local read "Data Folder"() -> (w2057:path)
                n1387 = Build Path(base path=w2057, name or relative path=w2058) -> (appended path=w2051:path)
                n1388 = call-poly <vilib>:"Read From Spreadsheet File.vi"("file path (dialog if empty)"=w2051) -> ("first row"=w2056:string[])  [unwired: 6 in, 4 out]
                n1389 = Search 1D Array(1D array=w2056, element="DeviceID") -> (index of element=w2054:i32)  [unwired: 1 in]
                n1390 = Equal?(x=w2054, y=0) -> (x = y?=w2052:bool)
                n1391 = case shown="False" w2052 {
                  tunnel: w2051 -> [w2062 _]
                  frame False {
                    n1392 = local read "Transformer \nHeaders"() -> (w2061:string[])
                    n1393 = call-poly <vilib>:"Write To Spreadsheet File.vi"("1D data"=w2061, "file path (dialog if empty)"=w2062) -> ()  [unwired: 6 in, 1 out]
                  }
                  frame True {
                  }
                }
              }
              frame #2 {
                # "Adds current device if it doesn't exist"
                n1394 = local read "Current \nRecord"() -> (w2068:string[])
                n1395 = Index Array(array=w2068, index=0) -> (element=w2067:string)
                n1396 = Concatenate Strings("Stats\\", "Tranformer Data.txt") -> (w2071:string)
                n1397 = local read "Data Folder"() -> (w2070:path)
                n1398 = local write "Current Device ID"(w2067) -> ()
                n1399 = local read "Current Device ID"() -> (w2077:string)
                n1400 = Build Path(base path=w2070, name or relative path=w2071) -> (appended path=w2069:path)
                n1401 = call-poly <vilib>:"Read From Spreadsheet File.vi"("file path (dialog if empty)"=w2069) -> ("all rows"=w2064:string[][])  [unwired: 6 in, 4 out]
                n1402 = Index Array(array=w2064, index (col)=0) -> (element=w2075:string[])  [unwired: 1 in]
                n1403 = Search 1D Array(1D array=w2075, element=w2077) -> (index of element=w2063:i32)  [unwired: 1 in]
                n1404 = Equal?(x=w2063, y=-1) -> (x = y?=w2066:bool)
                n1405 = case shown="False" w2066 {
                  tunnel: w2065 -> [w2079 w2092]
                  tunnel: w2063 -> [w2084 _]
                  tunnel: w2064 -> [w2085 _]
                  frame False {
                    n1406 = local read "Current \nRecord"() -> (w2083:string[])
                    n1407 = Replace Array Subset(array=w2085, new element=w2083, index (row)=w2084) -> (w2080:string[][])  [unwired: 1 in]
                    n1408 = flat-sequence {
                      tunnel: [w2086] -> _
                      tunnel: [w2087] -> _
                      tunnel: [w2087] -> w2082
                      tunnel: [w2086] -> w2081
                      tunnel: w2080 -> [w2087]
                      tunnel: w2079 -> [w2086]
                      tunnel: w2082 -> [w2089]
                      tunnel: w2081 -> [w2088]
                      frame #0 {
                        n1409 = Delete(path (use dialog)=w2086) -> ()  [unwired: 4 in, 3 out]
                      }
                      frame #1 {
                        n1410 = call-poly <vilib>:"Write To Spreadsheet File.vi"("append to file? (new file:F)"=TRUE, "2D data"=w2089, "file path (dialog if empty)"=w2088) -> ()  [unwired: 5 in, 1 out]
                      }
                    }
                  }
                  frame True {
                    n1411 = local read "Current \nRecord"() -> (w2091:string[])
                    n1412 = call-poly <vilib>:"Write To Spreadsheet File.vi"("append to file? (new file:F)"=TRUE, "1D data"=w2091, "file path (dialog if empty)"=w2092) -> ()  [unwired: 5 in, 1 out]
                  }
                }
              }
            }
          }
          event "Export": Mouse Down {
            n1413 = event-data() -> ()  [unwired: 1 in, 7 out]
            n1414 = local read "Data Folder"() -> (w2594:path)
            n1415 = Build Path(base path=w2594, name or relative path="Stats") -> (appended path=w2595:path)
            n1416 = call <vilib>:"Check if File or Folder Exists.vi"("path"=w2595) -> ("file or folder exists?"=w2611:bool, "dup path"=w2610:path)  [unwired: 8 in, 1 out]
            n1417 = local read "Project"() -> (w2607:path)
            n1418 = call <userlib>:"OA_ConnectToOrigin.vi"() -> ("error out"=w2608:errorcluster, "Origin.IOApplication"=w2609:refnum<k7>)  [unwired: 8 in]
            n1419 = case shown="False" w2611 {
              tunnel: w2610 -> [w2720 w2721]
              tunnel: [w2719 w2721] -> w2593
              frame False {
                n1420 = Create Folder(path (use dialog)=w2720) -> (created path=w2719:path)  [unwired: 2 in, 2 out]
              }
              frame True {
              }
            }
            n1421 = call <userlib>:"OA_Load.vi"("error in (no error)"=w2608, "Path"=w2607, "Origin.IOApplication"=w2609) -> ("error out"=w2605:errorcluster, "Origin.IOApplication"=w2606:refnum<k7>)  [unwired: 1 out]
            n1422 = call <userlib>:"OAExecute.vi"("script"="document -m 3;", "Error IO"=w2605, "Origin.IOApplication"=w2606) -> ("Error IO Out"=w2603:errorcluster, "Origin.IOApplication"=w2604:refnum<k7>)  [unwired: 1 in, 1 out]
            n1423 = stacked-sequence {
              tunnel: w2594 -> [w2623 w2626 w2639 w2652 w2665 w2678 w2692 w2706]
              tunnel: w2593 -> [w2622 w2627 w2640 w2653 w2666 w2679 w2691 w2707]
              tunnel: w2604 -> [w2619 w2629 w2642 w2655 w2668 w2681 w2694 w2709]
              tunnel: w2603 -> [w2621 w2628 w2641 w2654 w2667 w2680 w2693 w2708]
              tunnel: [_ _ _ _ _ _ _ w2704] -> w2592
              tunnel: [_ _ _ _ _ _ _ w2705] -> w2591
              frame #0 {
                n1424 = call "Param_Analysis_7_24b_JW.vi"("error in (no error)"=w2621, "Data Folder"=w2623, "Parameter String"="Mobility-Sat (cm^2/Vs):", "Parameter Name"="Mobility-Sat", "Stats Folder"=w2622) -> ("error out"=w2615:errorcluster, "Output Array"=w2613:string[][])  [unwired: 4 in, 1 out]
                n1425 = call "Origin_Export_7_24a_JW.vi"("Analysis Array"=w2613, "error in (no error)"=w2615, "Parameter Worksheet Name"="[MOBSvsLTable]Mobilities", "Parameter Folder Script"="pe_cd \"Mobility-Sat\";", "Origin.IOApplication"=w2619) -> ("error out"=w2614:errorcluster, "reference out"=w2616:refnum<k7>)  [unwired: 4 in, 1 out]
                n1426 = call <userlib>:"OAExecute.vi"("script"="window -a MOBSvsLTable;\nwindow -s TV;", "Error IO"=w2614, "Origin.IOApplication"=w2616) -> ()  [unwired: 1 in, 3 out]
              }
              frame #1 {
                n1427 = call "Param_Analysis_7_24b_JW.vi"("error in (no error)"=w2628, "Data Folder"=w2626, "Parameter String"="Mobility-Lin (cm^2/Vs):", "Parameter Name"="Mobility-Lin", "Stats Folder"=w2627) -> ("error out"=w2631:errorcluster, "Output Array"=w2633:string[][])  [unwired: 4 in, 1 out]
                n1428 = call "Origin_Export_7_24a_JW.vi"("Analysis Array"=w2633, "error in (no error)"=w2631, "Parameter Worksheet Name"="[MOBLvsLTable]Mobilities", "Parameter Folder Script"="pe_cd \"Mobility-Lin\";", "Origin.IOApplication"=w2629) -> ("error out"=w2630:errorcluster, "reference out"=w2632:refnum<k7>)  [unwired: 4 in, 1 out]
                n1429 = call <userlib>:"OAExecute.vi"("script"="window -a MOBLvsLTable;\nwindow -s TV;", "Error IO"=w2630, "Origin.IOApplication"=w2632) -> ()  [unwired: 1 in, 3 out]
              }
              frame #2 {
                n1430 = call "Param_Analysis_7_24b_JW.vi"("error in (no error)"=w2641, "Data Folder"=w2639, "Parameter String"="Off I-Sat (A):", "Parameter Name"="Off I-Sat", "Stats Folder"=w2640) -> ("error out"=w2645:errorcluster, "Output Array"=w2643:string[][])  [unwired: 4 in, 1 out]
                n1431 = call "Origin_Export_7_24a_JW.vi"("Analysis Array"=w2643, "error in (no error)"=w2645, "Parameter Worksheet Name"="[OffItable]OffCurrents", "Parameter Folder Script"="pe_cd \"Off I-Sat\";", "Origin.IOApplication"=w2642) -> ("error out"=w2644:errorcluster, "reference out"=w2646:refnum<k7>)  [unwired: 4 in, 1 out]
                n1432 = call <userlib>:"OAExecute.vi"("script"="window -a OffItable;\nwindow -s TV;", "Error IO"=w2644, "Origin.IOApplication"=w2646) -> ()  [unwired: 1 in, 3 out]
              }
              frame #3 {
                n1433 = call "Param_Analysis_7_24b_JW.vi"("error in (no error)"=w2654, "Data Folder"=w2652, "Parameter String"="On/Off I-Sat:", "Parameter Name"="OnOff Ratio", "Stats Folder"=w2653) -> ("error out"=w2658:errorcluster, "Output Array"=w2656:string[][])  [unwired: 4 in, 1 out]
                n1434 = call "Origin_Export_7_24a_JW.vi"("Analysis Array"=w2656, "error in (no error)"=w2658, "Parameter Worksheet Name"="[OnOffTable]On/Off Ratios", "Parameter Folder Script"="pe_cd \"On Off Ratio\";", "Origin.IOApplication"=w2655) -> ("error out"=w2657:errorcluster, "reference out"=w2659:refnum<k7>)  [unwired: 4 in, 1 out]
                n1435 = call <userlib>:"OAExecute.vi"("script"="window -a OnOffTable;\nwindow -s TV;", "Error IO"=w2657, "Origin.IOApplication"=w2659) -> ()  [unwired: 1 in, 3 out]
              }
              frame #4 {
                n1436 = call "Param_Analysis_7_24b_JW.vi"("error in (no error)"=w2667, "Data Folder"=w2665, "Parameter String"="STS-Sat (V/decade):", "Parameter Name"="STS-Sat", "Stats Folder"=w2666) -> ("error out"=w2671:errorcluster, "Output Array"=w2669:string[][])  [unwired: 4 in, 1 out]
                n1437 = call "Origin_Export_7_24a_JW.vi"("Analysis Array"=w2669, "error in (no error)"=w2671, "Parameter Worksheet Name"="[STable]Threshold Swing", "Parameter Folder Script"="pe_cd \"STS-Sat\";", "Origin.IOApplication"=w2668) -> ("error out"=w2670:errorcluster, "reference out"=w2672:refnum<k7>)  [unwired: 4 in, 1 out]
                n1438 = call <userlib>:"OAExecute.vi"("script"="window -a STable;\nwindow -s TV;", "Error IO"=w2670, "Origin.IOApplication"=w2672) -> ()  [unwired: 1 in, 3 out]
              }
              frame #5 {
                n1439 = call "Param_Analysis_7_24b_JW.vi"("error in (no error)"=w2680, "Data Folder"=w2678, "Parameter String"="Trap Density-STS (Traps/Vcm^2):", "Parameter Name"="Trap Density-STS", "Stats Folder"=w2679) -> ("error out"=w2684:errorcluster, "Output Array"=w2682:string[][])  [unwired: 4 in, 1 out]
                n1440 = call "Origin_Export_7_24a_JW.vi"("Analysis Array"=w2682, "error in (no error)"=w2684, "Parameter Worksheet Name"="[NSTSTable]Trap Densities", "Parameter Folder Script"="pe_cd \"Trap Density-STS\";", "Origin.IOApplication"=w2681) -> ("error out"=w2683:errorcluster, "reference out"=w2685:refnum<k7>)  [unwired: 4 in, 1 out]
                n1441 = call <userlib>:"OAExecute.vi"("script"="window -a NSTSTable;\nwindow -s TV;", "Error IO"=w2683, "Origin.IOApplication"=w2685) -> ()  [unwired: 1 in, 3 out]
              }
              frame #6 {
                n1442 = call "Param_Analysis_7_24b_JW.vi"("error in (no error)"=w2693, "Data Folder"=w2692, "Parameter String"="Trap Density-Vt (Traps/Vcm^2):", "Parameter Name"="Trap Density-Vt", "Stats Folder"=w2691) -> ("error out"=w2697:errorcluster, "Output Array"=w2695:string[][])  [unwired: 4 in, 1 out]
                n1443 = call "Origin_Export_7_24a_JW.vi"("Analysis Array"=w2695, "error in (no error)"=w2697, "Parameter Worksheet Name"="[NVTTable]Trap Densities", "Parameter Folder Script"="pe_cd \"Trap Density-Vt\";", "Origin.IOApplication"=w2694) -> ("error out"=w2696:errorcluster, "reference out"=w2698:refnum<k7>)  [unwired: 4 in, 1 out]
                n1444 = call <userlib>:"OAExecute.vi"("script"="window -a NVTTable;\nwindow -s TV;", "Error IO"=w2696, "Origin.IOApplication"=w2698) -> ()  [unwired: 1 in, 3 out]
              }
              frame #7 {
                n1445 = call "Param_Analysis_7_24b_JW.vi"("error in (no error)"=w2708, "Data Folder"=w2706, "Parameter String"="Vt-Sat (V):", "Parameter Name"="Vt-Sat", "Stats Folder"=w2707) -> ("error out"=w2712:errorcluster, "Output Array"=w2710:string[][])  [unwired: 4 in, 1 out]
                n1446 = call "Origin_Export_7_24a_JW.vi"("Analysis Array"=w2710, "error in (no error)"=w2712, "Parameter Worksheet Name"="[VtTable]Threshold Voltages", "Parameter Folder Script"="pe_cd \"Vt-Sat\";", "Origin.IOApplication"=w2709) -> ("error out"=w2711:errorcluster, "reference out"=w2713:refnum<k7>)  [unwired: 4 in, 1 out]
                n1447 = call <userlib>:"OAExecute.vi"("script"="window -a VtTable;\nwindow -s TV;", "Error IO"=w2711, "Origin.IOApplication"=w2713) -> ("Error IO Out"=w2704:errorcluster, "Origin.IOApplication"=w2705:refnum<k7>)  [unwired: 1 in, 1 out]
              }
            }
            n1448 = call "File Dialog"("start path"=w2595) -> ("selected path"=w2598:path)  [unwired: 11 in, 3 out]
            n1449 = Path To String(path=w2598) -> (string=w2597:string)
            n1450 = call <userlib>:"OAExecute.vi"("script"="pe_cd /; ", "Error IO"=w2592, "Origin.IOApplication"=w2591) -> ("Error IO Out"=w2599:errorcluster, "Origin.IOApplication"=w2600:refnum<k7>)  [unwired: 1 in, 1 out]
            n1451 = call <userlib>:"OASaveProject.vi"("path"=w2597, "Error IO"=w2599, "Origin.IOApplication"=w2600) -> ()  [unwired: 3 out]
          }
          event "Blank Button": Mouse Down {
            n1452 = event-data() -> ()  [unwired: 1 in, 7 out]
            n1453 = local read "Data File"() -> (w2729:path)
            n1454 = Strip Path(path=w2729) -> (stripped path=w2725:path, name=w2727:string)
            n1455 = Path To String(path=w2725) -> (string=w2724:string)
            n1456 = Concatenate Strings(w2724, "\\", "X_", w2727) -> (w2723:string)
            n1457 = String To Path(string=w2723) -> (path=w2722:path)
            n1458 = Move(source path=w2729, 10:w2722) -> ()  [unwired: 3 in, 3 out]
            n1459 = local write "Data File"(w2722) -> ()
          }
          event "Cancel Button": Mouse Down {
            (unwired) 6
            n1460 = event-data() -> ()  [unwired: 1 in, 7 out]
            n1461 = call "Simulate_Keyboard.vi"("Action"=2, "Virtual Key"=162) -> ()  [unwired: 7 in, 1 out]
          }
        }
        n1462 = Multiply(x=w522, y=10) -> (x*y=w524:sgl)
        n1463 = case shown="\"0\"" w563 {
          tunnel: w537 -> [w616 w622 w626 w628 w632 w634 w636 w638 w640 w642 w644 w646 w648 w650 w652 w654 w656 w658 w660 w662 w664 w666 w668 w670 w672 w674 w676 w678 w680 w682 w684 w686 w688 w690 w692 w694 w696 w698 w700 w702 w704 w706 w708 w710 w712 w714 w716 w718 w720 w722 w724 w726 w728 w730 w732 w734 w736 w738 w740 w742 w744 w746 w748 w750 w752 w754 w756 w758 w760 w762 w764 w766 w768 w770 w772 w774 w776 w778 w780 w782 w784 w786 w788 w790 w792 w794 w796 w798 w800 w802 w804 w806 w808 w810 w812 w814 w816 w818 w820 w822 w824 w826 w828 w830 w832]
          tunnel: [w616 w621 w625 w628 w632 w634 w636 w638 w640 w642 w644 w646 w648 w650 w652 w654 w656 w658 w660 w662 w664 w666 w668 w670 w672 w674 w676 w678 w680 w682 w684 w686 w688 w690 w692 w694 w696 w698 w700 w702 w704 w706 w708 w710 w712 w714 w716 w718 w720 w722 w724 w726 w728 w730 w732 w734 w736 w738 w740 w742 w744 w746 w748 w750 w752 w754 w756 w758 w760 w762 w764 w766 w768 w770 w772 w774 w776 w778 w780 w782 w784 w786 w788 w790 w792 w794 w796 w798 w800 w802 w804 w806 w808 w810 w812 w814 w816 w818 w820 w822 w824 w826 w828 w830 w832] -> w562
          tunnel: w538 -> [w618 w620 w624 w630 w631 w633 w635 w637 w639 w641 w643 w645 w647 w649 w651 w653 w655 w657 w659 w661 w663 w665 w667 w669 w671 w673 w675 w677 w679 w681 w683 w685 w687 w689 w691 w693 w695 w697 w699 w701 w703 w705 w707 w709 w711 w713 w715 w717 w719 w721 w723 w725 w727 w729 w731 w733 w735 w737 w739 w741 w743 w745 w747 w749 w751 w753 w755 w757 w759 w761 w763 w765 w767 w769 w771 w773 w775 w777 w779 w781 w783 w785 w787 w789 w791 w793 w795 w797 w799 w801 w803 w805 w807 w809 w811 w813 w815 w817 w819 w821 w823 w825 w827 w829 w831]
          tunnel: [w617 w620 w624 w629 w631 w633 w635 w637 w639 w641 w643 w645 w647 w649 w651 w653 w655 w657 w659 w661 w663 w665 w667 w669 w671 w673 w675 w677 w679 w681 w683 w685 w687 w689 w691 w693 w695 w697 w699 w701 w703 w705 w707 w709 w711 w713 w715 w717 w719 w721 w723 w725 w727 w729 w731 w733 w735 w737 w739 w741 w743 w745 w747 w749 w751 w753 w755 w757 w759 w761 w763 w765 w767 w769 w771 w773 w775 w777 w779 w781 w783 w785 w787 w789 w791 w793 w795 w797 w799 w801 w803 w805 w807 w809 w811 w813 w815 w817 w819 w821 w823 w825 w827 w829 w831] -> w561
          tunnel: w524 -> [w615 w619 w623 w627 _ _ _ _ _ _ _ _ _ _ _ _ _ _ _ _ _ _ _ _ _ _ _ _ _ _ _ _ _ _ _ _ _ _ _ _ _ _ _ _ _ _ _ _ _ _ _ _ _ _ _ _ _ _ _ _ _ _ _ _ _ _ _ _ _ _ _ _ _ _ _ _ _ _ _ _ _ _ _ _ _ _ _ _ _ _ _ _ _ _ _ _ _ _ _ _ _ _ _ _ _]
          frame "DOWN" {
            n1464 = Add(x=w618, y=w615) -> (x+y=w617:sgl)
          }
          frame "LEFT" {
            n1465 = Subtract(x=w622, y=w619) -> (x-y=w621:sgl)
          }
          frame "RIGHT" {
            n1466 = Add(x=w626, y=w623) -> (x+y=w625:sgl)
          }
          frame "UP" {
            n1467 = Subtract(x=w630, y=w627) -> (x-y=w629:sgl)
          }
          frame "ENTER (num pad)" {
          }
          frame "' (quote)" {
          }
          frame "END" {
          }
          frame "EQUALS" {
          }
          frame "ESCAPE" {
          }
          frame "GRAVE (`)" {
          }
          frame "HOME" {
          }
          frame "INSERT" {
          }
          frame "LBRACKET" {
          }
          frame "LCONTROL" {
          }
          frame "L ALT" {
          }
          frame "LSHIFT" {
          }
          frame "LWIN" {
          }
          frame "MINUS" {
          }
          frame "MULTIPLY" {
          }
          frame "NEXT" {
          }
          frame "NUMLOCK" {
          }
          frame "NUMPAD_0" {
          }
          frame "NUMPAD_1" {
          }
          frame "NUMPAD_2" {
          }
          frame "NUMPAD_3" {
          }
          frame "NUMPAD_4" {
          }
          frame "NUMPAD_5" {
          }
          frame "NUMPAD_6" {
          }
          frame "NUMPAD_7" {
          }
          frame "NUMPAD_8" {
          }
          frame "NUMPAD_9" {
          }
          frame "PAUSE" {
          }
          frame "PERIOD" {
          }
          frame "PRIOR (PG UP)" {
          }
          frame "RBRACKET" {
          }
          frame "RCONTROL" {
          }
          frame "RETURN" {
          }
          frame "R ALT" {
          }
          frame "RSHIFT" {
          }
          frame "RWIN" {
          }
          frame "SCROLL" {
          }
          frame "SEMICOLON" {
          }
          frame "SLASH" {
          }
          frame "SPACE" {
          }
          frame "SUBTRACT" {
          }
          frame "TAB" {
          }
          frame "DIVIDE" {
          }
          frame "DELETE" {
          }
          frame "DECIMAL" {
          }
          frame "COMMA" {
          }
          frame "CAPITAL" {
          }
          frame "BACKSLASH" {
          }
          frame "BACK" {
          }
          frame "ADD" {
          }
          frame "F15" {
          }
          frame "F14" {
          }
          frame "F13" {
          }
          frame "F12" {
          }
          frame "F11" {
          }
          frame "F10" {
          }
          frame "F9" {
          }
          frame "F8" {
          }
          frame "F7" {
          }
          frame "F6" {
          }
          frame "F5" {
          }
          frame "F4" {
          }
          frame "F3" {
          }
          frame "F2" {
          }
          frame "F1" {
          }
          frame "Z" {
          }
          frame "Y" {
          }
          frame "X" {
          }
          frame "W" {
          }
          frame "V" {
          }
          frame "U" {
          }
          frame "T" {
          }
          frame "S" {
          }
          frame "R" {
          }
          frame "Q" {
          }
          frame "P" {
          }
          frame "O" {
          }
          frame "N" {
          }
          frame "M" {
          }
          frame "L" {
          }
          frame "K" {
          }
          frame "J" {
          }
          frame "I" {
          }
          frame "H" {
          }
          frame "G" {
          }
          frame "F" {
          }
          frame "E" {
          }
          frame "D" {
          }
          frame "C" {
          }
          frame "B" {
          }
          frame "A" {
          }
          frame "9" {
          }
          frame "8" {
          }
          frame "7" {
          }
          frame "6" {
          }
          frame "5" {
          }
          frame "4" {
          }
          frame "3" {
          }
          frame "2" {
          }
          frame "1" {
          }
          frame "0" {
          }
        }
        n1468 = Bundle(w540, w539, w554, w553, 0.0) -> (w552:cluster{dbl, dbl, dbl, dbl, dbl})  [unwired: 1 in]
        n1469 = Bundle("X"=w562, "Y"=w561) -> (w556:cluster{"X":sgl, "Y":sgl})  [unwired: 1 in]
        n1470 = Divide(x=20, y=w523) -> (x/y=w526:sgl)
        n1471 = property on="Image Out" class="ImageControl"("Image Center Position"=w556) -> ()  [unwired: 2 in, 2 out]
        n1472 = call "IMAQ Convert Rectangle to ROI (Polygon)"("Rectangle"=w552) -> ("ROI Descriptor"=w550:T3)  [unwired: 7 in, 2 out]
        n1473 = Bundle("Application Font", w526, w530, w530, w530, w530, w530, TRUE, w528) -> (w532:T16)  [unwired: 1 in]
        n1474 = property on="Image Out 2" class="ImageControl"("ROI"=w550) -> ()  [unwired: 2 in, 2 out]
        n1475 = Bundle(w528, w532, w528, w528) -> (w531:T17)  [unwired: 1 in]
        n1476 = property on="Image Out" class="ImageControl"() -> ("ROI"=w515:T10)  [unwired: 2 in, 2 out]
        n1477 = Unbundle By Name(w515) -> ("Contours"=w579:T14)
        n1478 = local read "Image Out"() -> (w534:T2)
        n1479 = call "IMAQ Clear Overlay"("Image"=w534) -> ("Image Out"=w533:T2)  [unwired: 9 in, 1 out]
        n1480 = Initialize Array(0) -> (w577:i32[])  [unwired: 1 in]
        n1481 = local read "Magnification"() -> (w568:u16)
        n1482 = Array Size(array=w579) -> (size(s)=w578:i32)
        n1483 = Build Array(0.505025, 0.252522, 0.127742, 0.050345, 0.031129) -> (w569:dbl[])
        n1484 = Array Subset(array=w569, index=w568, length=1) -> (w566:dbl[])
        n1485 = property on="Image Out" class="ImageControl"() -> ("ZoomInteger"=w558:cluster{"X":i32, "Y":i32})  [unwired: 2 in, 2 out]
        n1486 = To Double Precision Float(number=w566) -> (double precision float=w565:dbl[])
        n1487 = for {
          N: w578 -> [_]
          shift-right: [w855] -> _
          shift-left: w579 -> [w855]
          shift-right: [w853] -> w564
          shift-left: w577 -> [w852]
          tunnel: w565 -> [w851]
          shift-right: [w848] -> _
          shift-left: w533 -> [w850]
          tunnel: w531 -> [w843]
          i -> [w847]
          n1488 = Index Array(array=w855, index=w847) -> (element=w864:T18)
          n1489 = Unbundle(w864) -> ("Points"=w863:i32[])  [unwired: 2 out]
          n1490 = Array To Cluster(array=w863) -> (cluster=w862:T19)
          n1491 = Unbundle(w862) -> ("Points[0]"=w842:i32, "Points[1]"=w839:i32, "Points[2]"=w854:i32, "Points[3]"=w860:i32)  [unwired: 5 out]
          n1492 = Add(x=w842, y=10) -> (x+y=w840:i32)
          n1493 = Subtract(x=w839, y=w860) -> (x-y=w859:i32)
          n1494 = Subtract(x=w842, y=w854) -> (x-y=w861:i32)
          n1495 = Square(x=w859) -> (x^2=w857:i32)
          n1496 = Square(x=w861) -> (x^2=w858:i32)
          n1497 = Add(x=w858, y=w857) -> (x+y=w856:i32)
          n1498 = Square Root(x=w856) -> (sqrt(x)=w833:dbl)
          n1499 = Multiply(x=w833, y=0.5) -> (x*y=w836:dbl)
          n1500 = Add(x=w836, y=w839) -> (x+y=w838:dbl)
          n1501 = Bundle(w840, w838) -> (w849:cluster{i32, dbl})  [unwired: 1 in]
          n1502 = Multiply(x=w833, y=w851) -> (x*y=w846:dbl[])
          n1503 = Index Array(array=w846) -> (element=w845:dbl)  [unwired: 1 in]
          n1504 = Number To Fractional String(number=w845) -> (F-format string=w844:string)  [unwired: 3 in]
          n1505 = call "IMAQ Overlay Text"("BG Color (Transparent)"=u32 0, "Text Color (black)"=u32 16448250, "Font, Size & Style"=w843, "String"=w844, "Origin"=w849, "Image"=w850) -> ("Image Out"=w848:T2)  [unwired: 4 in, 1 out]
          n1506 = Build Array (concatenate)(w852, w846) -> (w853:dbl[])
          n1507 = local write "Numeric 3"(w833) -> ()
        }
        n1508 = local write "ROI Descriptor"(w515) -> ()
        n1509 = Unbundle(w558) -> ("X"=w557:i32)  [unwired: 1 out]
        n1510 = Add Array Elements(numeric array=w564) -> (sum=w575:dbl)
        n1511 = local write "Distances"(w564) -> ()
        n1512 = local write "Total Width"(w575) -> ()
        n1513 = local write "Zoom"(w557) -> ()
        n1514 = local read "Manual-Width"() -> (w514:bool)
        n1515 = local read "Total Width"() -> (w518:dbl)
        n1516 = local read "Rec: Width"() -> (w516:dbl)
        n1517 = Not(x=w514) -> (.not. x?=w512:bool)
        n1518 = Equal To 0?(x=w518) -> (x = 0?=w513:bool)
        n1519 = Or(x=w513, y=w514) -> (x .or. y?=w517:bool)
        n1520 = And(x=w513, y=w512) -> (x .and. y?=w511:bool)
        n1521 = case shown="True" w511 {
          tunnel: w516 -> [_ w593]
          frame False {
          }
          frame True {
            n1522 = local write "New: Width"(w593) -> ()
          }
        }
        n1523 = case shown="False" w517 {
          tunnel: w518 -> [w594 _]
          frame False {
            n1524 = local write "New: Width"(w594) -> ()
          }
          frame True {
          }
        }
        n1525 = local read "Manuel-Dielectric"() -> (w440:bool)
        n1526 = local read "Rec: Dielectric (d)"() -> (w439:dbl)
        n1527 = local read "Manuel-Length"() -> (w441:bool)
        n1528 = local read "Rec: Length"() -> (w442:dbl)
        n1529 = case shown="False" w441 {
          tunnel: w442 -> [w584 _]
          frame False {
            n1530 = local write "New: Length"(w584) -> ()
          }
          frame True {
          }
        }
        n1531 = case shown="False" w440 {
          tunnel: w439 -> [w583 _]
          frame False {
            n1532 = local write "New: Dielectric"(w583) -> ()
          }
          frame True {
          }
        }
      }
    }
  }
  n1533 = Build Array("DeviceID", "Fabricator", "Deposition", "Date", "Sample", "Row", "Column", "L (um)", "W (um)", "Material", "Treatment", "TC (mM)", "Solvent", "C (%)", "ST (C)", "Drops", "Wait (s)", "RT (F)", "RH (%)", "Ramp (s)", "RPM", "Accel (RPM/s)", "Time (s)", "Mobility", "On/Off", "Vt", "S.T.S") -> (→"Transformer \nHeaders":string[])
